vi "AutoRun.vi"(11 "AllControls In":T1) -> ()   [LabVIEW 2017]
uses:
  Ctrls/AllControls.ctl
  Ctrls/Data.ctl
  Ctrls/CSV_Data.ctl
  0516/X682 Chassis Connectivity Tester Program/Ctrls/682_cmd.ctl
  <vilib>/Utility/miscctls.llb/LVRowAndColumnTypeDef.ctl
  Ctrls/AlarmIndex.ctl
  Ctrls/PathChoose.ctl
  ComVIS/Files/Ini/WriteIniFiles_ByVarient.vi
  <vilib>/Utility/file.llb/Write Delimited Spreadsheet (string).vi
  <vilib>/regexp/Match Regular Expression.xnode
  <instrlib>/GPP/GPP.lvlib
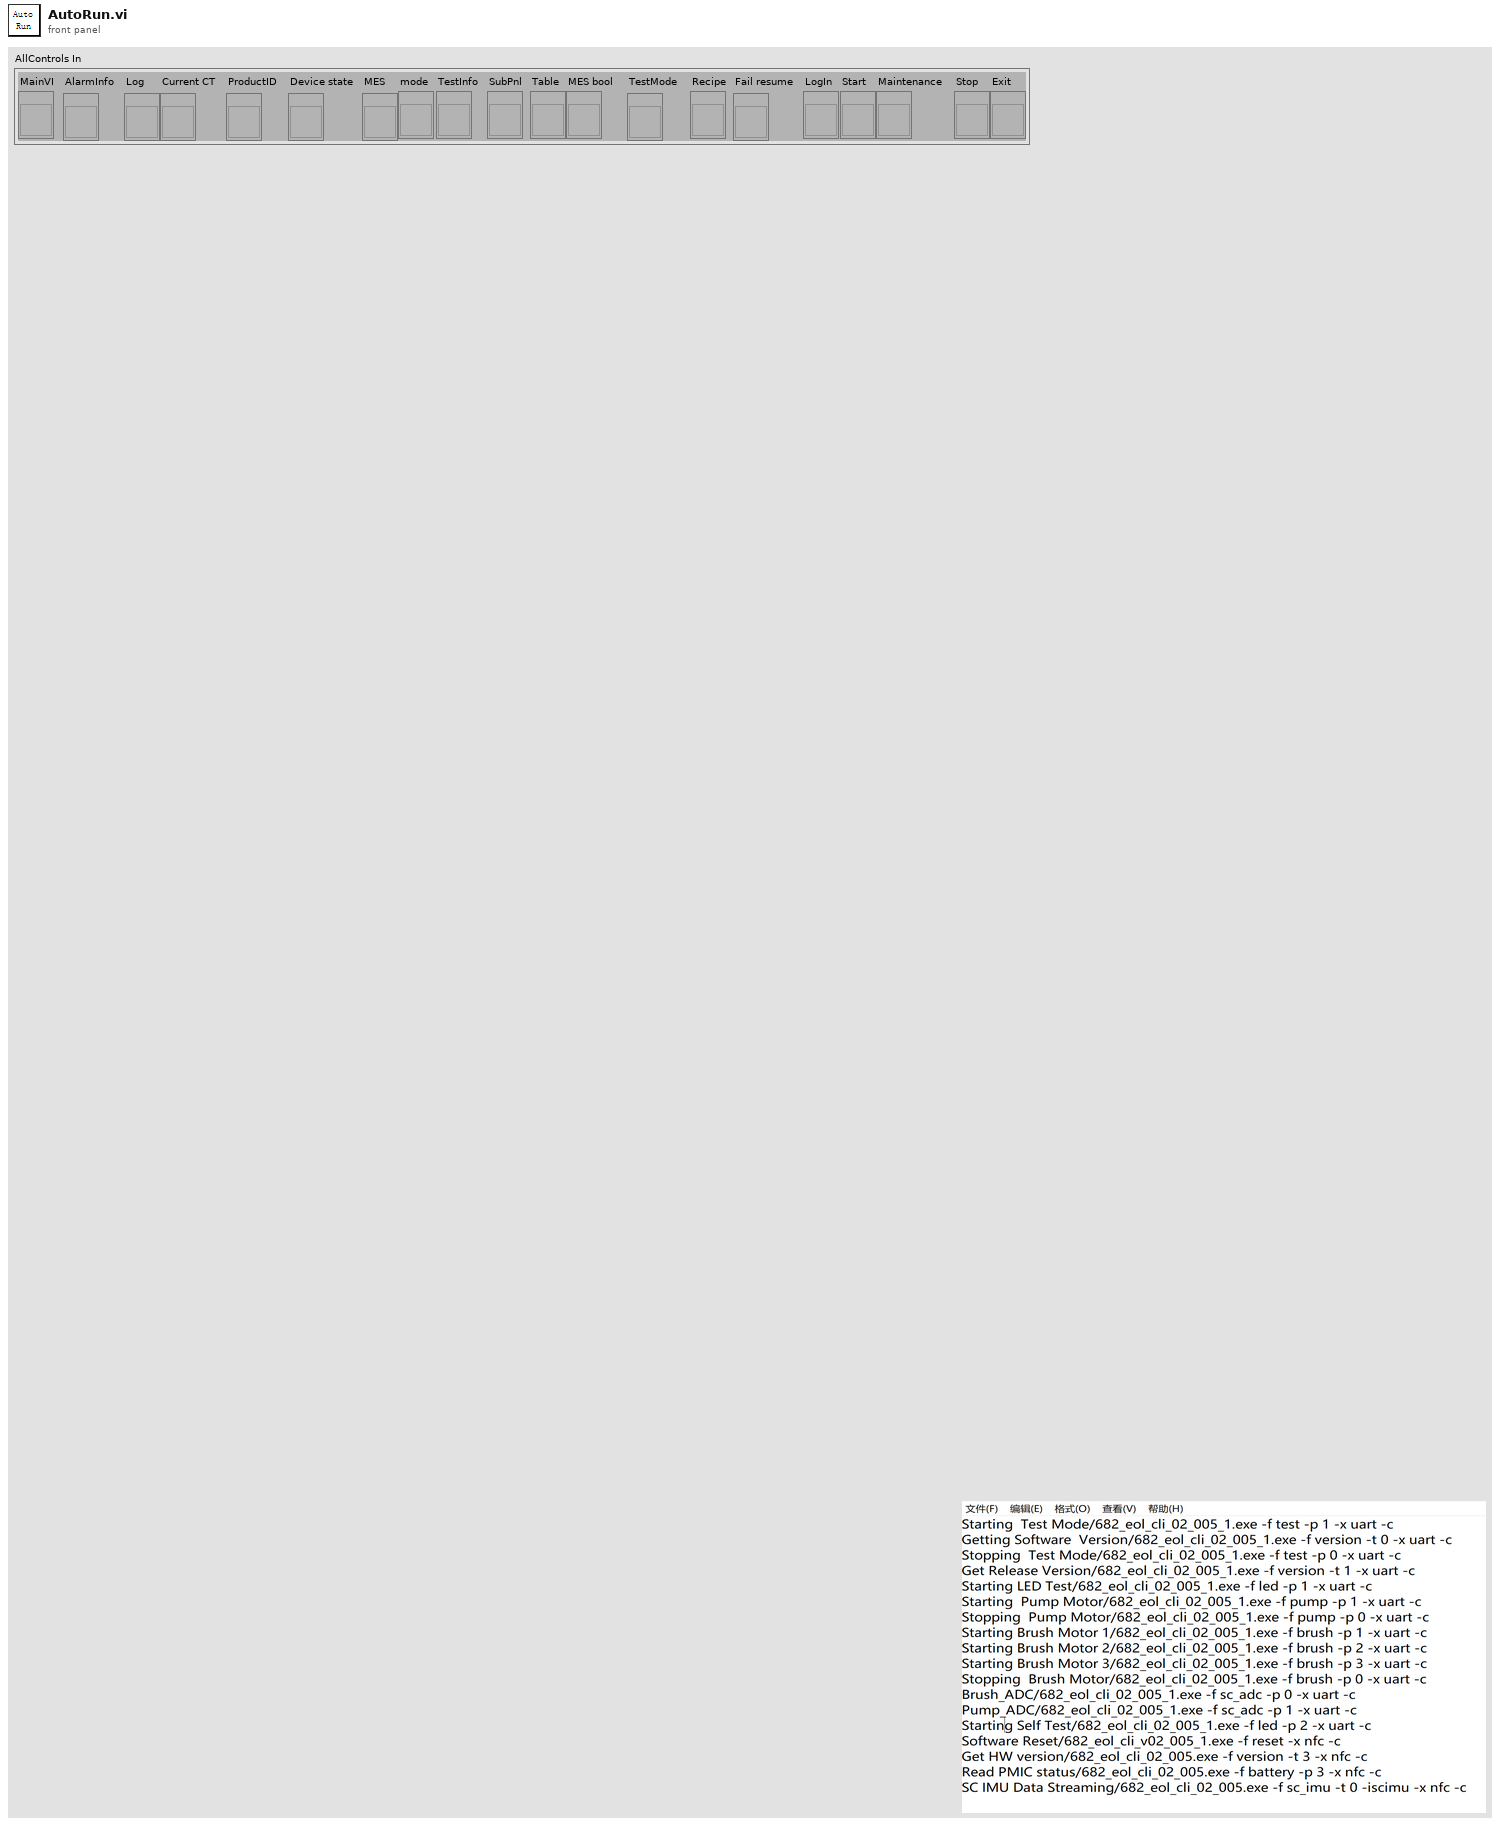
[diagram p1: front panel]
types:
  T1 = typedef "AllControls.ctl" = cluster{"MainVI":refnum<vi>, "AlarmInfo":refnum<vi>, "Log":refnum<vi>, "Current CT":refnum<vi>, "ProductID":refnum<vi>, "Device state":refnum<vi>, "MES":refnum<vi>, "mode":refnum<vi>, "TestInfo":refnum<vi>, "SubPnl":refnum<vi>, "Table":refnum<vi>, "MES bool":refnum<vi>, "TestMode":refnum<vi>, "Recipe":refnum<vi>, "Fail resume":refnum<vi>, "LogIn":refnum<vi>, "Start":refnum<vi>, "Maintenance":refnum<vi>, "Stop":refnum<vi>, "Exit":refnum<vi>}
  T2 = typedef "682_cmd.ctl" = cluster{"Brush_ADC.bat":string, "Get Release Version.bat":string, "Getting Software  Version.bat":string, "Pump_ADC.bat":string, "Starting  Pump Motor.bat":string, "Starting  Test Mode.bat":string, "Starting Brush Motor 1.bat":string, "Starting Brush Motor 2.bat":string, "Starting Brush Motor 3.bat":string, "Starting LED Test.bat":string, "Stopping  Brush Motor.bat":string, "Stopping  Pump Motor.bat":string, "Stopping  Test Mode.bat":string, "Starting Self Test.bat":string, "Software Reset.bat":string, "Get HW version.bat":string, "Read PMIC status.bat":string, "SC IMU Data Streaming.bat":string}
  T3 = typedef "CSV_Data.ctl" = cluster{"Initialisation":cluster{"LMT - Connect UUT (con COM)":string, "LMT - Software Version (rrel)":string, "LMT - Write SKU file (wskuc)":string, "LMT - SKU file name":string, "Connect UUT DDM":string, "Read DDM EOL Timestamp - Mode":string, "Read DDM EOL Timestamp - Timestamp":string, "Read DDM EOL Timestamp - Rig ID":string, "Read DDM EOL Timestamp - Passmark ID":string, "Read DDM EOL Timestamp - Passmark Rev":string, "Software Version before flashing":string, "Read Hardware Serial":string, "UUT DDM SN":string, "Compare DDM SN with MES SN":string, "Backup PCBA Calibration EEPROM Response - CAL":string, "Flash Firmware Version":string, "Check SW Version":string, "Read DDM SW Version after flashing":string, "Set SKU Config":string, "Ready Status":string, "Set Device Mode to EOL":string, "DDM Parameter - Voltage":string, "DDM Parameter - Current":string, "DDM Parameter - Power":string, "DDM Parameter - Speed":string, "DDM Parameter - Pressure":string, "Tester Parameter - Voltage":string, "Tester Parameter - Current":string, "Tester Parameter - Power":string, "Tester Parameter - Ambient Pressure":string, "Tester Parameter - Ambient Temperature":string, "Calculated Parameter - DDM Pressure Corrected":string, "Calculated Parameter - DDM Real Power":string, "Calculated Parameter - Delta V":string}, "BEMF_Calibration":cluster{"Calibration Result - eol_cold_bemf_temp":string, "DDM Ambient Temp":string, "Restriction Plate Diameter":string, "Calibration Result - eol_bemf_mp_cold_coef_a":string, "Calibration Result - eol_bemf_mp_cold_coef_b":string, "Calibration Result - eol_bemf_mp_cold_coef_c":string, "Calibration Result - eol_bemf_lsi_cold_ref_coeffs":string, "Get - Calibration Result - eol_bemf_lsi_speed":string, "Get - Calibration Result - eol_bemf_lsi_integral_0":string, "Calibration Result - eol_bemf_lsi_integral_1":string, "Get - Calibration Result - eol_bemf_lsi_integral_2":string, "Get - Calibration Result - eol_cold_bemf":string, "Get - Calibration Result - eol_cold_bemf_fisf":string, "Finalise Calibration":string, "Compare -Calibration Result - eol_cold_bemf":string, "Compare -Calibration Result - eol_cold_bemf_fisf":string}, "ECO":cluster{"Reset Power Tune":string, "Reset BEMF FISF Calibration":string, "Restriction Plate Diameter":string, "ECO - Stabilisation Time":string, "ECO - DDM Parameter - Voltage":string, "ECO - DDM Parameter - Current":string, "ECO - DDM Parameter - Power":string, "ECO - DDM Parameter - Measured Power":string, "ECO - DDM Parameter - Speed":string, "ECO - DDM Parameter - Pressure":string, "ECO - Tester Parameter - Voltage":string, "ECO - Tester Parameter - Current":string, "ECO - Tester Parameter - Power":string, "ECO - Tester Parameter - Ambient Pressure":string, "ECO - Tester Parameter - Ambient Temperature":string, "ECO - Tester Parameter - Ambient Humidity":string, "ECO - Calculated Parameter - DDM Pressure Corrected":string, "ECO - Calculated Parameter - DDM Real Power":string, "ECO - Calculated Parameter - Delta V":string, "ECO - Calculated Parameter - Flowrate":string, "ECO - Calculated Parameter - Airwatt":string, "ECO - Formula":string, "PT ECO - Power Tune Mode Status":string}, "BOOST":cluster{"Restriction Plate Diameter":string, "BOOST - Stabilisation Time":string, "BOOST - DDM Parameter - Voltage":string, "BOOST - DDM Parameter - Current":string, "BOOST - DDM Parameter - Power":string, "BOOST - DDM Parameter - Measured Power":string, "BOOST - DDM Parameter - Speed":string, "BOOST - DDM Parameter - Pressure":string, "BOOST - Tester Parameter - Voltage":string, "BOOST - Tester Parameter - Current":string, "BOOST - Tester Parameter - Power":string, "BOOST - Tester Parameter - Ambient Pressure":string, "BOOST - Tester Parameter - Ambient Temperature":string, "BOOST - Tester Parameter - Ambient Humidity":string, "BOOST - Calculated Parameter - DDM Pressure Corrected":string, "BOOST - Calculated Parameter - DDM Real Power":string, "BOOST - Calculated Parameter - Delta V":string, "BOOST - Calculated Parameter - Flowrate":string, "BOOST - Calculated Parameter - Airwatt":string, "BOOST - Get AM Presence":string, "Air Muscle Turn Off Status":string, "BOOST - Air Muscle Calculated Parameter - Airwatt B":string, "BOOST - Air Muscle Calculate Airwatt Delta":string, "PT BOOST - Power Tune Mode Status":string, "Finalise Calibration":string, "ECO - Get AW Calibration value":string, "BOOST - Get AW Calibration value":string}, "MAX":cluster{"Restriction Plate Diameter":string, "MAX - Stabilisation Time":string, "Get Average Delta Tmag (LSIdelta_FISFdelta_LSItmag_FISFtmag_IIRtmag)":string, "Get Average Delta Tmag FISF":string, "MAX - DDM Parameter - Voltage":string, "MAX - DDM Parameter - Current":string, "MAX - DDM Parameter - Power":string, "MAX - DDM Parameter - Measured Power":string, "MAX - DDM Parameter - Speed":string, "MAX - DDM Parameter - Pressure":string, "MAX - Tester Parameter - Voltage":string, "MAX - Tester Parameter - Current":string, "MAX - Tester Parameter - Power":string, "MAX - Tester Parameter - Ambient Pressure":string, "MAX - Tester Parameter - Ambient Temperature":string, "MAX - Tester Parameter - Ambient Humidity":string, "MAX - Calculated Parameter - DDM Pressure Corrected":string, "MAX - Calculated Parameter - DDM Real Power":string, "MAX - Calculated Parameter - Delta V":string, "MAX - Calculated Parameter - Flowrate":string, "MAX - Calculated Parameter - Airwatt":string, "MAX_FISF_Check_Average_Delta_Tmag":string, "MAX - FISF - BEMF Finetune Result":string, "MAX tune - Delta P1":string, "MAX tune - Calculated Parameter - Airwatt":string, "Calculate Delta Airwatts - MAX finetune - Delta P2":string, "MAX finetune - DDM Parameter - Voltage":string, "MAX finetune - DDM Parameter - Current":string, "MAX finetune - DDM Parameter - Power":string, "MAX finetune - DDM Parameter - Measured Power":string, "MAX finetune - DDM Parameter - Speed":string, "MAX finetune - DDM Parameter - Pressure":string, "MAX finetune - Tester Parameter - Voltage":string, "MAX finetune - Tester Parameter - Current":string, "MAX finetune - Tester Parameter - Power":string, "MAX finetune - Tester Parameter - Ambient Pressure":string, "MAX finetune - Tester Parameter - Ambient Temperature":string, "MAX finetune - Tester Parameter - Ambient Humidity":string, "MAX finetune - Calculated Parameter - DDM Pressure Corrected":string, "MAX finetune - Calculated Parameter - DDM Real Power":string, "MAX finetune - Calculated Parameter - Delta V":string, "MAX finetune - Calculated Parameter - Flowrate":string, "MAX finetune - Calculated Parameter - Airwatt":string, "Check Derate Result":string, "Delta Tmag FISF":string, "Get Hot BEMF Result":string, "Calculate delta Pressure":string, "Finalise Calibration":string, "Calculate & Check Delta BEMF":string, "Delta P Airwatts Value":string}, "LL":cluster{"DDM Ambient Temp":string, "Restriction Plate Diameter":string, "LL - DDM Parameter - Voltage":string, "LL - DDM Parameter - Current":string, "LL - DDM Parameter - Power":string, "LL - DDM Parameter - Measured Power":string, "LL - DDM Parameter - Speed":string, "LL - DDM Parameter - Pressure":string, "LL - Tester Parameter - Voltage":string, "LL - Tester Parameter - Current":string, "LL - Tester Parameter - Power":string, "LL - DDM Real Power":string, "LL - Calibrate Task Detect LL":string}, "HL":cluster{"HL - DDM Parameter - Voltage":string, "HL - DDM Parameter - Current":string, "HL - DDM Parameter - Power":string, "HL - DDM Parameter - Measured Power":string, "HL - DDM Parameter - Speed":string, "HL - DDM Parameter - Pressure":string, "HL - Tester Parameter - Voltage":string, "HL - Tester Parameter - Current":string, "HL - Tester Parameter - Power":string, "HL - DDM Real Power":string, "HL - Calibrate Task Detect HL":string}, "LH":cluster{"Restriction Plate Diameter":string, "LH - DDM Parameter - Voltage":string, "LH - DDM Parameter - Current":string, "LH - DDM Parameter - Power":string, "LH - DDM Parameter - Measured Power":string, "LH - DDM Parameter - Speed":string, "LH - DDM Parameter - Pressure":string, "LH - Tester Parameter - Voltage":string, "LH - Tester Parameter - Current":string, "LH - Tester Parameter - Power":string, "LH - DDM Real Power":string, "LH - Calibrate Task Detect LH":string}, "HH":cluster{"HH - DDM Parameter - Voltage":string, "HH - DDM Parameter - Current":string, "HH - DDM Parameter - Power":string, "HH - DDM Parameter - Measured Power":string, "HH - DDM Parameter - Speed":string, "HH - DDM Parameter - Pressure":string, "HH - Tester Parameter - Voltage":string, "HH - Tester Parameter - Current":string, "HH - Tester Parameter - Power":string, "HH - DDM Real Power":string, "HH - Calibrate Task Detect HH":string}, "Inlet Blockage Calibration":cluster{"Inlet Blockage Calibration - DDM Parameter - Voltage":string, "Inlet Blockage Calibration - DDM Parameter - Current":string, "Inlet Blockage Calibration - DDM Parameter - Power":string, "Inlet Blockage Calibration - DDM Parameter - Measured Power":string, "Inlet Blockage Calibration - DDM Parameter - Speed":string, "Inlet Blockage Calibration - DDM Parameter - Pressure":string, "Inlet Blockage Calibration - Tester Parameter - Voltage":string, "Inlet Blockage Calibration - Tester Parameter - Current":string, "Inlet Blockage Calibration - Tester Parameter - Power":string, "Inlet Blockage Calibration - DDM Real Power":string, "Calibration Inlet Blockage_E":string, "Finalise Calibration":string, "Get Task Detect LL":string, "Get Task Detect HL":string, "Get Task Detect LH":string, "Get Task Detect HH":string, "Calibration Inlet Blockage":string, "Calibration eol cold bemf temp":string}, "GOOD":cluster{"GOOD UNIT - Clear EEPROM Error Log":string, "GOOD UNIT - Write Product Timestamp - Mode":string, "GOOD UNIT - Write Product Timestamp - Timestamp":string, "GOOD UNIT - Write Product Timestamp - Rig ID":string, "GOOD UNIT - Write Product Timestamp - Passmark ID":string, "GOOD UNIT - Write Product Timestamp - Passmark Rev":string, "GOOD UNIT - Set Device Mode to PROD":string, "GOOD UNIT - Backup PCBA Calibration EEPROM Response":string, "GOOD UNIT - Check Security Bit":string, "GOOD UNIT - Set Calibration Lock":string, "GOOD UNIT - Get_Calibration_Lock":string, "GOOD UNIT - Disconnect UUT":string}, "NG":cluster{"NG UNIT - Read NVM Error":string, "NG UNIT - Set Device Mode to FCT":string, "NG UNIT - Backup PCBA Calibration EEPROM Response - CAL":string, "NG UNIT - Backup PCBA Calibration EEPROM Response - ERROR":string, "NG UNIT - Backup PCBA Calibration EEPROM Response - USAGE":string, "NG UNIT - Disconnect UUT":string}, "SN":string, "Table":string[][], "Count":cluster{"Total":i32, "OK":i32, "NG":i32, "Yield":dbl}, "Start Time":timestamp, "daemon reference":refnum<k5>, "CT":dbl, "Config":string[][], "OK/NG":bool, "Station ID":string, "MES DDM SN":string, "MES PCBA SN":string, "Retest":string, "Lux":string, "Initialisation_Status":cluster{"LMT - Connect UUT (con COM)":string, "LMT - Software Version (rrel)":string, "LMT - Write SKU file (wskuc)":string, "LMT - SKU file name":string, "Connect UUT DDM":string, "Read DDM EOL Timestamp - Mode":string, "Read DDM EOL Timestamp - Timestamp":string, "Read DDM EOL Timestamp - Rig ID":string, "Read DDM EOL Timestamp - Passmark ID":string, "Read DDM EOL Timestamp - Passmark Rev":string, "Software Version before flashing":string, "Read Hardware Serial":string, "UUT DDM SN":string, "Compare DDM SN with MES SN":string, "Backup PCBA Calibration EEPROM Response - CAL":string, "Flash Firmware Version":string, "Check SW Version":string, "Read DDM SW Version after flashing":string, "Set SKU Config":string, "Ready Status":string, "Set Device Mode to EOL":string, "DDM Parameter - Voltage":string, "DDM Parameter - Current":string, "DDM Parameter - Power":string, "DDM Parameter - Speed":string, "DDM Parameter - Pressure":string, "Tester Parameter - Voltage":string, "Tester Parameter - Current":string, "Tester Parameter - Power":string, "Tester Parameter - Ambient Pressure":string, "Tester Parameter - Ambient Temperature":string, "Calculated Parameter - DDM Pressure Corrected":string, "Calculated Parameter - DDM Real Power":string, "Calculated Parameter - Delta V":string}, "BEMF_Calibration_Status":cluster{"Calibration Result - eol_cold_bemf_temp":string, "DDM Ambient Temp":string, "Restriction Plate Diameter":string, "Calibration Result - eol_bemf_mp_cold_coef_a":string, "Calibration Result - eol_bemf_mp_cold_coef_b":string, "Calibration Result - eol_bemf_mp_cold_coef_c":string, "Calibration Result - eol_bemf_lsi_cold_ref_coeffs":string, "Get - Calibration Result - eol_bemf_lsi_speed":string, "Get - Calibration Result - eol_bemf_lsi_integral_0":string, "Calibration Result - eol_bemf_lsi_integral_1":string, "Get - Calibration Result - eol_bemf_lsi_integral_2":string, "Get - Calibration Result - eol_cold_bemf":string, "Get - Calibration Result - eol_cold_bemf_fisf":string, "Finalise Calibration":string, "Compare -Calibration Result - eol_cold_bemf":string, "Compare -Calibration Result - eol_cold_bemf_fisf":string}, "ECO_Status":cluster{"Reset Power Tune":string, "Reset BEMF FISF Calibration":string, "Restriction Plate Diameter":string, "ECO - Stabilisation Time":string, "ECO - DDM Parameter - Voltage":string, "ECO - DDM Parameter - Current":string, "ECO - DDM Parameter - Power":string, "ECO - DDM Parameter - Measured Power":string, "ECO - DDM Parameter - Speed":string, "ECO - DDM Parameter - Pressure":string, "ECO - Tester Parameter - Voltage":string, "ECO - Tester Parameter - Current":string, "ECO - Tester Parameter - Power":string, "ECO - Tester Parameter - Ambient Pressure":string, "ECO - Tester Parameter - Ambient Temperature":string, "ECO - Tester Parameter - Ambient Humidity":string, "ECO - Calculated Parameter - DDM Pressure Corrected":string, "ECO - Calculated Parameter - DDM Real Power":string, "ECO - Calculated Parameter - Delta V":string, "ECO - Calculated Parameter - Flowrate":string, "ECO - Calculated Parameter - Airwatt":string, "ECO - Formula":string, "PT ECO - Power Tune Mode Status":string}, "BOOST_Status":cluster{"Restriction Plate Diameter":string, "BOOST - Stabilisation Time":string, "BOOST - DDM Parameter - Voltage":string, "BOOST - DDM Parameter - Current":string, "BOOST - DDM Parameter - Power":string, "BOOST - DDM Parameter - Measured Power":string, "BOOST - DDM Parameter - Speed":string, "BOOST - DDM Parameter - Pressure":string, "BOOST - Tester Parameter - Voltage":string, "BOOST - Tester Parameter - Current":string, "BOOST - Tester Parameter - Power":string, "BOOST - Tester Parameter - Ambient Pressure":string, "BOOST - Tester Parameter - Ambient Temperature":string, "BOOST - Tester Parameter - Ambient Humidity":string, "BOOST - Calculated Parameter - DDM Pressure Corrected":string, "BOOST - Calculated Parameter - DDM Real Power":string, "BOOST - Calculated Parameter - Delta V":string, "BOOST - Calculated Parameter - Flowrate":string, "BOOST - Calculated Parameter - Airwatt":string, "BOOST - Get AM Presence":string, "Air Muscle Turn Off Status":string, "BOOST - Air Muscle Calculated Parameter - Airwatt B":string, "BOOST - Air Muscle Calculate Airwatt Delta":string, "PT BOOST - Power Tune Mode Status":string, "Finalise Calibration":string, "ECO - Get AW Calibration value":string, "BOOST - Get AW Calibration value":string}, "MAX_Status":cluster{"Restriction Plate Diameter":string, "MAX - Stabilisation Time":string, "Get Average Delta Tmag (LSIdelta_FISFdelta_LSItmag_FISFtmag_IIRtmag)":string, "Get Average Delta Tmag FISF":string, "MAX - DDM Parameter - Voltage":string, "MAX - DDM Parameter - Current":string, "MAX - DDM Parameter - Power":string, "MAX - DDM Parameter - Measured Power":string, "MAX - DDM Parameter - Speed":string, "MAX - DDM Parameter - Pressure":string, "MAX - Tester Parameter - Voltage":string, "MAX - Tester Parameter - Current":string, "MAX - Tester Parameter - Power":string, "MAX - Tester Parameter - Ambient Pressure":string, "MAX - Tester Parameter - Ambient Temperature":string, "MAX - Tester Parameter - Ambient Humidity":string, "MAX - Calculated Parameter - DDM Pressure Corrected":string, "MAX - Calculated Parameter - DDM Real Power":string, "MAX - Calculated Parameter - Delta V":string, "MAX - Calculated Parameter - Flowrate":string, "MAX - Calculated Parameter - Airwatt":string, "MAX_FISF_Check_Average_Delta_Tmag":string, "MAX - FISF - BEMF Finetune Result":string, "MAX tune - Delta P1":string, "MAX tune - Calculated Parameter - Airwatt":string, "Calculate Delta Airwatts - MAX finetune - Delta P2":string, "MAX finetune - DDM Parameter - Voltage":string, "MAX finetune - DDM Parameter - Current":string, "MAX finetune - DDM Parameter - Power":string, "MAX finetune - DDM Parameter - Measured Power":string, "MAX finetune - DDM Parameter - Speed":string, "MAX finetune - DDM Parameter - Pressure":string, "MAX finetune - Tester Parameter - Voltage":string, "MAX finetune - Tester Parameter - Current":string, "MAX finetune - Tester Parameter - Power":string, "MAX finetune - Tester Parameter - Ambient Pressure":string, "MAX finetune - Tester Parameter - Ambient Temperature":string, "MAX finetune - Tester Parameter - Ambient Humidity":string, "MAX finetune - Calculated Parameter - DDM Pressure Corrected":string, "MAX finetune - Calculated Parameter - DDM Real Power":string, "MAX finetune - Calculated Parameter - Delta V":string, "MAX finetune - Calculated Parameter - Flowrate":string, "MAX finetune - Calculated Parameter - Airwatt":string, "Check Derate Result":string, "Delta Tmag FISF":string, "Get Hot BEMF Result":string, "Calculate delta Pressure":string, "Finalise Calibration":string, "Calculate & Check Delta BEMF":string, "Delta P Airwatts Value":string}, "LL_Status":cluster{"DDM Ambient Temp":string, "Restriction Plate Diameter":string, "LL - DDM Parameter - Voltage":string, "LL - DDM Parameter - Current":string, "LL - DDM Parameter - Power":string, "LL - DDM Parameter - Measured Power":string, "LL - DDM Parameter - Speed":string, "LL - DDM Parameter - Pressure":string, "LL - Tester Parameter - Voltage":string, "LL - Tester Parameter - Current":string, "LL - Tester Parameter - Power":string, "LL - DDM Real Power":string, "LL - Calibrate Task Detect LL":string}, "HL_Status":cluster{"HL - DDM Parameter - Voltage":string, "HL - DDM Parameter - Current":string, "HL - DDM Parameter - Power":string, "HL - DDM Parameter - Measured Power":string, "HL - DDM Parameter - Speed":string, "HL - DDM Parameter - Pressure":string, "HL - Tester Parameter - Voltage":string, "HL - Tester Parameter - Current":string, "HL - Tester Parameter - Power":string, "HL - DDM Real Power":string, "HL - Calibrate Task Detect HL":string}, "LH_Status":cluster{"Restriction Plate Diameter":string, "LH - DDM Parameter - Voltage":string, "LH - DDM Parameter - Current":string, "LH - DDM Parameter - Power":string, "LH - DDM Parameter - Measured Power":string, "LH - DDM Parameter - Speed":string, "LH - DDM Parameter - Pressure":string, "LH - Tester Parameter - Voltage":string, "LH - Tester Parameter - Current":string, "LH - Tester Parameter - Power":string, "LH - DDM Real Power":string, "LH - Calibrate Task Detect LH":string}, "HH_Status":cluster{"HH - DDM Parameter - Voltage":string, "HH - DDM Parameter - Current":string, "HH - DDM Parameter - Power":string, "HH - DDM Parameter - Measured Power":string, "HH - DDM Parameter - Speed":string, "HH - DDM Parameter - Pressure":string, "HH - Tester Parameter - Voltage":string, "HH - Tester Parameter - Current":string, "HH - Tester Parameter - Power":string, "HH - DDM Real Power":string, "HH - Calibrate Task Detect HH":string}, "Inlet Blockage Calibration_Status":cluster{"Inlet Blockage Calibration - DDM Parameter - Voltage":string, "Inlet Blockage Calibration - DDM Parameter - Current":string, "Inlet Blockage Calibration - DDM Parameter - Power":string, "Inlet Blockage Calibration - DDM Parameter - Measured Power":string, "Inlet Blockage Calibration - DDM Parameter - Speed":string, "Inlet Blockage Calibration - DDM Parameter - Pressure":string, "Inlet Blockage Calibration - Tester Parameter - Voltage":string, "Inlet Blockage Calibration - Tester Parameter - Current":string, "Inlet Blockage Calibration - Tester Parameter - Power":string, "Inlet Blockage Calibration - DDM Real Power":string, "Calibration Inlet Blockage_E":string, "Finalise Calibration":string, "Get Task Detect LL":string, "Get Task Detect HL":string, "Get Task Detect LH":string, "Get Task Detect HH":string, "Calibration Inlet Blockage":string, "Calibration eol cold bemf temp":string}, "GOOD_Status":cluster{"GOOD UNIT - Clear EEPROM Error Log":string, "GOOD UNIT - Write Product Timestamp - Mode":string, "GOOD UNIT - Write Product Timestamp - Timestamp":string, "GOOD UNIT - Write Product Timestamp - Rig ID":string, "GOOD UNIT - Write Product Timestamp - Passmark ID":string, "GOOD UNIT - Write Product Timestamp - Passmark Rev":string, "GOOD UNIT - Set Device Mode to PROD":string, "GOOD UNIT - Backup PCBA Calibration EEPROM Response":string, "GOOD UNIT - Check Security Bit":string, "GOOD UNIT - Set Calibration Lock":string, "GOOD UNIT - Get_Calibration_Lock":string, "GOOD UNIT - Disconnect UUT":string}, "NG_Status":cluster{"NG UNIT - Read NVM Error":string, "NG UNIT - Set Device Mode to FCT":string, "NG UNIT - Backup PCBA Calibration EEPROM Response - CAL":string, "NG UNIT - Backup PCBA Calibration EEPROM Response - ERROR":string, "NG UNIT - Backup PCBA Calibration EEPROM Response - USAGE":string, "NG UNIT - Disconnect UUT":string}, "SKU":string, "Plate_Diameter":string, "Alarm":string}
  T4 = typedef "Data.ctl" = cluster{"Initialisation":cluster{"DDM_Parameter":dbl[], "DDM_Parameter_status":bool[], "Get_Tester_Parameter":dbl[], "Get_Tester_Parameter_status":bool[], "Cal_Tester_Parameter":dbl[], "Cal_Tester_Parameter_status":bool[], "sw_version_before_status":bool, "sw_version_after_status":bool, "Set_SKU_Config_With_LMT_status":bool, "FCT_timestamp_status":bool, "LMT_Connect_to_UUT_status":bool}, "BEMF_Calibration":cluster{"Read_ambient_temperature":dbl, "Calibration_Vaule":dbl[], "Calibration_Vaule _B":dbl[], "Calibration_Vaule_status":bool[], "Calibration_Vaule_B_status":bool[]}, "ECO":cluster{"DDM_Parameter":dbl[], "DDM_Parameter_status":bool[], "Get_Tester_Parameter":dbl[], "Get_Tester_Parameter_status":bool[], "Cal_Tester_Parameter":dbl[], "Cal_Tester_Parameter_status":bool[], "DDM_Parameter_after_power_tune":dbl[], "Get_Tester_Parameter_after_power_tune":dbl[], "Cal_Tester_Parameter_after_power_tune":dbl[], "Cal_Tester_Parameter_after_power_tune_status":bool[], "Delta_P":dbl}, "BOOST":cluster{"DDM_Parameter":dbl[], "DDM_Parameter_status":bool[], "Get_Tester_Parameter":dbl[], "Get_Tester_Parameter_status":bool[], "Cal_Tester_Parameter":dbl[], "Cal_Tester_Parameter_status":bool[], "DDM_Parameter_after_power_tune":dbl[], "Get_Tester_Parameter_after_power_tune":dbl[], "Cal_Tester_Parameter_after_power_tune":dbl[], "Cal_Tester_Parameter_after_power_tune_status":bool[], "airwatts_am_off":dbl, "AW_Delta_(AM_on_and_off)":dbl, "AW_Delta_(AM_on_and_off)_Status":bool, "Delta_P":dbl}, "MAX":cluster{"Average_Tmag_Data":cluster{"LSI Delta in degC":dbl, "FISF Delta in degc":dbl, "LSI Tmag in degC":dbl, "Fisf Tmag in degC":dbl, "IIR Tmag in degC":dbl}, "DDM_Parameter":dbl[], "DDM_Parameter_status":bool[], "Get_Tester_Parameter":dbl[], "Get_Tester_Parameter_status":bool[], "Cal_Tester_Parameter":dbl[], "BEMF_Finetune":cluster{"eol_bemf_mp_cold_coef_c":dbl, "eol_cold_bemf_fisf_offset":dbl}, "AW_Tune":cluster{"delta_P1":dbl, "delta_P_Setting":dbl}, "DDM_Parameter_after_Airwatts_Tune":dbl[], "Get_Tester_Parameter_after_Airwatts_Tune":dbl[], "Cal_Tester_Parameter_after_Airwatts_Tune":dbl[], "DDM_Parameter_after_Airwatts_Finetune":dbl[], "Get_Tester_Parameter_after_Airwatts_Finetune":dbl[], "Cal_Tester_Parameter_after_Airwatts_Finetune":dbl[], "AW_Finetune":cluster{"delta_P2":dbl, "delta_P_Setting":dbl}, "Delta_Tmag_after_tune":cluster{"LSI Delta in degC":dbl, "FISF Delta in degc":dbl, "LSI Tmag in degC":dbl, "Fisf Tmag in degC":dbl, "IIR Tmag in degC":dbl}, "Hot Bemf in mV":dbl, "DDM_Pressure":dbl, "Delta_Pressure":dbl, " Cold Bemf in mV":dbl, " delta Bemf":dbl, " delta p":dbl, "Delta_Pressure_status":bool, " delta Bemf_status":bool, "LSI Delta in degC_status":bool, "FISF Delta in degc_status":bool, "Max_check_derate_status_status":bool, "Average_All_data":dbl[][], "Average_Tmag_Data_status":bool[], "Average_Tmag_Data_after_tune_status":bool[], "Cal_Tester_Parameter_status":bool[], "Cal_Tester_Parameter_status_after_Airwatts_Tune":bool[], "Cal_Tester_Parameter_status_after_Airwatts_FineTune":bool[]}, "Task_Detect_Calib":cluster{"LL":cluster{"DDM_Parameter":dbl[], "DDM_Parameter_status":bool[], "Get_Tester_Parameter":dbl[], "Get_Tester_Parameter_status":bool[], "Set_task_detect_A":dbl, "Set_task_detect_A_Status":bool}, "HL":cluster{"DDM_Parameter":dbl[], "DDM_Parameter_status":bool[], "Get_Tester_Parameter":dbl[], "Get_Tester_Parameter_status":bool[], "Set_task_detect_B":dbl, "Set_task_detect_B_Status":bool}, "LH":cluster{"DDM_Parameter":dbl[], "DDM_Parameter_status":bool[], "Get_Tester_Parameter":dbl[], "Get_Tester_Parameter_status":bool[], "Set_task_detect_C":dbl, "Set_task_detect_C_Status":bool}, "HH":cluster{"DDM_Parameter":dbl[], "DDM_Parameter_status":bool[], "Get_Tester_Parameter":dbl[], "Get_Tester_Parameter_status":bool[], "Set_task_detect_D":dbl, "Read_and_check_calibration_Status":bool[], "Set_task_detect_D_Status":bool}, "Get_eol_inlet_blockage_E":dbl, "Calib_vaule":cluster{"Get_task_detect_LL":dbl, "Get_task_detect_HL":dbl, "Get_task_detect_LH":dbl, "Get_task_detect_HH":dbl, "eol_inlet_blockage":dbl, "eol_code_bemf_temp":dbl}, "calibrated temp":dbl, "Inlet_Blockage_Calibration":cluster{"DDM_Parameter":dbl[], "DDM_Parameter_status":bool[], "Get_Tester_Parameter":dbl[], "Get_Tester_Parameter_status":bool[]}, "Get_eol_inlet_blockage_E_Status":bool}, "good":cluster{"Write_Product_TS":cluster{"TIMESTAMP":i64, "RIG_ID":i64, "PASSMARK_ID":i64, "PASSMARK_REV":i64}, "Read_Product_TS":cluster{"TIMESTAMP":i64, "RIG_ID":i64, "PASSMARK_ID":i64, "PASSMARK_REV":i64}, "Good_Check_Secuity_Bit_Stauts":bool}}
  T5 = typedef "amc_Message Queue.ctl" = refnum<queue>
  T6 = typedef "TesterInfo.ctl" = cluster{"Station Name":string, "Station Code":string, "ES NO.":string, "Tester ID":string, "PassMark Revision":string, "Rig ID":string, "Deamon_vision":string, "Project Name":string, "FFTesterPath":path, "Enable_User":bool, "Mode":enum16{"682"}, "MES":bool}
  T7 = cluster{"Total":i32, "OK":i32, "NG":i32, "Yield":dbl}
  T8 = typedef "LVRowAndColumnTypeDef.ctl" = cluster{"Row":i32, "Column":i32}
  T9 = enum8{"Enabled", "Disabled", "Disabled and Grayed Out"}
  T10 = typedef "AlarmIndex.ctl" = enum16{"E-Stop", "Safety light grid", "UUT Sealing Cylinder HomePoint", "UUT Sealing Cylinder WorkPoint", "Orifice fixed Cylinder L HomePoint", "Orifice fixed Cylinder L WorkPoint", "Orifice fixed Cylinder R HomePoint", "Orifice fixed Cylinder R WorkPoint", "UUT Cylinder HomePoint", "UUT Cylinder WorkPoint", "Carrier fixed Cylinder L HomePoint", "Carrier fixed Cylinder L WorkPoint", "Carrier fixed Cylinder R HomePoint", "Carrier fixed Cylinder R WorkPoint", "Probe Cylinder HomePoint", "Probe Cylinder WorkPoint", "Motor Error", "Test Error"}
  T11 = typedef "PathChoose.ctl" = enum16{"OperatorLog", "AutoRunLog", "AlmLog", "TestData", "AllTestData", "backup_nvm", "backup_before_flashing"}
  T12 = typedef "HD Config.ctl" = cluster{" PC":cluster{"PC Address":u8[], "PC Port":i32}, "FCO":cluster{"COM":refnum<visa-resource-name>, "Baudrate":u32}, "DC Power ":cluster{"COM":refnum<visa-resource-name>, "Baudrate":u32}, "PW3336":cluster{"COM":refnum<visa-resource-name>, "Baudrate":u32}, "Lefoo":cluster{"COM":refnum<visa-resource-name>, "Baudrate":u32}, "Tempt&Hum":cluster{"COM":refnum<visa-resource-name>, "Baudrate":u32}, "DIPC":cluster{"COM":refnum<visa-resource-name>}, "Daemon":cluster{"IP Address":string, "Port":u16, "Retry":u16}, "URAT":cluster{"COM":refnum<visa-resource-name>, "Baudrate":u32}, "Fail_resume_mode":bool, "GRR":bool}
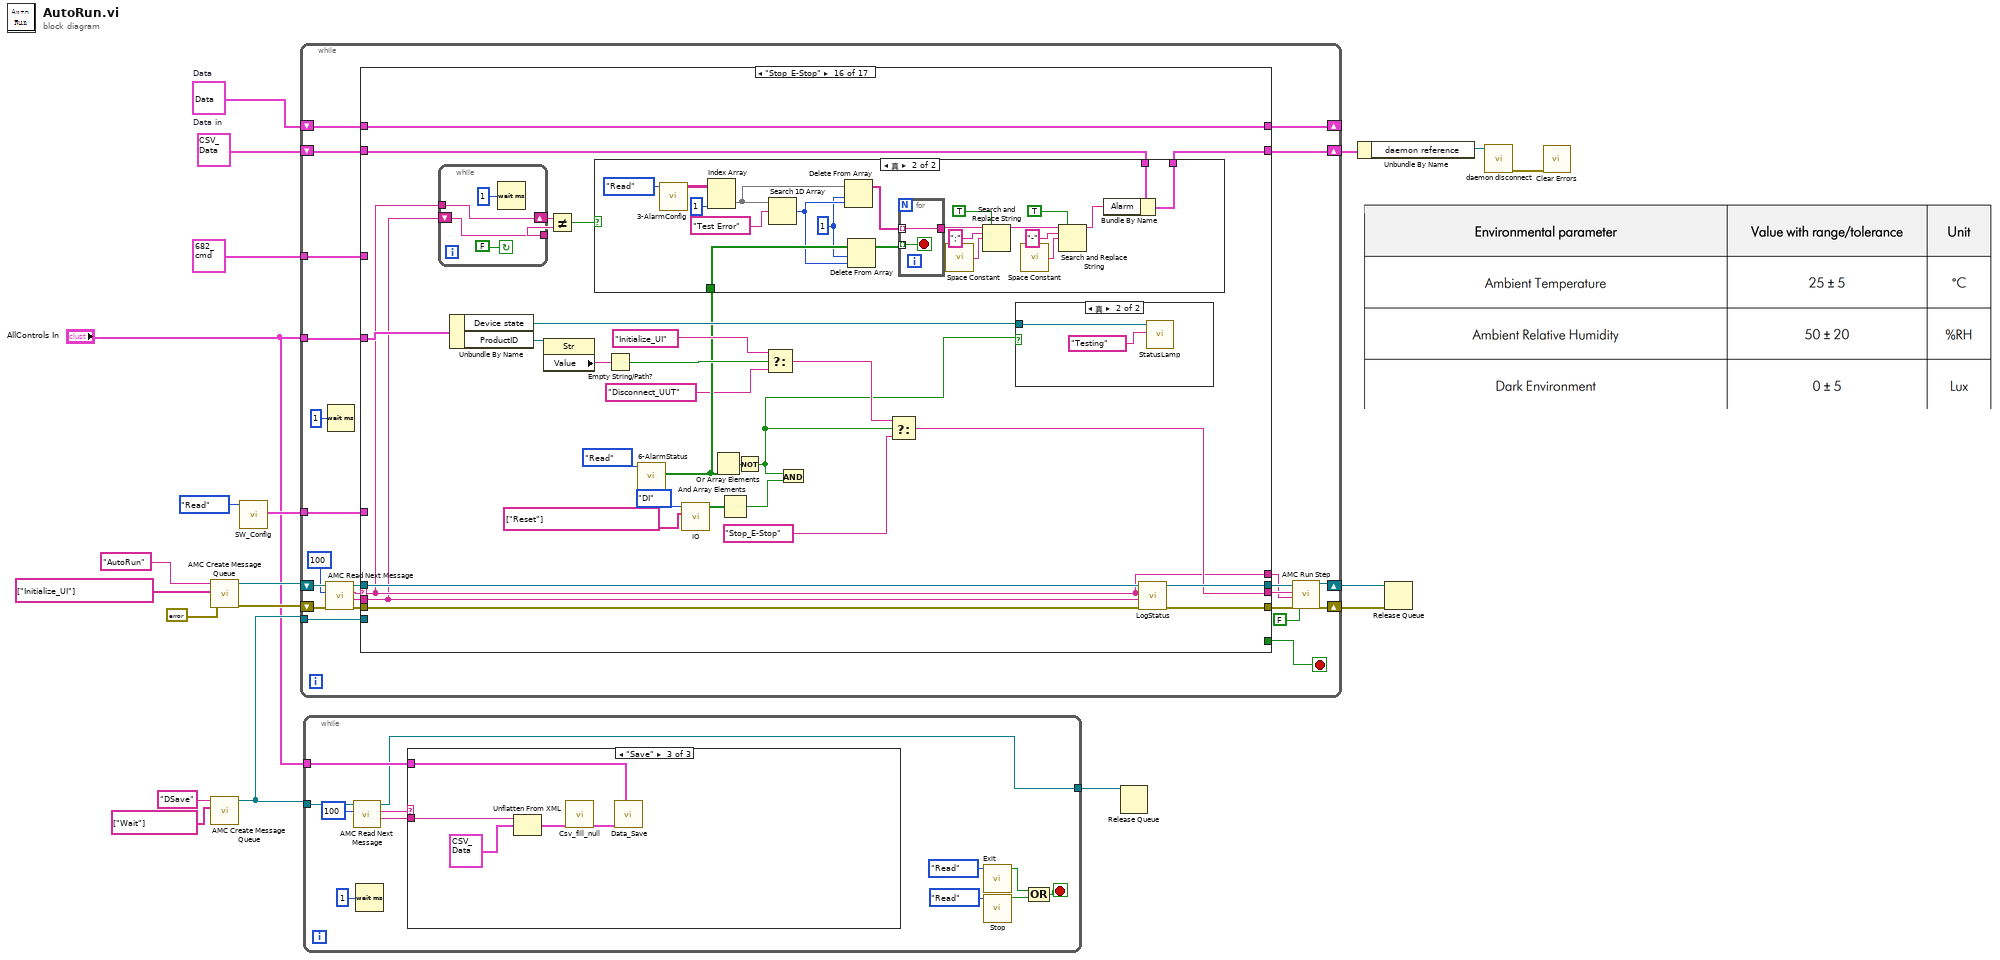
[diagram p0: block diagram]
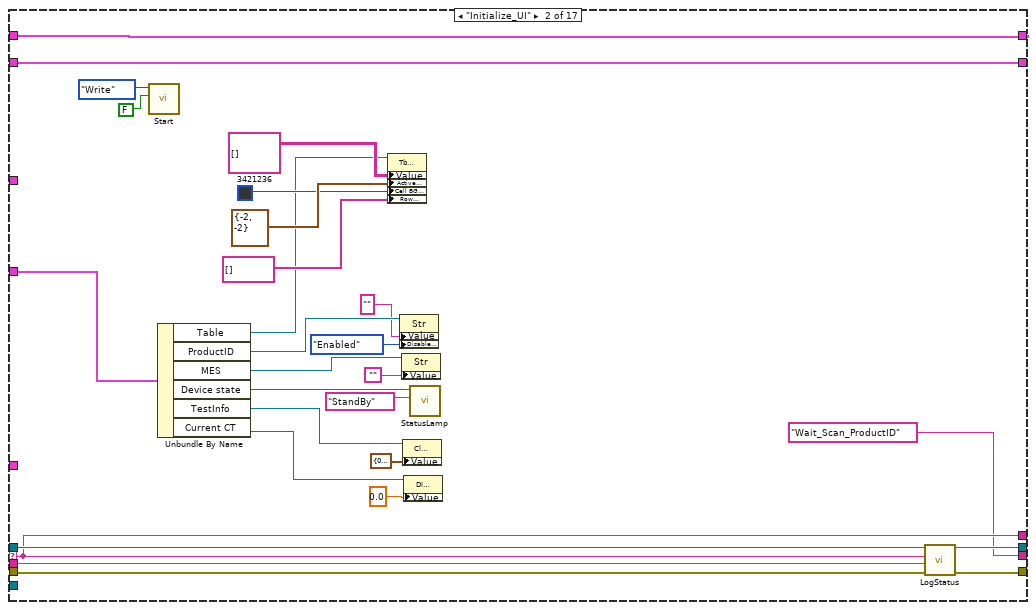
[diagram p5: hidden frame]
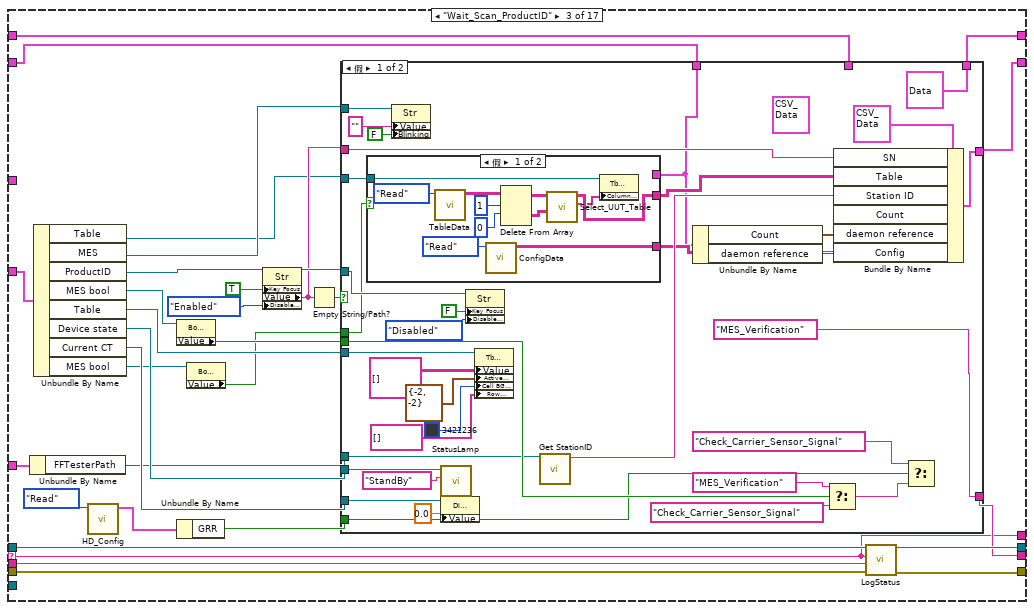
[diagram p6: hidden frame]
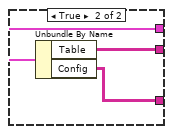
[diagram p7: hidden frame]
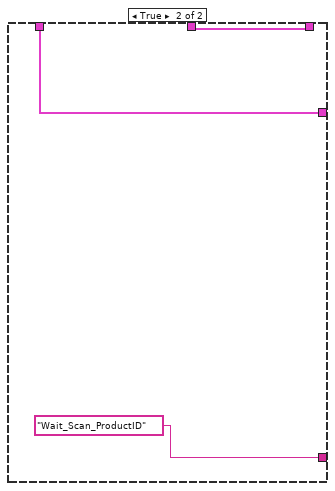
[diagram p8: hidden frame]
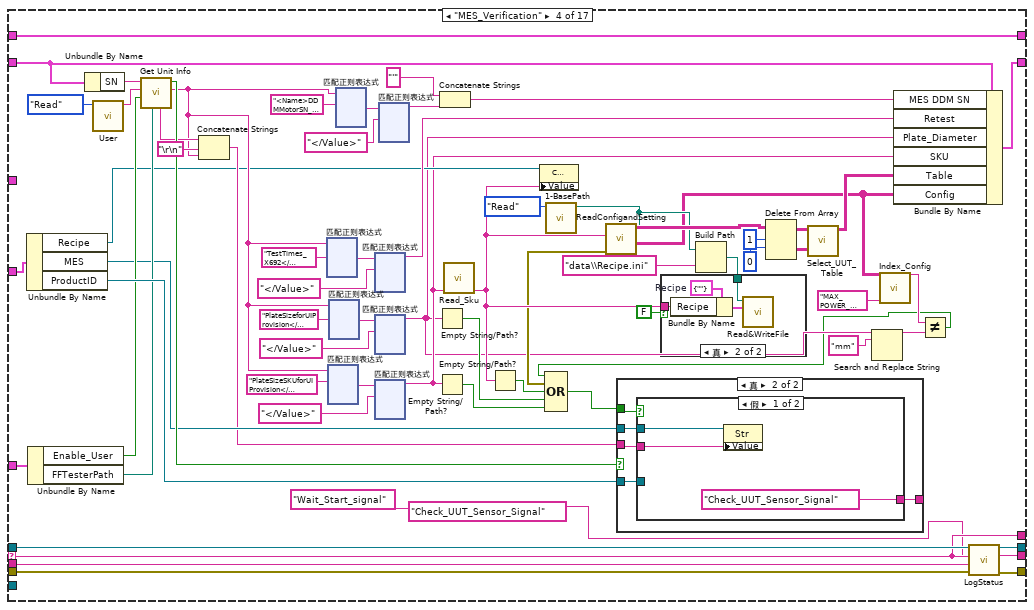
[diagram p9: hidden frame]
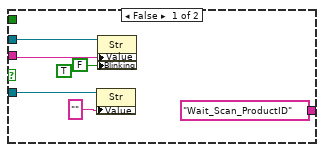
[diagram p11: hidden frame]
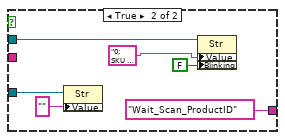
[diagram p12: hidden frame]
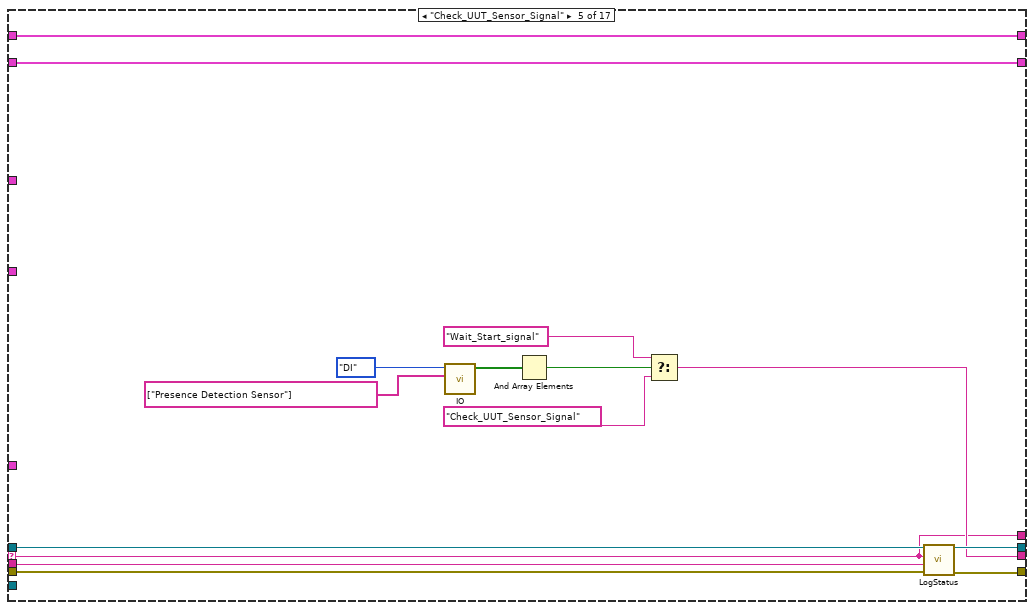
[diagram p13: hidden frame]
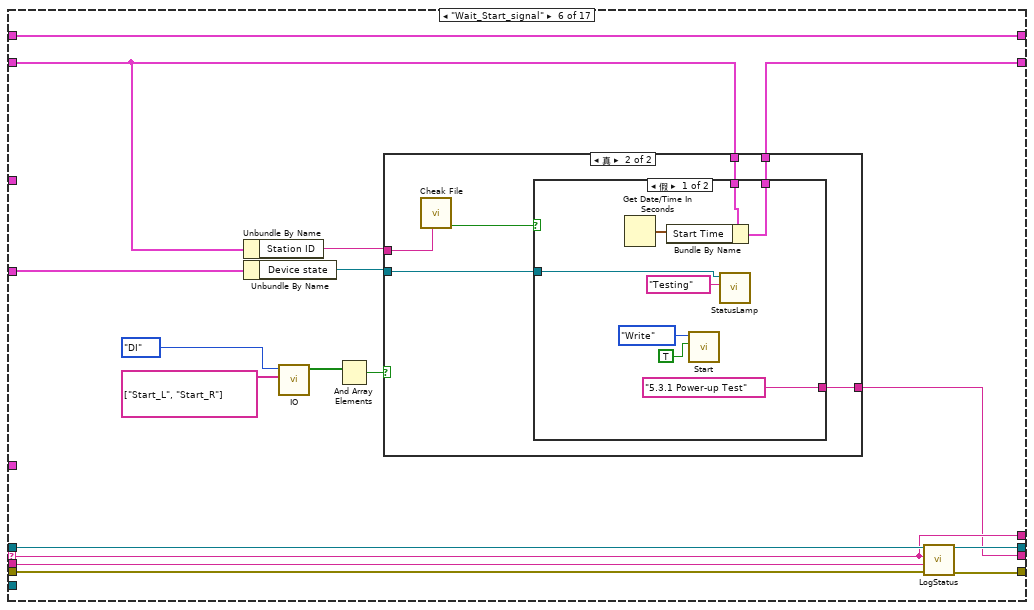
[diagram p14: hidden frame]
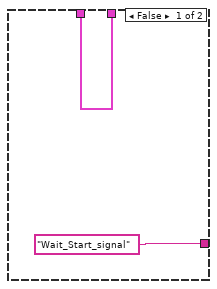
[diagram p15: hidden frame]
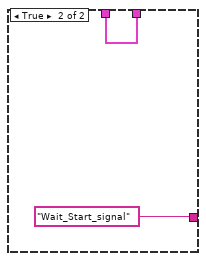
[diagram p16: hidden frame]
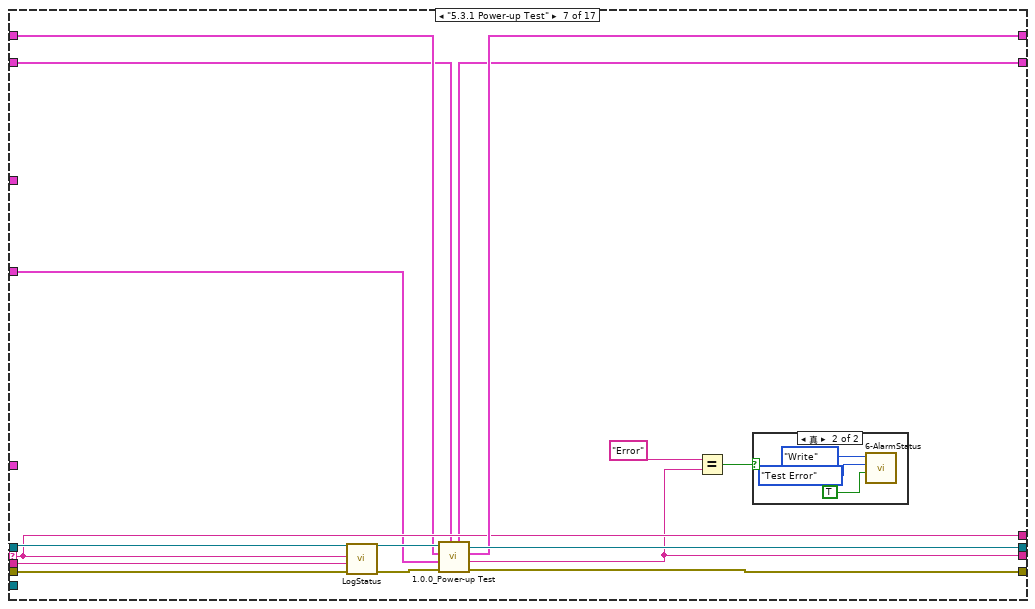
[diagram p17: hidden frame]
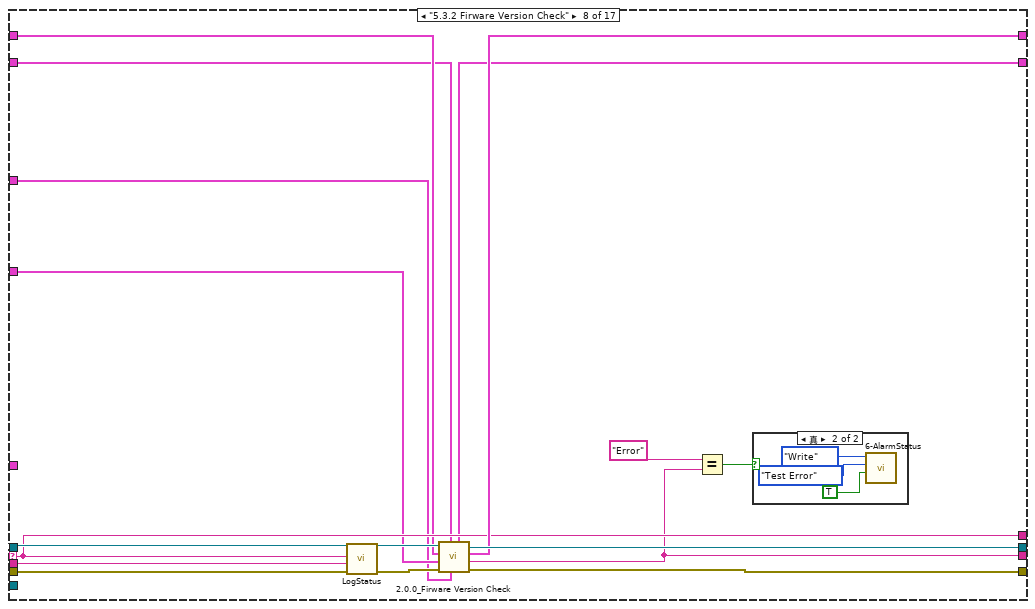
[diagram p19: hidden frame]
diagram:
  w3 = T3 {"Initialisation"={"LMT - Connect UUT (con COM)"="", "LMT - Software Version (rrel)"="", "LMT - Write SKU file (wskuc)"="", "LMT - SKU file name"="", "Connect UUT DDM"="", "Read DDM EOL Timestamp - Mode"="", "Read DDM EOL Timestamp - Timestamp"="", "Read DDM EOL Timestamp - Rig ID"="", "Read DDM EOL Timestamp - Passmark ID"="", "Read DDM EOL Timestamp - Passmark Rev"="", "Software Version before flashing"="", "Read Hardware Serial"="", "UUT DDM SN"="", "Compare DDM SN with MES SN"="", "Backup PCBA Calibration EEPROM Response - CAL"="", "Flash Firmware Version"="", "Check SW Version"="", "Read DDM SW Version after flashing"="", "Set SKU Config"="", "Ready Status"="", "Set Device Mode to EOL"="", "DDM Parameter - Voltage"="", "DDM Parameter - Current"="", "DDM Parameter - Power"="", "DDM Parameter - Speed"="", "DDM Parameter - Pressure"="", "Tester Parameter - Voltage"="", "Tester Parameter - Current"="", "Tester Parameter - Power"="", "Tester Parameter - Ambient Pressure"="", "Tester Parameter - Ambient Temperature"="", "Calculated Parameter - DDM Pressure Corrected"="", "Calculated Parameter - DDM Real Power"="", "Calculated Parameter - Delta V"=""}, "BEMF_Calibration"={"Calibration Result - eol_cold_bemf_temp"="", "DDM Ambient Temp"="", "Restriction Plate Diameter"="", "Calibration Result - eol_bemf_mp_cold_coef_a"="", "Calibration Result - eol_bemf_mp_cold_coef_b"="", "Calibration Result - eol_bemf_mp_cold_coef_c"="", "Calibration Result - eol_bemf_lsi_cold_ref_coeffs"="", "Get - Calibration Result - eol_bemf_lsi_speed"="", "Get - Calibration Result - eol_bemf_lsi_integral_0"="", "Calibration Result - eol_bemf_lsi_integral_1"="", "Get - Calibration Result - eol_bemf_lsi_integral_2"="", "Get - Calibration Result - eol_cold_bemf"="", "Get - Calibration Result - eol_cold_bemf_fisf"="", "Finalise Calibration"="", "Compare -Calibration Result - eol_cold_bemf"="", "Compare -Calibration Result - eol_cold_bemf_fisf"=""}, "ECO"={"Reset Power Tune"="", "Reset BEMF FISF Calibration"="", "Restriction Plate Diameter"="", "ECO - Stabilisation Time"="", "ECO - DDM Parameter - Voltage"="", "ECO - DDM Parameter - Current"="", "ECO - DDM Parameter - Power"="", "ECO - DDM Parameter - Measured Power"="", "ECO - DDM Parameter - Speed"="", "ECO - DDM Parameter - Pressure"="", "ECO - Tester Parameter - Voltage"="", "ECO - Tester Parameter - Current"="", "ECO - Tester Parameter - Power"="", "ECO - Tester Parameter - Ambient Pressure"="", "ECO - Tester Parameter - Ambient Temperature"="", "ECO - Tester Parameter - Ambient Humidity"="", "ECO - Calculated Parameter - DDM Pressure Corrected"="", "ECO - Calculated Parameter - DDM Real Power"="", "ECO - Calculated Parameter - Delta V"="", "ECO - Calculated Parameter - Flowrate"="", "ECO - Calculated Parameter - Airwatt"="", "ECO - Formula"="", "PT ECO - Power Tune Mode Status"=""}, "BOOST"={"Restriction Plate Diameter"="", "BOOST - Stabilisation Time"="", "BOOST - DDM Parameter - Voltage"="", "BOOST - DDM Parameter - Current"="", "BOOST - DDM Parameter - Power"="", "BOOST - DDM Parameter - Measured Power"="", "BOOST - DDM Parameter - Speed"="", "BOOST - DDM Parameter - Pressure"="", "BOOST - Tester Parameter - Voltage"="", "BOOST - Tester Parameter - Current"="", "BOOST - Tester Parameter - Power"="", "BOOST - Tester Parameter - Ambient Pressure"="", "BOOST - Tester Parameter - Ambient Temperature"="", "BOOST - Tester Parameter - Ambient Humidity"="", "BOOST - Calculated Parameter - DDM Pressure Corrected"="", "BOOST - Calculated Parameter - DDM Real Power"="", "BOOST - Calculated Parameter - Delta V"="", "BOOST - Calculated Parameter - Flowrate"="", "BOOST - Calculated Parameter - Airwatt"="", "BOOST - Get AM Presence"="", "Air Muscle Turn Off Status"="", "BOOST - Air Muscle Calculated Parameter - Airwatt B"="", "BOOST - Air Muscle Calculate Airwatt Delta"="", "PT BOOST - Power Tune Mode Status"="", "Finalise Calibration"="", "ECO - Get AW Calibration value"="", "BOOST - Get AW Calibration value"=""}, "MAX"={"Restriction Plate Diameter"="", "MAX - Stabilisation Time"="", "Get Average Delta Tmag (LSIdelta_FISFdelta_LSItmag_FISFtmag_IIRtmag)"="", "Get Average Delta Tmag FISF"="", "MAX - DDM Parameter - Voltage"="", "MAX - DDM Parameter - Current"="", "MAX - DDM Parameter - Power"="", "MAX - DDM Parameter - Measured Power"="", "MAX - DDM Parameter - Speed"="", "MAX - DDM Parameter - Pressure"="", "MAX - Tester Parameter - Voltage"="", "MAX - Tester Parameter - Current"="", "MAX - Tester Parameter - Power"="", "MAX - Tester Parameter - Ambient Pressure"="", "MAX - Tester Parameter - Ambient Temperature"="", "MAX - Tester Parameter - Ambient Humidity"="", "MAX - Calculated Parameter - DDM Pressure Corrected"="", "MAX - Calculated Parameter - DDM Real Power"="", "MAX - Calculated Parameter - Delta V"="", "MAX - Calculated Parameter - Flowrate"="", "MAX - Calculated Parameter - Airwatt"="", "MAX_FISF_Check_Average_Delta_Tmag"="", "MAX - FISF - BEMF Finetune Result"="No BEMF Finetune Required", "MAX tune - Delta P1"="No AW tune required", "MAX tune - Calculated Parameter - Airwatt"="", "Calculate Delta Airwatts - MAX finetune - Delta P2"="No AW finetune required", "MAX finetune - DDM Parameter - Voltage"="", "MAX finetune - DDM Parameter - Current"="", "MAX finetune - DDM Parameter - Power"="", "MAX finetune - DDM Parameter - Measured Power"="", "MAX finetune - DDM Parameter - Speed"="", "MAX finetune - DDM Parameter - Pressure"="", "MAX finetune - Tester Parameter - Voltage"="", "MAX finetune - Tester Parameter - Current"="", "MAX finetune - Tester Parameter - Power"="", "MAX finetune - Tester Parameter - Ambient Pressure"="", "MAX finetune - Tester Parameter - Ambient Temperature"="", "MAX finetune - Tester Parameter - Ambient Humidity"="", "MAX finetune - Calculated Parameter - DDM Pressure Corrected"="", "MAX finetune - Calculated Parameter - DDM Real Power"="", "MAX finetune - Calculated Parameter - Delta V"="", "MAX finetune - Calculated Parameter - Flowrate"="", "MAX finetune - Calculated Parameter - Airwatt"="", "Check Derate Result"="", "Delta Tmag FISF"="", "Get Hot BEMF Result"="", "Calculate delta Pressure"="", "Finalise Calibration"="", "Calculate & Check Delta BEMF"="", "Delta P Airwatts Value"=""}, "LL"={"DDM Ambient Temp"="", "Restriction Plate Diameter"="", "LL - DDM Parameter - Voltage"="", "LL - DDM Parameter - Current"="", "LL - DDM Parameter - Power"="", "LL - DDM Parameter - Measured Power"="", "LL - DDM Parameter - Speed"="", "LL - DDM Parameter - Pressure"="", "LL - Tester Parameter - Voltage"="", "LL - Tester Parameter - Current"="", "LL - Tester Parameter - Power"="", "LL - DDM Real Power"="", "LL - Calibrate Task Detect LL"=""}, "HL"={"HL - DDM Parameter - Voltage"="", "HL - DDM Parameter - Current"="", "HL - DDM Parameter - Power"="", "HL - DDM Parameter - Measured Power"="", "HL - DDM Parameter - Speed"="", "HL - DDM Parameter - Pressure"="", "HL - Tester Parameter - Voltage"="", "HL - Tester Parameter - Current"="", "HL - Tester Parameter - Power"="", "HL - DDM Real Power"="", "HL - Calibrate Task Detect HL"=""}, "LH"={"Restriction Plate Diameter"="", "LH - DDM Parameter - Voltage"="", "LH - DDM Parameter - Current"="", "LH - DDM Parameter - Power"="", "LH - DDM Parameter - Measured Power"="", "LH - DDM Parameter - Speed"="", "LH - DDM Parameter - Pressure"="", "LH - Tester Parameter - Voltage"="", "LH - Tester Parameter - Current"="", "LH - Tester Parameter - Power"="", "LH - DDM Real Power"="", "LH - Calibrate Task Detect LH"=""}, "HH"={"HH - DDM Parameter - Voltage"="", "HH - DDM Parameter - Current"="", "HH - DDM Parameter - Power"="", "HH - DDM Parameter - Measured Power"="", "HH - DDM Parameter - Speed"="", "HH - DDM Parameter - Pressure"="", "HH - Tester Parameter - Voltage"="", "HH - Tester Parameter - Current"="", "HH - Tester Parameter - Power"="", "HH - DDM Real Power"="", "HH - Calibrate Task Detect HH"=""}, "Inlet Blockage Calibration"={"Inlet Blockage Calibration - DDM Parameter - Voltage"="", "Inlet Blockage Calibration - DDM Parameter - Current"="", "Inlet Blockage Calibration - DDM Parameter - Power"="", "Inlet Blockage Calibration - DDM Parameter - Measured Power"="", "Inlet Blockage Calibration - DDM Parameter - Speed"="", "Inlet Blockage Calibration - DDM Parameter - Pressure"="", "Inlet Blockage Calibration - Tester Parameter - Voltage"="", "Inlet Blockage Calibration - Tester Parameter - Current"="", "Inlet Blockage Calibration - Tester Parameter - Power"="", "Inlet Blockage Calibration - DDM Real Power"="", "Calibration Inlet Blockage_E"="", "Finalise Calibration"="", "Get Task Detect LL"="", "Get Task Detect HL"="", "Get Task Detect LH"="", "Get Task Detect HH"="", "Calibration Inlet Blockage"="", "Calibration eol cold bemf temp"=""}, "GOOD"={"GOOD UNIT - Clear EEPROM Error Log"="", "GOOD UNIT - Write Product Timestamp - Mode"="", "GOOD UNIT - Write Product Timestamp - Timestamp"="", "GOOD UNIT - Write Product Timestamp - Rig ID"="", "GOOD UNIT - Write Product Timestamp - Passmark ID"="", "GOOD UNIT - Write Product Timestamp - Passmark Rev"="", "GOOD UNIT - Set Device Mode to PROD"="", "GOOD UNIT - Backup PCBA Calibration EEPROM Response"="", "GOOD UNIT - Check Security Bit"="", "GOOD UNIT - Set Calibration Lock"="", "GOOD UNIT - Get_Calibration_Lock"="", "GOOD UNIT - Disconnect UUT"=""}, "NG"={"NG UNIT - Read NVM Error"="", "NG UNIT - Set Device Mode to FCT"="", "NG UNIT - Backup PCBA Calibration EEPROM Response - CAL"="", "NG UNIT - Backup PCBA Calibration EEPROM Response - ERROR"="", "NG UNIT - Backup PCBA Calibration EEPROM Response - USAGE"="", "NG UNIT - Disconnect UUT"=""}, "SN"="", "Table"=[], "Count"={"Total"=0, "OK"=0, "NG"=0, "Yield"=0.0}, "Start Time"=timestamp(0 s since 1904-01-01), "daemon reference"=refnum, "CT"=0.0, "Config"=[], "OK/NG"=FALSE, "Station ID"="", "MES DDM SN"="", "MES PCBA SN"="", "Retest"="", "Lux"="", "Initialisation_Status"={"LMT - Connect UUT (con COM)"="", "LMT - Software Version (rrel)"="", "LMT - Write SKU file (wskuc)"="", "LMT - SKU file name"="", "Connect UUT DDM"="", "Read DDM EOL Timestamp - Mode"="", "Read DDM EOL Timestamp - Timestamp"="", "Read DDM EOL Timestamp - Rig ID"="", "Read DDM EOL Timestamp - Passmark ID"="", "Read DDM EOL Timestamp - Passmark Rev"="", "Software Version before flashing"="", "Read Hardware Serial"="", "UUT DDM SN"="", "Compare DDM SN with MES SN"="", "Backup PCBA Calibration EEPROM Response - CAL"="", "Flash Firmware Version"="", "Check SW Version"="", "Read DDM SW Version after flashing"="", "Set SKU Config"="", "Ready Status"="", "Set Device Mode to EOL"="", "DDM Parameter - Voltage"="", "DDM Parameter - Current"="", "DDM Parameter - Power"="", "DDM Parameter - Speed"="", "DDM Parameter - Pressure"="", "Tester Parameter - Voltage"="", "Tester Parameter - Current"="", "Tester Parameter - Power"="", "Tester Parameter - Ambient Pressure"="", "Tester Parameter - Ambient Temperature"="", "Calculated Parameter - DDM Pressure Corrected"="", "Calculated Parameter - DDM Real Power"="", "Calculated Parameter - Delta V"=""}, "BEMF_Calibration_Status"={"Calibration Result - eol_cold_bemf_temp"="", "DDM Ambient Temp"="", "Restriction Plate Diameter"="", "Calibration Result - eol_bemf_mp_cold_coef_a"="", "Calibration Result - eol_bemf_mp_cold_coef_b"="", "Calibration Result - eol_bemf_mp_cold_coef_c"="", "Calibration Result - eol_bemf_lsi_cold_ref_coeffs"="", "Get - Calibration Result - eol_bemf_lsi_speed"="", "Get - Calibration Result - eol_bemf_lsi_integral_0"="", "Calibration Result - eol_bemf_lsi_integral_1"="", "Get - Calibration Result - eol_bemf_lsi_integral_2"="", "Get - Calibration Result - eol_cold_bemf"="", "Get - Calibration Result - eol_cold_bemf_fisf"="", "Finalise Calibration"="", "Compare -Calibration Result - eol_cold_bemf"="", "Compare -Calibration Result - eol_cold_bemf_fisf"=""}, "ECO_Status"={"Reset Power Tune"="", "Reset BEMF FISF Calibration"="", "Restriction Plate Diameter"="", "ECO - Stabilisation Time"="", "ECO - DDM Parameter - Voltage"="", "ECO - DDM Parameter - Current"="", "ECO - DDM Parameter - Power"="", "ECO - DDM Parameter - Measured Power"="", "ECO - DDM Parameter - Speed"="", "ECO - DDM Parameter - Pressure"="", "ECO - Tester Parameter - Voltage"="", "ECO - Tester Parameter - Current"="", "ECO - Tester Parameter - Power"="", "ECO - Tester Parameter - Ambient Pressure"="", "ECO - Tester Parameter - Ambient Temperature"="", "ECO - Tester Parameter - Ambient Humidity"="", "ECO - Calculated Parameter - DDM Pressure Corrected"="", "ECO - Calculated Parameter - DDM Real Power"="", "ECO - Calculated Parameter - Delta V"="", "ECO - Calculated Parameter - Flowrate"="", "ECO - Calculated Parameter - Airwatt"="", "ECO - Formula"="", "PT ECO - Power Tune Mode Status"=""}, "BOOST_Status"={"Restriction Plate Diameter"="", "BOOST - Stabilisation Time"="", "BOOST - DDM Parameter - Voltage"="", "BOOST - DDM Parameter - Current"="", "BOOST - DDM Parameter - Power"="", "BOOST - DDM Parameter - Measured Power"="", "BOOST - DDM Parameter - Speed"="", "BOOST - DDM Parameter - Pressure"="", "BOOST - Tester Parameter - Voltage"="", "BOOST - Tester Parameter - Current"="", "BOOST - Tester Parameter - Power"="", "BOOST - Tester Parameter - Ambient Pressure"="", "BOOST - Tester Parameter - Ambient Temperature"="", "BOOST - Tester Parameter - Ambient Humidity"="", "BOOST - Calculated Parameter - DDM Pressure Corrected"="", "BOOST - Calculated Parameter - DDM Real Power"="", "BOOST - Calculated Parameter - Delta V"="", "BOOST - Calculated Parameter - Flowrate"="", "BOOST - Calculated Parameter - Airwatt"="", "BOOST - Get AM Presence"="", "Air Muscle Turn Off Status"="", "BOOST - Air Muscle Calculated Parameter - Airwatt B"="", "BOOST - Air Muscle Calculate Airwatt Delta"="", "PT BOOST - Power Tune Mode Status"="", "Finalise Calibration"="", "ECO - Get AW Calibration value"="", "BOOST - Get AW Calibration value"=""}, "MAX_Status"={"Restriction Plate Diameter"="", "MAX - Stabilisation Time"="", "Get Average Delta Tmag (LSIdelta_FISFdelta_LSItmag_FISFtmag_IIRtmag)"="", "Get Average Delta Tmag FISF"="", "MAX - DDM Parameter - Voltage"="", "MAX - DDM Parameter - Current"="", "MAX - DDM Parameter - Power"="", "MAX - DDM Parameter - Measured Power"="", "MAX - DDM Parameter - Speed"="", "MAX - DDM Parameter - Pressure"="", "MAX - Tester Parameter - Voltage"="", "MAX - Tester Parameter - Current"="", "MAX - Tester Parameter - Power"="", "MAX - Tester Parameter - Ambient Pressure"="", "MAX - Tester Parameter - Ambient Temperature"="", "MAX - Tester Parameter - Ambient Humidity"="", "MAX - Calculated Parameter - DDM Pressure Corrected"="", "MAX - Calculated Parameter - DDM Real Power"="", "MAX - Calculated Parameter - Delta V"="", "MAX - Calculated Parameter - Flowrate"="", "MAX - Calculated Parameter - Airwatt"="", "MAX_FISF_Check_Average_Delta_Tmag"="", "MAX - FISF - BEMF Finetune Result"="", "MAX tune - Delta P1"="", "MAX tune - Calculated Parameter - Airwatt"="", "Calculate Delta Airwatts - MAX finetune - Delta P2"="", "MAX finetune - DDM Parameter - Voltage"="", "MAX finetune - DDM Parameter - Current"="", "MAX finetune - DDM Parameter - Power"="", "MAX finetune - DDM Parameter - Measured Power"="", "MAX finetune - DDM Parameter - Speed"="", "MAX finetune - DDM Parameter - Pressure"="", "MAX finetune - Tester Parameter - Voltage"="", "MAX finetune - Tester Parameter - Current"="", "MAX finetune - Tester Parameter - Power"="", "MAX finetune - Tester Parameter - Ambient Pressure"="", "MAX finetune - Tester Parameter - Ambient Temperature"="", "MAX finetune - Tester Parameter - Ambient Humidity"="", "MAX finetune - Calculated Parameter - DDM Pressure Corrected"="", "MAX finetune - Calculated Parameter - DDM Real Power"="", "MAX finetune - Calculated Parameter - Delta V"="", "MAX finetune - Calculated Parameter - Flowrate"="", "MAX finetune - Calculated Parameter - Airwatt"="", "Check Derate Result"="", "Delta Tmag FISF"="", "Get Hot BEMF Result"="", "Calculate delta Pressure"="", "Finalise Calibration"="", "Calculate & Check Delta BEMF"="", "Delta P Airwatts Value"=""}, "LL_Status"={"DDM Ambient Temp"="", "Restriction Plate Diameter"="", "LL - DDM Parameter - Voltage"="", "LL - DDM Parameter - Current"="", "LL - DDM Parameter - Power"="", "LL - DDM Parameter - Measured Power"="", "LL - DDM Parameter - Speed"="", "LL - DDM Parameter - Pressure"="", "LL - Tester Parameter - Voltage"="", "LL - Tester Parameter - Current"="", "LL - Tester Parameter - Power"="", "LL - DDM Real Power"="", "LL - Calibrate Task Detect LL"=""}, "HL_Status"={"HL - DDM Parameter - Voltage"="", "HL - DDM Parameter - Current"="", "HL - DDM Parameter - Power"="", "HL - DDM Parameter - Measured Power"="", "HL - DDM Parameter - Speed"="", "HL - DDM Parameter - Pressure"="", "HL - Tester Parameter - Voltage"="", "HL - Tester Parameter - Current"="", "HL - Tester Parameter - Power"="", "HL - DDM Real Power"="", "HL - Calibrate Task Detect HL"=""}, "LH_Status"={"Restriction Plate Diameter"="", "LH - DDM Parameter - Voltage"="", "LH - DDM Parameter - Current"="", "LH - DDM Parameter - Power"="", "LH - DDM Parameter - Measured Power"="", "LH - DDM Parameter - Speed"="", "LH - DDM Parameter - Pressure"="", "LH - Tester Parameter - Voltage"="", "LH - Tester Parameter - Current"="", "LH - Tester Parameter - Power"="", "LH - DDM Real Power"="", "LH - Calibrate Task Detect LH"=""}, "HH_Status"={"HH - DDM Parameter - Voltage"="", "HH - DDM Parameter - Current"="", "HH - DDM Parameter - Power"="", "HH - DDM Parameter - Measured Power"="", "HH - DDM Parameter - Speed"="", "HH - DDM Parameter - Pressure"="", "HH - Tester Parameter - Voltage"="", "HH - Tester Parameter - Current"="", "HH - Tester Parameter - Power"="", "HH - DDM Real Power"="", "HH - Calibrate Task Detect HH"=""}, "Inlet Blockage Calibration_Status"={"Inlet Blockage Calibration - DDM Parameter - Voltage"="", "Inlet Blockage Calibration - DDM Parameter - Current"="", "Inlet Blockage Calibration - DDM Parameter - Power"="", "Inlet Blockage Calibration - DDM Parameter - Measured Power"="", "Inlet Blockage Calibration - DDM Parameter - Speed"="", "Inlet Blockage Calibration - DDM Parameter - Pressure"="", "Inlet Blockage Calibration - Tester Parameter - Voltage"="", "Inlet Blockage Calibration - Tester Parameter - Current"="", "Inlet Blockage Calibration - Tester Parameter - Power"="", "Inlet Blockage Calibration - DDM Real Power"="", "Calibration Inlet Blockage_E"="", "Finalise Calibration"="", "Get Task Detect LL"="", "Get Task Detect HL"="", "Get Task Detect LH"="", "Get Task Detect HH"="", "Calibration Inlet Blockage"="", "Calibration eol cold bemf temp"=""}, "GOOD_Status"={"GOOD UNIT - Clear EEPROM Error Log"="", "GOOD UNIT - Write Product Timestamp - Mode"="", "GOOD UNIT - Write Product Timestamp - Timestamp"="", "GOOD UNIT - Write Product Timestamp - Rig ID"="", "GOOD UNIT - Write Product Timestamp - Passmark ID"="", "GOOD UNIT - Write Product Timestamp - Passmark Rev"="", "GOOD UNIT - Set Device Mode to PROD"="", "GOOD UNIT - Backup PCBA Calibration EEPROM Response"="", "GOOD UNIT - Check Security Bit"="", "GOOD UNIT - Set Calibration Lock"="", "GOOD UNIT - Get_Calibration_Lock"="", "GOOD UNIT - Disconnect UUT"=""}, "NG_Status"={"NG UNIT - Read NVM Error"="", "NG UNIT - Set Device Mode to FCT"="", "NG UNIT - Backup PCBA Calibration EEPROM Response - CAL"="", "NG UNIT - Backup PCBA Calibration EEPROM Response - ERROR"="", "NG UNIT - Backup PCBA Calibration EEPROM Response - USAGE"="", "NG UNIT - Disconnect UUT"=""}, "SKU"="", "Plate_Diameter"="", "Alarm"=""}  # Data in
  w8 = T4 {"Initialisation"={"DDM_Parameter"=[], "DDM_Parameter_status"=[], "Get_Tester_Parameter"=[], "Get_Tester_Parameter_status"=[], "Cal_Tester_Parameter"=[], "Cal_Tester_Parameter_status"=[], "sw_version_before_status"=FALSE, "sw_version_after_status"=FALSE, "Set_SKU_Config_With_LMT_status"=FALSE, "FCT_timestamp_status"=FALSE, "LMT_Connect_to_UUT_status"=FALSE}, "BEMF_Calibration"={"Read_ambient_temperature"=0.0, "Calibration_Vaule"=[], "Calibration_Vaule _B"=[], "Calibration_Vaule_status"=[], "Calibration_Vaule_B_status"=[]}, "ECO"={"DDM_Parameter"=[], "DDM_Parameter_status"=[], "Get_Tester_Parameter"=[], "Get_Tester_Parameter_status"=[], "Cal_Tester_Parameter"=[], "Cal_Tester_Parameter_status"=[], "DDM_Parameter_after_power_tune"=[], "Get_Tester_Parameter_after_power_tune"=[], "Cal_Tester_Parameter_after_power_tune"=[], "Cal_Tester_Parameter_after_power_tune_status"=[], "Delta_P"=0.0}, "BOOST"={"DDM_Parameter"=[], "DDM_Parameter_status"=[], "Get_Tester_Parameter"=[], "Get_Tester_Parameter_status"=[], "Cal_Tester_Parameter"=[], "Cal_Tester_Parameter_status"=[], "DDM_Parameter_after_power_tune"=[], "Get_Tester_Parameter_after_power_tune"=[], "Cal_Tester_Parameter_after_power_tune"=[], "Cal_Tester_Parameter_after_power_tune_status"=[], "airwatts_am_off"=0.0, "AW_Delta_(AM_on_and_off)"=0.0, "AW_Delta_(AM_on_and_off)_Status"=FALSE, "Delta_P"=0.0}, "MAX"={"Average_Tmag_Data"={"LSI Delta in degC"=0.0, "FISF Delta in degc"=0.0, "LSI Tmag in degC"=0.0, "Fisf Tmag in degC"=0.0, "IIR Tmag in degC"=0.0}, "DDM_Parameter"=[], "DDM_Parameter_status"=[], "Get_Tester_Parameter"=[], "Get_Tester_Parameter_status"=[], "Cal_Tester_Parameter"=[], "BEMF_Finetune"={"eol_bemf_mp_cold_coef_c"=0.0, "eol_cold_bemf_fisf_offset"=0.0}, "AW_Tune"={"delta_P1"=0.0, "delta_P_Setting"=0.0}, "DDM_Parameter_after_Airwatts_Tune"=[], "Get_Tester_Parameter_after_Airwatts_Tune"=[], "Cal_Tester_Parameter_after_Airwatts_Tune"=[], "DDM_Parameter_after_Airwatts_Finetune"=[], "Get_Tester_Parameter_after_Airwatts_Finetune"=[], "Cal_Tester_Parameter_after_Airwatts_Finetune"=[], "AW_Finetune"={"delta_P2"=0.0, "delta_P_Setting"=0.0}, "Delta_Tmag_after_tune"={"LSI Delta in degC"=0.0, "FISF Delta in degc"=0.0, "LSI Tmag in degC"=0.0, "Fisf Tmag in degC"=0.0, "IIR Tmag in degC"=0.0}, "Hot Bemf in mV"=0.0, "DDM_Pressure"=0.0, "Delta_Pressure"=0.0, " Cold Bemf in mV"=0.0, " delta Bemf"=0.0, " delta p"=0.0, "Delta_Pressure_status"=FALSE, " delta Bemf_status"=FALSE, "LSI Delta in degC_status"=FALSE, "FISF Delta in degc_status"=FALSE, "Max_check_derate_status_status"=FALSE, "Average_All_data"=[], "Average_Tmag_Data_status"=[], "Average_Tmag_Data_after_tune_status"=[], "Cal_Tester_Parameter_status"=[], "Cal_Tester_Parameter_status_after_Airwatts_Tune"=[], "Cal_Tester_Parameter_status_after_Airwatts_FineTune"=[]}, "Task_Detect_Calib"={"LL"={"DDM_Parameter"=[], "DDM_Parameter_status"=[], "Get_Tester_Parameter"=[], "Get_Tester_Parameter_status"=[], "Set_task_detect_A"=0.0, "Set_task_detect_A_Status"=FALSE}, "HL"={"DDM_Parameter"=[], "DDM_Parameter_status"=[], "Get_Tester_Parameter"=[], "Get_Tester_Parameter_status"=[], "Set_task_detect_B"=0.0, "Set_task_detect_B_Status"=FALSE}, "LH"={"DDM_Parameter"=[], "DDM_Parameter_status"=[], "Get_Tester_Parameter"=[], "Get_Tester_Parameter_status"=[], "Set_task_detect_C"=0.0, "Set_task_detect_C_Status"=FALSE}, "HH"={"DDM_Parameter"=[], "DDM_Parameter_status"=[], "Get_Tester_Parameter"=[], "Get_Tester_Parameter_status"=[], "Set_task_detect_D"=0.0, "Read_and_check_calibration_Status"=[], "Set_task_detect_D_Status"=FALSE}, "Get_eol_inlet_blockage_E"=0.0, "Calib_vaule"={"Get_task_detect_LL"=0.0, "Get_task_detect_HL"=0.0, "Get_task_detect_LH"=0.0, "Get_task_detect_HH"=0.0, "eol_inlet_blockage"=0.0, "eol_code_bemf_temp"=0.0}, "calibrated temp"=0.0, "Inlet_Blockage_Calibration"={"DDM_Parameter"=[], "DDM_Parameter_status"=[], "Get_Tester_Parameter"=[], "Get_Tester_Parameter_status"=[]}, "Get_eol_inlet_blockage_E_Status"=FALSE}, "good"={"Write_Product_TS"={"TIMESTAMP"=0, "RIG_ID"=0, "PASSMARK_ID"=0, "PASSMARK_REV"=0}, "Read_Product_TS"={"TIMESTAMP"=0, "RIG_ID"=0, "PASSMARK_ID"=0, "PASSMARK_REV"=0}, "Good_Check_Secuity_Bit_Stauts"=FALSE}}  # Data
  n1 = call "AMC Create Message Queue.vi"("error in (no error)"=errorcluster {"status"=FALSE, "code"=0, "source"=""}, "Initial Message Names"=string[] ["Initialize_UI"] ("Initial Message Values"), "Message Queue Name"="AutoRun" ("Message queue name (unnamed)")) -> ("error out"=w18:errorcluster, "Message Queue out"=w19:T5)  [unwired: 2 in, 5 out]
  n2 = call "AMC Create Message Queue.vi"("Initial Message Names"=string[] ["Wait"], "Message Queue Name"="DSave") -> ("Message Queue out"=w14:T5)  [unwired: 3 in, 6 out]
  n3 = call "SW_Config.vi"("Step"=enum16{"Initial", "Write", "Read"}."Read") -> ("SW Config out"=w10:T6)  [unwired: 9 in, 1 out]
  n4 = while {
    tunnel: "AllControls In" -> [w33]
    shift-right: [w40] -> w6
    shift-left: w19 -> [w44]
    shift-right: [w41] -> w5
    shift-left: w18 -> [w43]
    tunnel: w14 -> [w38]
    shift-right: [w26] -> _
    shift-left: w8 -> [w27]
    tunnel: w10 -> [w25]
    shift-right: [w24] -> w9
    shift-left: w3 -> [w23]
    tunnel: T2 {"Brush_ADC.bat"="Brush_ADC.bat", "Get Release Version.bat"="Get Release Version.bat", "Getting Software  Version.bat"="Getting Software  Version.bat", "Pump_ADC.bat"="Pump_ADC.bat", "Starting  Pump Motor.bat"="Starting  Pump Motor.bat", "Starting  Test Mode.bat"="Starting  Test Mode.bat", "Starting Brush Motor 1.bat"="Starting Brush Motor 1.bat", "Starting Brush Motor 2.bat"="Starting Brush Motor 2.bat", "Starting Brush Motor 3.bat"="Starting Brush Motor 3.bat", "Starting LED Test.bat"="Starting LED Test.bat", "Stopping  Brush Motor.bat"="Stopping  Brush Motor.bat", "Stopping  Pump Motor.bat"="Stopping  Pump Motor.bat", "Stopping  Test Mode.bat"="Stopping  Test Mode.bat", "Starting Self Test.bat"="Starting Self Test.bat", "Software Reset.bat"="Software Reset.bat", "Get HW version.bat"="Get HW version.bat", "Read PMIC status.bat"="Read PMIC status.bat", "SC IMU Data Streaming.bat"="SC IMU Data Streaming.bat"} (".batCMD") -> [w22]
    stop <- w21 stop-if-true
    n5 = call "AMC Read Next Message.vi"("error in (no error)"=w43, "timeout (1ms)"=100 ("Timeout"), "Message Queue in"=w44) -> ("error out"=w34:errorcluster, "Message Value"=w28:string, "Message Name"=w37:string, "Message Queue out"=w36:T5)  [unwired: 1 in, 4 out]
    n6 = Wait (ms)(milliseconds to wait=u32 1) -> ()  [unwired: 1 out]
    n7 = case shown="\"Stop_E-Stop\"" w37 {
      selector: w37 -> [_ w50 w92 w217 w1165 w1184 w1216 w1235 w1254 w1273 w1292 w1323 w1378 w1402 w1441 w1451 w1521]
      tunnel: w38 -> [_ _ _ _ _ _ _ _ _ _ _ _ w1382 _ _ _ _]
      tunnel: w36 -> [w48 w75 w106 w223 w1173 w1189 w1220 w1239 w1258 w1277 w1296 w1326 w1383 w1407 w1444 w1475 w1523]
      tunnel: [w48 w75 w106 w223 w1173 w1189 w1219 w1238 w1257 w1276 w1295 w1326 w1383 w1407 w1444 w1475 w1523] -> w35
      tunnel: w34 -> [w47 w55 w105 w222 w1172 w1188 w1222 w1241 w1260 w1279 w1298 w1325 w1380 w1406 w1443 w1474 w1518]
      tunnel: [w47 w71 w104 w221 w1171 w1187 w1218 w1237 w1256 w1275 w1294 w1324 w1379 w1405 w1442 w1473 w1520] -> w31
      tunnel: w33 -> [_ w73 w100 w219 _ w1180 w1211 w1230 w1249 w1268 w1287 _ w1369 w1384 w1432 w1463 _]
      tunnel: [_ _ _ _ _ _ _ _ _ _ _ _ _ _ _ _ TRUE] -> w21
      tunnel: [_ "Wait_Scan_ProductID" w98 "Wait_Start_signal" w1167 w1178 w1208 w1227 w1246 w1265 w1284 "UI_Display_and_Save_Test_Data" w1335 "Wait_Scan_ProductID" w1433 w1462 _] -> w30
      tunnel: [_ w50 w92 w217 w1165 w1184 w1216 w1235 w1254 w1273 w1292 w1323 w1378 w1402 w1441 w1451 _] -> w29
      tunnel: w28 -> [_ w65 w96 w218 w1164 w1183 w1221 w1240 w1259 w1278 w1297 w1322 w1377 w1403 w1440 w1450 _]
      tunnel: w27 -> [w46 w52 w93 w209 w1166 w1175 w1215 w1234 w1253 w1272 w1291 w1318 w1343 w1401 w1426 w1460 w1519]
      tunnel: [w46 w52 w94 w209 w1166 w1175 w1217 w1236 w1255 w1274 w1293 w1318 w1343 w1401 w1426 w1460 w1519] -> w26
      tunnel: w25 -> [_ _ w85 w212 _ _ _ _ _ _ _ _ _ w1386 _ _ _]
      tunnel: [w45 w51 w83 w207 w1160 w1174 w1210 w1229 w1248 w1267 w1286 w1319 w1342 w1388 w1416 w1455 w1517] -> w24
      tunnel: w23 -> [w45 w51 w82 w208 w1160 w1176 w1209 w1228 w1247 w1266 w1285 w1317 w1341 w1388 w1416 w1456 w1517]
      tunnel: w22 -> [_ _ _ _ _ _ _ w1226 w1245 w1264 w1283 _ _ _ _ _ _]
      frame "Empty", Default {
      }
      frame "Initialize_UI" {
        n8 = call "Start.vi"("Start In"=FALSE, "Step"=enum16{"Initial", "Write", "Read"}."Write") -> ()  [unwired: 8 in, 2 out]
        n9 = Unbundle By Name(w73) -> ("Table"=w60:refnum<vi>, "ProductID"=w68:refnum<vi>, "MES"=w74:refnum<vi>, "Device state"=w70:refnum<vi>, "TestInfo"=w59:refnum<vi>, "Current CT"=w57:refnum<vi>)
        n10 = property class="Tbl (strict)"(reference=w60, "Value"=string[][] [] ("值"), "Active Cell"=T8 {"Row"=-2, "Column"=-2} ("活动单元格:活动单元格"), "Cell BG Color"=u32 3421236, "Row Headers[]"=string[] [] ("Row Header Strings[]")) -> ()  [unwired: 1 in, 2 out]
        n11 = property class="Str"(reference=w68, "Value"="" ("值"), "DisabledEnum"=T9."Enabled" ("Disabled")) -> ()  [unwired: 1 in, 2 out]
        n12 = property class="Str"(reference=w74, "Value"="") -> ()  [unwired: 1 in, 2 out]
        n13 = property class="Clust (strict)"(reference=w59, "Value"=T7 {"Total"=0, "OK"=0, "NG"=0, "Yield"=0.0}) -> ()  [unwired: 1 in, 2 out]
        n14 = property class="DigNum (strict)"(reference=w57, "Value"=0.0) -> ()  [unwired: 1 in, 2 out]
        n15 = call "StatusLamp.vi"("State"="StandBy", "Boolean输入"=w70) -> ()  [unwired: 9 in, 1 out]
        n16 = call "LogStatus.vi"("error in (no error)"=w55, "last message"=w65, "message"=w50) -> ("error  out"=w71:errorcluster)  [unwired: 8 in]
      }
      frame "Wait_Scan_ProductID" {
        n17 = Unbundle By Name(w85) -> ("FFTesterPath"=w84:path)
        n18 = Unbundle By Name(w100) -> ("Table"=w76:refnum<vi>, "MES"=w89:refnum<vi>, "ProductID"=w103:refnum<vi>, "MES bool"=w91:refnum<vi>, "Table"=w88:refnum<vi>, "Device state"=w87:refnum<vi>, "Current CT"=w86:refnum<vi>, "MES bool"=w78:refnum<vi>)
        n19 = call "HD_Config.vi"("Step"=enum16{"Initial", "Write", "Read"}."Read") -> ("HD Config out"=w80:T12)  [unwired: 9 in, 1 out]
        n20 = property class="Bool (strict)"(reference=w91) -> ("Value"=w90:bool)  [unwired: 1 in, 2 out]
        n21 = Unbundle By Name(w80) -> ("GRR"=w79:bool)
        n22 = property class="Bool (严格)"(reference=w78) -> ("Value"=w77:bool)  [unwired: 1 in, 2 out]
        n23 = property class="Str"(reference=w103, "Key Focus"=TRUE, "DisabledEnum"=T9."Enabled" ("Disabled")) -> (reference out=w97:refnum<vi>, "Value"=w95:string)  [unwired: 1 in, 1 out]
        n24 = Empty String/Path?(string/path=w95) -> (empty?=w99:bool)
        n25 = case shown="假" w99 {
          tunnel: ["MES_Verification" "Wait_Scan_ProductID"] -> w98
          tunnel: w97 -> [w139 _]
          tunnel: w93 -> [_ w157]
          tunnel: w95 -> [w122 _]
          tunnel: [T4 {"Initialisation"={"DDM_Parameter"=[nan, nan, nan, nan, nan], "DDM_Parameter_status"=[FALSE, FALSE, FALSE, FALSE, FALSE], "Get_Tester_Parameter"=[nan, nan, nan, nan, nan, nan], "Get_Tester_Parameter_status"=[FALSE, FALSE, FALSE, FALSE, FALSE, FALSE], "Cal_Tester_Parameter"=[nan, nan, nan], "Cal_Tester_Parameter_status"=[FALSE, FALSE, FALSE], "sw_version_before_status"=FALSE, "sw_version_after_status"=FALSE, "Set_SKU_Config_With_LMT_status"=FALSE, "FCT_timestamp_status"=FALSE, "LMT_Connect_to_UUT_status"=FALSE}, "BEMF_Calibration"={"Read_ambient_temperature"=nan, "Calibration_Vaule"=[nan, nan, nan, nan, nan, nan, nan, nan, nan, nan], "Calibration_Vaule _B"=[nan, nan], "Calibration_Vaule_status"=[FALSE, FALSE, FALSE, FALSE, FALSE, FALSE, FALSE, FALSE, FALSE, FALSE], "Calibration_Vaule_B_status"=[FALSE, FALSE]}, "ECO"={"DDM_Parameter"=[nan, nan, nan, nan, nan, nan, nan, nan, nan], "DDM_Parameter_status"=[FALSE, FALSE, FALSE, FALSE, FALSE, FALSE, FALSE, FALSE, FALSE], "Get_Tester_Parameter"=[nan, nan, nan, nan, nan, nan, nan], "Get_Tester_Parameter_status"=[FALSE, FALSE, FALSE, FALSE, FALSE, FALSE, FALSE], "Cal_Tester_Parameter"=[nan, nan, nan, nan, nan, nan], "Cal_Tester_Parameter_status"=[FALSE, FALSE, FALSE, FALSE, FALSE], "DDM_Parameter_after_power_tune"=[nan, nan, nan, nan, nan, nan, nan, nan, nan], "Get_Tester_Parameter_after_power_tune"=[nan, nan, nan, nan, nan, nan, nan], "Cal_Tester_Parameter_after_power_tune"=[nan, nan, nan, nan, nan, nan], "Cal_Tester_Parameter_after_power_tune_status"=[FALSE, FALSE, FALSE, FALSE, FALSE], "Delta_P"=nan}, "BOOST"={"DDM_Parameter"=[nan, nan, nan, nan, nan, nan, nan, nan, nan], "DDM_Parameter_status"=[FALSE, FALSE, FALSE, FALSE, FALSE, FALSE, FALSE, FALSE, FALSE], "Get_Tester_Parameter"=[nan, nan, nan, nan, nan, nan, nan], "Get_Tester_Parameter_status"=[FALSE, FALSE, FALSE, FALSE, FALSE, FALSE, FALSE], "Cal_Tester_Parameter"=[nan, nan, nan, nan, nan, nan], "Cal_Tester_Parameter_status"=[FALSE, FALSE, FALSE, FALSE, FALSE], "DDM_Parameter_after_power_tune"=[nan, nan, nan, nan, nan, nan, nan, nan, nan], "Get_Tester_Parameter_after_power_tune"=[nan, nan, nan, nan, nan, nan, nan], "Cal_Tester_Parameter_after_power_tune"=[nan, nan, nan, nan, nan, nan], "Cal_Tester_Parameter_after_power_tune_status"=[FALSE, FALSE, FALSE, FALSE, FALSE], "airwatts_am_off"=nan, "AW_Delta_(AM_on_and_off)"=nan, "AW_Delta_(AM_on_and_off)_Status"=FALSE, "Delta_P"=nan}, "MAX"={"Average_Tmag_Data"={"LSI Delta in degC"=nan, "FISF Delta in degc"=nan, "LSI Tmag in degC"=nan, "Fisf Tmag in degC"=nan, "IIR Tmag in degC"=nan}, "DDM_Parameter"=[nan, nan, nan, nan, nan, nan, nan, nan, nan], "DDM_Parameter_status"=[FALSE, FALSE, FALSE, FALSE, FALSE, FALSE, FALSE, FALSE, FALSE], "Get_Tester_Parameter"=[nan, nan, nan, nan, nan, nan, nan], "Get_Tester_Parameter_status"=[FALSE, FALSE, FALSE, FALSE, FALSE, FALSE, FALSE], "Cal_Tester_Parameter"=[nan, nan, nan, nan, nan, nan], "BEMF_Finetune"={"eol_bemf_mp_cold_coef_c"=nan, "eol_cold_bemf_fisf_offset"=nan}, "AW_Tune"={"delta_P1"=nan, "delta_P_Setting"=nan}, "DDM_Parameter_after_Airwatts_Tune"=[nan, nan, nan, nan, nan, nan, nan, nan, nan], "Get_Tester_Parameter_after_Airwatts_Tune"=[nan, nan, nan, nan, nan, nan, nan], "Cal_Tester_Parameter_after_Airwatts_Tune"=[nan, nan, nan, nan, nan, nan], "DDM_Parameter_after_Airwatts_Finetune"=[nan, nan, nan, nan, nan, nan, nan, nan, nan], "Get_Tester_Parameter_after_Airwatts_Finetune"=[nan, nan, nan, nan, nan, nan, nan], "Cal_Tester_Parameter_after_Airwatts_Finetune"=[nan, nan, nan, nan, nan, nan], "AW_Finetune"={"delta_P2"=nan, "delta_P_Setting"=nan}, "Delta_Tmag_after_tune"={"LSI Delta in degC"=nan, "FISF Delta in degc"=nan, "LSI Tmag in degC"=nan, "Fisf Tmag in degC"=nan, "IIR Tmag in degC"=nan}, "Hot Bemf in mV"=nan, "DDM_Pressure"=nan, "Delta_Pressure"=nan, " Cold Bemf in mV"=nan, " delta Bemf"=nan, " delta p"=nan, "Delta_Pressure_status"=FALSE, " delta Bemf_status"=FALSE, "LSI Delta in degC_status"=FALSE, "FISF Delta in degc_status"=FALSE, "Max_check_derate_status_status"=FALSE, "Average_All_data"=[[nan], [nan], [nan], [nan], [nan]], "Average_Tmag_Data_status"=[FALSE, FALSE, FALSE, FALSE, FALSE], "Average_Tmag_Data_after_tune_status"=[FALSE, FALSE, FALSE, FALSE, FALSE], "Cal_Tester_Parameter_status"=[FALSE, FALSE, FALSE, FALSE, FALSE], "Cal_Tester_Parameter_status_after_Airwatts_Tune"=[FALSE, FALSE, FALSE, FALSE, FALSE], "Cal_Tester_Parameter_status_after_Airwatts_FineTune"=[FALSE, FALSE, FALSE, FALSE, FALSE]}, "Task_Detect_Calib"={"LL"={"DDM_Parameter"=[nan, nan, nan, nan, nan, nan], "DDM_Parameter_status"=[FALSE, FALSE, FALSE, FALSE, FALSE, FALSE], "Get_Tester_Parameter"=[nan, nan, nan, nan], "Get_Tester_Parameter_status"=[FALSE, FALSE, FALSE, FALSE], "Set_task_detect_A"=nan, "Set_task_detect_A_Status"=FALSE}, "HL"={"DDM_Parameter"=[nan, nan, nan, nan, nan, nan], "DDM_Parameter_status"=[FALSE, FALSE, FALSE, FALSE, FALSE, FALSE], "Get_Tester_Parameter"=[nan, nan, nan, nan], "Get_Tester_Parameter_status"=[FALSE, FALSE, FALSE, FALSE], "Set_task_detect_B"=nan, "Set_task_detect_B_Status"=FALSE}, "LH"={"DDM_Parameter"=[nan, nan, nan, nan, nan, nan], "DDM_Parameter_status"=[FALSE, FALSE, FALSE, FALSE, FALSE, FALSE], "Get_Tester_Parameter"=[nan, nan, nan, nan], "Get_Tester_Parameter_status"=[FALSE, FALSE, FALSE, FALSE], "Set_task_detect_C"=nan, "Set_task_detect_C_Status"=FALSE}, "HH"={"DDM_Parameter"=[nan, nan, nan, nan, nan, nan], "DDM_Parameter_status"=[FALSE, FALSE, FALSE, FALSE, FALSE, FALSE], "Get_Tester_Parameter"=[nan, nan, nan, nan], "Get_Tester_Parameter_status"=[FALSE, FALSE, FALSE, FALSE], "Set_task_detect_D"=nan, "Read_and_check_calibration_Status"=[FALSE, FALSE, FALSE, FALSE, FALSE, FALSE], "Set_task_detect_D_Status"=FALSE}, "Get_eol_inlet_blockage_E"=nan, "Calib_vaule"={"Get_task_detect_LL"=nan, "Get_task_detect_HL"=nan, "Get_task_detect_LH"=nan, "Get_task_detect_HH"=nan, "eol_inlet_blockage"=nan, "eol_code_bemf_temp"=nan}, "calibrated temp"=nan, "Inlet_Blockage_Calibration"={"DDM_Parameter"=[nan, nan, nan, nan, nan, nan, nan, nan, nan], "DDM_Parameter_status"=[FALSE, FALSE, FALSE, FALSE, FALSE, FALSE], "Get_Tester_Parameter"=[nan, nan, nan, nan], "Get_Tester_Parameter_status"=[FALSE, FALSE, FALSE, FALSE]}, "Get_eol_inlet_blockage_E_Status"=FALSE}, "good"={"Write_Product_TS"={"TIMESTAMP"=0, "RIG_ID"=0, "PASSMARK_ID"=0, "PASSMARK_REV"=0}, "Read_Product_TS"={"TIMESTAMP"=0, "RIG_ID"=0, "PASSMARK_ID"=0, "PASSMARK_REV"=0}, "Good_Check_Secuity_Bit_Stauts"=FALSE}} ("Data") w157] -> w94
          tunnel: w90 -> [w136 _]
          tunnel: w89 -> [w135 _]
          tunnel: w88 -> [w129 _]
          tunnel: w87 -> [w127 _]
          tunnel: w86 -> [w126 _]
          tunnel: w84 -> [w124 _]
          tunnel: [w123 w156] -> w83
          tunnel: w82 -> [w108 w156]
          tunnel: w79 -> [w118 _]
          tunnel: w77 -> [w111 _]
          tunnel: w76 -> [w109 _]
          frame False {
            (unwired) T3 {"Initialisation"={"LMT - Connect UUT (con COM)"="Skip", "LMT - Software Version (rrel)"="Skip", "LMT - Write SKU file (wskuc)"="Skip", "LMT - SKU file name"="Skip", "Connect UUT DDM"="", "Read DDM EOL Timestamp - Mode"="", "Read DDM EOL Timestamp - Timestamp"="", "Read DDM EOL Timestamp - Rig ID"="", "Read DDM EOL Timestamp - Passmark ID"="", "Read DDM EOL Timestamp - Passmark Rev"="", "Software Version before flashing"="", "Read Hardware Serial"="", "UUT DDM SN"="", "Compare DDM SN with MES SN"="Skip", "Backup PCBA Calibration EEPROM Response - CAL"="Skip", "Flash Firmware Version"="", "Check SW Version"="", "Read DDM SW Version after flashing"="", "Set SKU Config"="", "Ready Status"="Skip", "Set Device Mode to EOL"="", "DDM Parameter - Voltage"="", "DDM Parameter - Current"="", "DDM Parameter - Power"="", "DDM Parameter - Speed"="", "DDM Parameter - Pressure"="", "Tester Parameter - Voltage"="", "Tester Parameter - Current"="", "Tester Parameter - Power"="", "Tester Parameter - Ambient Pressure"="", "Tester Parameter - Ambient Temperature"="", "Calculated Parameter - DDM Pressure Corrected"="", "Calculated Parameter - DDM Real Power"="", "Calculated Parameter - Delta V"=""}, "BEMF_Calibration"={"Calibration Result - eol_cold_bemf_temp"="", "DDM Ambient Temp"="Skip", "Restriction Plate Diameter"="Skip", "Calibration Result - eol_bemf_mp_cold_coef_a"="", "Calibration Result - eol_bemf_mp_cold_coef_b"="", "Calibration Result - eol_bemf_mp_cold_coef_c"="", "Calibration Result - eol_bemf_lsi_cold_ref_coeffs"="", "Get - Calibration Result - eol_bemf_lsi_speed"="", "Get - Calibration Result - eol_bemf_lsi_integral_0"="", "Calibration Result - eol_bemf_lsi_integral_1"="", "Get - Calibration Result - eol_bemf_lsi_integral_2"="", "Get - Calibration Result - eol_cold_bemf"="", "Get - Calibration Result - eol_cold_bemf_fisf"="", "Finalise Calibration"="Skip", "Compare -Calibration Result - eol_cold_bemf"="", "Compare -Calibration Result - eol_cold_bemf_fisf"=""}, "ECO"={"Reset Power Tune"="", "Reset BEMF FISF Calibration"="", "Restriction Plate Diameter"="", "ECO - Stabilisation Time"="", "ECO - DDM Parameter - Voltage"="", "ECO - DDM Parameter - Current"="", "ECO - DDM Parameter - Power"="", "ECO - DDM Parameter - Measured Power"="", "ECO - DDM Parameter - Speed"="", "ECO - DDM Parameter - Pressure"="", "ECO - Tester Parameter - Voltage"="", "ECO - Tester Parameter - Current"="", "ECO - Tester Parameter - Power"="", "ECO - Tester Parameter - Ambient Pressure"="", "ECO - Tester Parameter - Ambient Temperature"="", "ECO - Tester Parameter - Ambient Humidity"="", "ECO - Calculated Parameter - DDM Pressure Corrected"="", "ECO - Calculated Parameter - DDM Real Power"="", "ECO - Calculated Parameter - Delta V"="", "ECO - Calculated Parameter - Flowrate"="", "ECO - Calculated Parameter - Airwatt"="", "ECO - Formula"="", "PT ECO - Power Tune Mode Status"="Skip"}, "BOOST"={"Restriction Plate Diameter"="", "BOOST - Stabilisation Time"="", "BOOST - DDM Parameter - Voltage"="", "BOOST - DDM Parameter - Current"="", "BOOST - DDM Parameter - Power"="", "BOOST - DDM Parameter - Measured Power"="", "BOOST - DDM Parameter - Speed"="", "BOOST - DDM Parameter - Pressure"="", "BOOST - Tester Parameter - Voltage"="", "BOOST - Tester Parameter - Current"="", "BOOST - Tester Parameter - Power"="", "BOOST - Tester Parameter - Ambient Pressure"="", "BOOST - Tester Parameter - Ambient Temperature"="", "BOOST - Tester Parameter - Ambient Humidity"="", "BOOST - Calculated Parameter - DDM Pressure Corrected"="", "BOOST - Calculated Parameter - DDM Real Power"="", "BOOST - Calculated Parameter - Delta V"="", "BOOST - Calculated Parameter - Flowrate"="", "BOOST - Calculated Parameter - Airwatt"="", "BOOST - Get AM Presence"="", "Air Muscle Turn Off Status"="", "BOOST - Air Muscle Calculated Parameter - Airwatt B"="", "BOOST - Air Muscle Calculate Airwatt Delta"="", "PT BOOST - Power Tune Mode Status"="Skip", "Finalise Calibration"="Skip", "ECO - Get AW Calibration value"="", "BOOST - Get AW Calibration value"=""}, "MAX"={"Restriction Plate Diameter"="", "MAX - Stabilisation Time"="", "Get Average Delta Tmag (LSIdelta_FISFdelta_LSItmag_FISFtmag_IIRtmag)"="", "Get Average Delta Tmag FISF"="", "MAX - DDM Parameter - Voltage"="", "MAX - DDM Parameter - Current"="", "MAX - DDM Parameter - Power"="", "MAX - DDM Parameter - Measured Power"="", "MAX - DDM Parameter - Speed"="", "MAX - DDM Parameter - Pressure"="", "MAX - Tester Parameter - Voltage"="", "MAX - Tester Parameter - Current"="", "MAX - Tester Parameter - Power"="", "MAX - Tester Parameter - Ambient Pressure"="", "MAX - Tester Parameter - Ambient Temperature"="", "MAX - Tester Parameter - Ambient Humidity"="", "MAX - Calculated Parameter - DDM Pressure Corrected"="", "MAX - Calculated Parameter - DDM Real Power"="", "MAX - Calculated Parameter - Delta V"="", "MAX - Calculated Parameter - Flowrate"="", "MAX - Calculated Parameter - Airwatt"="", "MAX_FISF_Check_Average_Delta_Tmag"="", "MAX - FISF - BEMF Finetune Result"="No BEMF Finetune Required", "MAX tune - Delta P1"="No AW tune required", "MAX tune - Calculated Parameter - Airwatt"="", "Calculate Delta Airwatts - MAX finetune - Delta P2"="No AW finetune required", "MAX finetune - DDM Parameter - Voltage"="", "MAX finetune - DDM Parameter - Current"="", "MAX finetune - DDM Parameter - Power"="", "MAX finetune - DDM Parameter - Measured Power"="", "MAX finetune - DDM Parameter - Speed"="", "MAX finetune - DDM Parameter - Pressure"="", "MAX finetune - Tester Parameter - Voltage"="", "MAX finetune - Tester Parameter - Current"="", "MAX finetune - Tester Parameter - Power"="", "MAX finetune - Tester Parameter - Ambient Pressure"="", "MAX finetune - Tester Parameter - Ambient Temperature"="", "MAX finetune - Tester Parameter - Ambient Humidity"="", "MAX finetune - Calculated Parameter - DDM Pressure Corrected"="", "MAX finetune - Calculated Parameter - DDM Real Power"="", "MAX finetune - Calculated Parameter - Delta V"="", "MAX finetune - Calculated Parameter - Flowrate"="", "MAX finetune - Calculated Parameter - Airwatt"="", "Check Derate Result"="", "Delta Tmag FISF"="", "Get Hot BEMF Result"="", "Calculate delta Pressure"="", "Finalise Calibration"="Skip", "Calculate & Check Delta BEMF"="", "Delta P Airwatts Value"=""}, "LL"={"DDM Ambient Temp"="", "Restriction Plate Diameter"="", "LL - DDM Parameter - Voltage"="", "LL - DDM Parameter - Current"="", "LL - DDM Parameter - Power"="", "LL - DDM Parameter - Measured Power"="", "LL - DDM Parameter - Speed"="", "LL - DDM Parameter - Pressure"="", "LL - Tester Parameter - Voltage"="", "LL - Tester Parameter - Current"="", "LL - Tester Parameter - Power"="", "LL - DDM Real Power"="", "LL - Calibrate Task Detect LL"=""}, "HL"={"HL - DDM Parameter - Voltage"="", "HL - DDM Parameter - Current"="", "HL - DDM Parameter - Power"="", "HL - DDM Parameter - Measured Power"="", "HL - DDM Parameter - Speed"="", "HL - DDM Parameter - Pressure"="", "HL - Tester Parameter - Voltage"="", "HL - Tester Parameter - Current"="", "HL - Tester Parameter - Power"="", "HL - DDM Real Power"="", "HL - Calibrate Task Detect HL"=""}, "LH"={"Restriction Plate Diameter"="", "LH - DDM Parameter - Voltage"="", "LH - DDM Parameter - Current"="", "LH - DDM Parameter - Power"="", "LH - DDM Parameter - Measured Power"="", "LH - DDM Parameter - Speed"="", "LH - DDM Parameter - Pressure"="", "LH - Tester Parameter - Voltage"="", "LH - Tester Parameter - Current"="", "LH - Tester Parameter - Power"="", "LH - DDM Real Power"="", "LH - Calibrate Task Detect LH"=""}, "HH"={"HH - DDM Parameter - Voltage"="", "HH - DDM Parameter - Current"="", "HH - DDM Parameter - Power"="", "HH - DDM Parameter - Measured Power"="", "HH - DDM Parameter - Speed"="", "HH - DDM Parameter - Pressure"="", "HH - Tester Parameter - Voltage"="", "HH - Tester Parameter - Current"="", "HH - Tester Parameter - Power"="", "HH - DDM Real Power"="", "HH - Calibrate Task Detect HH"=""}, "Inlet Blockage Calibration"={"Inlet Blockage Calibration - DDM Parameter - Voltage"="", "Inlet Blockage Calibration - DDM Parameter - Current"="", "Inlet Blockage Calibration - DDM Parameter - Power"="", "Inlet Blockage Calibration - DDM Parameter - Measured Power"="", "Inlet Blockage Calibration - DDM Parameter - Speed"="", "Inlet Blockage Calibration - DDM Parameter - Pressure"="", "Inlet Blockage Calibration - Tester Parameter - Voltage"="", "Inlet Blockage Calibration - Tester Parameter - Current"="", "Inlet Blockage Calibration - Tester Parameter - Power"="", "Inlet Blockage Calibration - DDM Real Power"="", "Calibration Inlet Blockage_E"="", "Finalise Calibration"="Skip", "Get Task Detect LL"="", "Get Task Detect HL"="", "Get Task Detect LH"="", "Get Task Detect HH"="", "Calibration Inlet Blockage"="", "Calibration eol cold bemf temp"=""}, "GOOD"={"GOOD UNIT - Clear EEPROM Error Log"="", "GOOD UNIT - Write Product Timestamp - Mode"="", "GOOD UNIT - Write Product Timestamp - Timestamp"="", "GOOD UNIT - Write Product Timestamp - Rig ID"="", "GOOD UNIT - Write Product Timestamp - Passmark ID"="", "GOOD UNIT - Write Product Timestamp - Passmark Rev"="", "GOOD UNIT - Set Device Mode to PROD"="", "GOOD UNIT - Backup PCBA Calibration EEPROM Response"="", "GOOD UNIT - Check Security Bit"="", "GOOD UNIT - Set Calibration Lock"="", "GOOD UNIT - Get_Calibration_Lock"="", "GOOD UNIT - Disconnect UUT"=""}, "NG"={"NG UNIT - Read NVM Error"="", "NG UNIT - Set Device Mode to FCT"="", "NG UNIT - Backup PCBA Calibration EEPROM Response - CAL"="", "NG UNIT - Backup PCBA Calibration EEPROM Response - ERROR"="", "NG UNIT - Backup PCBA Calibration EEPROM Response - USAGE"="", "NG UNIT - Disconnect UUT"=""}, "SN"="", "Table"=[], "Count"={"Total"=0, "OK"=0, "NG"=0, "Yield"=0.0}, "Start Time"=timestamp(0 s since 1904-01-01), "daemon reference"=refnum, "CT"=0.0, "Config"=[], "OK/NG"=FALSE, "Station ID"="", "MES DDM SN"="Skip", "MES PCBA SN"="", "Retest"="Skip", "Lux"="", "Initialisation_Status"={"LMT - Connect UUT (con COM)"="", "LMT - Software Version (rrel)"="", "LMT - Write SKU file (wskuc)"="", "LMT - SKU file name"="", "Connect UUT DDM"="", "Read DDM EOL Timestamp - Mode"="", "Read DDM EOL Timestamp - Timestamp"="", "Read DDM EOL Timestamp - Rig ID"="", "Read DDM EOL Timestamp - Passmark ID"="", "Read DDM EOL Timestamp - Passmark Rev"="", "Software Version before flashing"="", "Read Hardware Serial"="", "UUT DDM SN"="", "Compare DDM SN with MES SN"="", "Backup PCBA Calibration EEPROM Response - CAL"="", "Flash Firmware Version"="", "Check SW Version"="", "Read DDM SW Version after flashing"="", "Set SKU Config"="", "Ready Status"="", "Set Device Mode to EOL"="", "DDM Parameter - Voltage"="", "DDM Parameter - Current"="", "DDM Parameter - Power"="", "DDM Parameter - Speed"="", "DDM Parameter - Pressure"="", "Tester Parameter - Voltage"="", "Tester Parameter - Current"="", "Tester Parameter - Power"="", "Tester Parameter - Ambient Pressure"="", "Tester Parameter - Ambient Temperature"="", "Calculated Parameter - DDM Pressure Corrected"="", "Calculated Parameter - DDM Real Power"="", "Calculated Parameter - Delta V"=""}, "BEMF_Calibration_Status"={"Calibration Result - eol_cold_bemf_temp"="", "DDM Ambient Temp"="", "Restriction Plate Diameter"="", "Calibration Result - eol_bemf_mp_cold_coef_a"="", "Calibration Result - eol_bemf_mp_cold_coef_b"="", "Calibration Result - eol_bemf_mp_cold_coef_c"="", "Calibration Result - eol_bemf_lsi_cold_ref_coeffs"="", "Get - Calibration Result - eol_bemf_lsi_speed"="", "Get - Calibration Result - eol_bemf_lsi_integral_0"="", "Calibration Result - eol_bemf_lsi_integral_1"="", "Get - Calibration Result - eol_bemf_lsi_integral_2"="", "Get - Calibration Result - eol_cold_bemf"="", "Get - Calibration Result - eol_cold_bemf_fisf"="", "Finalise Calibration"="", "Compare -Calibration Result - eol_cold_bemf"="", "Compare -Calibration Result - eol_cold_bemf_fisf"=""}, "ECO_Status"={"Reset Power Tune"="", "Reset BEMF FISF Calibration"="", "Restriction Plate Diameter"="", "ECO - Stabilisation Time"="", "ECO - DDM Parameter - Voltage"="", "ECO - DDM Parameter - Current"="", "ECO - DDM Parameter - Power"="", "ECO - DDM Parameter - Measured Power"="", "ECO - DDM Parameter - Speed"="", "ECO - DDM Parameter - Pressure"="", "ECO - Tester Parameter - Voltage"="", "ECO - Tester Parameter - Current"="", "ECO - Tester Parameter - Power"="", "ECO - Tester Parameter - Ambient Pressure"="", "ECO - Tester Parameter - Ambient Temperature"="", "ECO - Tester Parameter - Ambient Humidity"="", "ECO - Calculated Parameter - DDM Pressure Corrected"="", "ECO - Calculated Parameter - DDM Real Power"="", "ECO - Calculated Parameter - Delta V"="", "ECO - Calculated Parameter - Flowrate"="", "ECO - Calculated Parameter - Airwatt"="", "ECO - Formula"="", "PT ECO - Power Tune Mode Status"=""}, "BOOST_Status"={"Restriction Plate Diameter"="", "BOOST - Stabilisation Time"="", "BOOST - DDM Parameter - Voltage"="", "BOOST - DDM Parameter - Current"="", "BOOST - DDM Parameter - Power"="", "BOOST - DDM Parameter - Measured Power"="", "BOOST - DDM Parameter - Speed"="", "BOOST - DDM Parameter - Pressure"="", "BOOST - Tester Parameter - Voltage"="", "BOOST - Tester Parameter - Current"="", "BOOST - Tester Parameter - Power"="", "BOOST - Tester Parameter - Ambient Pressure"="", "BOOST - Tester Parameter - Ambient Temperature"="", "BOOST - Tester Parameter - Ambient Humidity"="", "BOOST - Calculated Parameter - DDM Pressure Corrected"="", "BOOST - Calculated Parameter - DDM Real Power"="", "BOOST - Calculated Parameter - Delta V"="", "BOOST - Calculated Parameter - Flowrate"="", "BOOST - Calculated Parameter - Airwatt"="", "BOOST - Get AM Presence"="", "Air Muscle Turn Off Status"="", "BOOST - Air Muscle Calculated Parameter - Airwatt B"="", "BOOST - Air Muscle Calculate Airwatt Delta"="", "PT BOOST - Power Tune Mode Status"="", "Finalise Calibration"="", "ECO - Get AW Calibration value"="", "BOOST - Get AW Calibration value"=""}, "MAX_Status"={"Restriction Plate Diameter"="", "MAX - Stabilisation Time"="", "Get Average Delta Tmag (LSIdelta_FISFdelta_LSItmag_FISFtmag_IIRtmag)"="", "Get Average Delta Tmag FISF"="", "MAX - DDM Parameter - Voltage"="", "MAX - DDM Parameter - Current"="", "MAX - DDM Parameter - Power"="", "MAX - DDM Parameter - Measured Power"="", "MAX - DDM Parameter - Speed"="", "MAX - DDM Parameter - Pressure"="", "MAX - Tester Parameter - Voltage"="", "MAX - Tester Parameter - Current"="", "MAX - Tester Parameter - Power"="", "MAX - Tester Parameter - Ambient Pressure"="", "MAX - Tester Parameter - Ambient Temperature"="", "MAX - Tester Parameter - Ambient Humidity"="", "MAX - Calculated Parameter - DDM Pressure Corrected"="", "MAX - Calculated Parameter - DDM Real Power"="", "MAX - Calculated Parameter - Delta V"="", "MAX - Calculated Parameter - Flowrate"="", "MAX - Calculated Parameter - Airwatt"="", "MAX_FISF_Check_Average_Delta_Tmag"="", "MAX - FISF - BEMF Finetune Result"="", "MAX tune - Delta P1"="", "MAX tune - Calculated Parameter - Airwatt"="", "Calculate Delta Airwatts - MAX finetune - Delta P2"="", "MAX finetune - DDM Parameter - Voltage"="", "MAX finetune - DDM Parameter - Current"="", "MAX finetune - DDM Parameter - Power"="", "MAX finetune - DDM Parameter - Measured Power"="", "MAX finetune - DDM Parameter - Speed"="", "MAX finetune - DDM Parameter - Pressure"="", "MAX finetune - Tester Parameter - Voltage"="", "MAX finetune - Tester Parameter - Current"="", "MAX finetune - Tester Parameter - Power"="", "MAX finetune - Tester Parameter - Ambient Pressure"="", "MAX finetune - Tester Parameter - Ambient Temperature"="", "MAX finetune - Tester Parameter - Ambient Humidity"="", "MAX finetune - Calculated Parameter - DDM Pressure Corrected"="", "MAX finetune - Calculated Parameter - DDM Real Power"="", "MAX finetune - Calculated Parameter - Delta V"="", "MAX finetune - Calculated Parameter - Flowrate"="", "MAX finetune - Calculated Parameter - Airwatt"="", "Check Derate Result"="", "Delta Tmag FISF"="", "Get Hot BEMF Result"="", "Calculate delta Pressure"="", "Finalise Calibration"="", "Calculate & Check Delta BEMF"="", "Delta P Airwatts Value"=""}, "LL_Status"={"DDM Ambient Temp"="", "Restriction Plate Diameter"="", "LL - DDM Parameter - Voltage"="", "LL - DDM Parameter - Current"="", "LL - DDM Parameter - Power"="", "LL - DDM Parameter - Measured Power"="", "LL - DDM Parameter - Speed"="", "LL - DDM Parameter - Pressure"="", "LL - Tester Parameter - Voltage"="", "LL - Tester Parameter - Current"="", "LL - Tester Parameter - Power"="", "LL - DDM Real Power"="", "LL - Calibrate Task Detect LL"=""}, "HL_Status"={"HL - DDM Parameter - Voltage"="", "HL - DDM Parameter - Current"="", "HL - DDM Parameter - Power"="", "HL - DDM Parameter - Measured Power"="", "HL - DDM Parameter - Speed"="", "HL - DDM Parameter - Pressure"="", "HL - Tester Parameter - Voltage"="", "HL - Tester Parameter - Current"="", "HL - Tester Parameter - Power"="", "HL - DDM Real Power"="", "HL - Calibrate Task Detect HL"=""}, "LH_Status"={"Restriction Plate Diameter"="", "LH - DDM Parameter - Voltage"="", "LH - DDM Parameter - Current"="", "LH - DDM Parameter - Power"="", "LH - DDM Parameter - Measured Power"="", "LH - DDM Parameter - Speed"="", "LH - DDM Parameter - Pressure"="", "LH - Tester Parameter - Voltage"="", "LH - Tester Parameter - Current"="", "LH - Tester Parameter - Power"="", "LH - DDM Real Power"="", "LH - Calibrate Task Detect LH"=""}, "HH_Status"={"HH - DDM Parameter - Voltage"="", "HH - DDM Parameter - Current"="", "HH - DDM Parameter - Power"="", "HH - DDM Parameter - Measured Power"="", "HH - DDM Parameter - Speed"="", "HH - DDM Parameter - Pressure"="", "HH - Tester Parameter - Voltage"="", "HH - Tester Parameter - Current"="", "HH - Tester Parameter - Power"="", "HH - DDM Real Power"="", "HH - Calibrate Task Detect HH"=""}, "Inlet Blockage Calibration_Status"={"Inlet Blockage Calibration - DDM Parameter - Voltage"="", "Inlet Blockage Calibration - DDM Parameter - Current"="", "Inlet Blockage Calibration - DDM Parameter - Power"="", "Inlet Blockage Calibration - DDM Parameter - Measured Power"="", "Inlet Blockage Calibration - DDM Parameter - Speed"="", "Inlet Blockage Calibration - DDM Parameter - Pressure"="", "Inlet Blockage Calibration - Tester Parameter - Voltage"="", "Inlet Blockage Calibration - Tester Parameter - Current"="", "Inlet Blockage Calibration - Tester Parameter - Power"="", "Inlet Blockage Calibration - DDM Real Power"="", "Calibration Inlet Blockage_E"="", "Finalise Calibration"="", "Get Task Detect LL"="", "Get Task Detect HL"="", "Get Task Detect LH"="", "Get Task Detect HH"="", "Calibration Inlet Blockage"="", "Calibration eol cold bemf temp"=""}, "GOOD_Status"={"GOOD UNIT - Clear EEPROM Error Log"="", "GOOD UNIT - Write Product Timestamp - Mode"="", "GOOD UNIT - Write Product Timestamp - Timestamp"="", "GOOD UNIT - Write Product Timestamp - Rig ID"="", "GOOD UNIT - Write Product Timestamp - Passmark ID"="", "GOOD UNIT - Write Product Timestamp - Passmark Rev"="", "GOOD UNIT - Set Device Mode to PROD"="", "GOOD UNIT - Backup PCBA Calibration EEPROM Response"="", "GOOD UNIT - Check Security Bit"="", "GOOD UNIT - Set Calibration Lock"="", "GOOD UNIT - Get_Calibration_Lock"="", "GOOD UNIT - Disconnect UUT"=""}, "NG_Status"={"NG UNIT - Read NVM Error"="", "NG UNIT - Set Device Mode to FCT"="", "NG UNIT - Backup PCBA Calibration EEPROM Response - CAL"="", "NG UNIT - Backup PCBA Calibration EEPROM Response - ERROR"="", "NG UNIT - Backup PCBA Calibration EEPROM Response - USAGE"="", "NG UNIT - Disconnect UUT"=""}, "SKU"="", "Plate_Diameter"="", "Alarm"=""} ("Data in")
            n26 = case shown="假" w111 {
              tunnel: [w146 w154] -> w121
              tunnel: [w144 w153] -> w110
              tunnel: w109 -> [w143 _]
              tunnel: w108 -> [_ w155]
              frame False {
                n27 = call "TableData.vi"("Step"=enum16{"Initial", "Write", "Read"}."Read") -> ("Tabledata Out"=w147:string[][])  [unwired: 9 in, 1 out]
                n28 = call "ConfigData.vi"("Step"=enum16{"Initial", "Write", "Read"}."Read") -> ("Tabledata Out"=w144:string[][])  [unwired: 9 in, 1 out]
                n29 = Delete From Array(array=w147, length=1 ("长度"), index (row)=0 ("索引 (行)")) -> (deleted portion=w148:string[][], array with subset deleted=w149:string[][])  [unwired: 1 in]
                n30 = call "Select_UUT_Table.vi"("all Title"=w148, "all Table"=w149) -> ("Title"=w142:string[], "Table"=w146:string[][])  [unwired: 8 in]
                n31 = property class="Tbl (strict)"(reference=w143, "Column Headers[]"=w142) -> ()  [unwired: 1 in, 2 out]
              }
              frame True {
                n32 = Unbundle By Name(w155) -> ("Table"=w154:string[][], "Config"=w153:string[][])
              }
            }
            n33 = property class="Str"(reference=w135, "Value"="" ("值"), "Blinking"=FALSE ("闪烁")) -> ()  [unwired: 1 in, 2 out]
            n34 = call "StatusLamp.vi"("State"="StandBy", "Boolean输入"=w127) -> ()  [unwired: 9 in, 1 out]
            n35 = property class="DigNum (strict)"(reference=w126, "Value"=0.0) -> ()  [unwired: 1 in, 2 out]
            n36 = property class="Str"(reference=w139, "Key Focus"=FALSE, "DisabledEnum"=T9."Disabled" ("Disabled")) -> ()  [unwired: 1 in, 2 out]
            n37 = property class="Tbl (strict)"(reference=w129, "Value"=string[][] [] ("值"), "Active Cell"=T8 {"Row"=-2, "Column"=-2} ("活动单元格:活动单元格"), "Cell BG Color"=u32 3421236, "Row Headers[]"=string[] [] ("Row Header Strings[]")) -> ()  [unwired: 1 in, 2 out]
            n38 = call "Get StationID.vi"("路径"=w124) -> ("Station ID"=w120:string)  [unwired: 10 in]
            n39 = Unbundle By Name(w108) -> ("Count"=w115:T7, "daemon reference"=w114:refnum<k5>)
            n40 = Select(t="MES_Verification", s=w136, f="Check_Carrier_Sensor_Signal") -> (s? t:f=w119:string)
            n41 = Bundle By Name(cluster=T3 {"Initialisation"={"LMT - Connect UUT (con COM)"="", "LMT - Software Version (rrel)"="", "LMT - Write SKU file (wskuc)"="", "LMT - SKU file name"="", "Connect UUT DDM"="", "Read DDM EOL Timestamp - Mode"="", "Read DDM EOL Timestamp - Timestamp"="", "Read DDM EOL Timestamp - Rig ID"="", "Read DDM EOL Timestamp - Passmark ID"="", "Read DDM EOL Timestamp - Passmark Rev"="", "Software Version before flashing"="", "Read Hardware Serial"="", "UUT DDM SN"="", "Compare DDM SN with MES SN"="", "Backup PCBA Calibration EEPROM Response - CAL"="", "Flash Firmware Version"="", "Check SW Version"="", "Read DDM SW Version after flashing"="", "Set SKU Config"="", "Ready Status"="", "Set Device Mode to EOL"="", "DDM Parameter - Voltage"="", "DDM Parameter - Current"="", "DDM Parameter - Power"="", "DDM Parameter - Speed"="", "DDM Parameter - Pressure"="", "Tester Parameter - Voltage"="", "Tester Parameter - Current"="", "Tester Parameter - Power"="", "Tester Parameter - Ambient Pressure"="", "Tester Parameter - Ambient Temperature"="", "Calculated Parameter - DDM Pressure Corrected"="", "Calculated Parameter - DDM Real Power"="", "Calculated Parameter - Delta V"=""}, "BEMF_Calibration"={"Calibration Result - eol_cold_bemf_temp"="", "DDM Ambient Temp"="", "Restriction Plate Diameter"="", "Calibration Result - eol_bemf_mp_cold_coef_a"="", "Calibration Result - eol_bemf_mp_cold_coef_b"="", "Calibration Result - eol_bemf_mp_cold_coef_c"="", "Calibration Result - eol_bemf_lsi_cold_ref_coeffs"="", "Get - Calibration Result - eol_bemf_lsi_speed"="", "Get - Calibration Result - eol_bemf_lsi_integral_0"="", "Calibration Result - eol_bemf_lsi_integral_1"="", "Get - Calibration Result - eol_bemf_lsi_integral_2"="", "Get - Calibration Result - eol_cold_bemf"="", "Get - Calibration Result - eol_cold_bemf_fisf"="", "Finalise Calibration"="", "Compare -Calibration Result - eol_cold_bemf"="", "Compare -Calibration Result - eol_cold_bemf_fisf"=""}, "ECO"={"Reset Power Tune"="", "Reset BEMF FISF Calibration"="", "Restriction Plate Diameter"="", "ECO - Stabilisation Time"="", "ECO - DDM Parameter - Voltage"="", "ECO - DDM Parameter - Current"="", "ECO - DDM Parameter - Power"="", "ECO - DDM Parameter - Measured Power"="", "ECO - DDM Parameter - Speed"="", "ECO - DDM Parameter - Pressure"="", "ECO - Tester Parameter - Voltage"="", "ECO - Tester Parameter - Current"="", "ECO - Tester Parameter - Power"="", "ECO - Tester Parameter - Ambient Pressure"="", "ECO - Tester Parameter - Ambient Temperature"="", "ECO - Tester Parameter - Ambient Humidity"="", "ECO - Calculated Parameter - DDM Pressure Corrected"="", "ECO - Calculated Parameter - DDM Real Power"="", "ECO - Calculated Parameter - Delta V"="", "ECO - Calculated Parameter - Flowrate"="", "ECO - Calculated Parameter - Airwatt"="", "ECO - Formula"="", "PT ECO - Power Tune Mode Status"=""}, "BOOST"={"Restriction Plate Diameter"="", "BOOST - Stabilisation Time"="", "BOOST - DDM Parameter - Voltage"="", "BOOST - DDM Parameter - Current"="", "BOOST - DDM Parameter - Power"="", "BOOST - DDM Parameter - Measured Power"="", "BOOST - DDM Parameter - Speed"="", "BOOST - DDM Parameter - Pressure"="", "BOOST - Tester Parameter - Voltage"="", "BOOST - Tester Parameter - Current"="", "BOOST - Tester Parameter - Power"="", "BOOST - Tester Parameter - Ambient Pressure"="", "BOOST - Tester Parameter - Ambient Temperature"="", "BOOST - Tester Parameter - Ambient Humidity"="", "BOOST - Calculated Parameter - DDM Pressure Corrected"="", "BOOST - Calculated Parameter - DDM Real Power"="", "BOOST - Calculated Parameter - Delta V"="", "BOOST - Calculated Parameter - Flowrate"="", "BOOST - Calculated Parameter - Airwatt"="", "BOOST - Get AM Presence"="", "Air Muscle Turn Off Status"="", "BOOST - Air Muscle Calculated Parameter - Airwatt B"="", "BOOST - Air Muscle Calculate Airwatt Delta"="", "PT BOOST - Power Tune Mode Status"="", "Finalise Calibration"="", "ECO - Get AW Calibration value"="", "BOOST - Get AW Calibration value"=""}, "MAX"={"Restriction Plate Diameter"="", "MAX - Stabilisation Time"="", "Get Average Delta Tmag (LSIdelta_FISFdelta_LSItmag_FISFtmag_IIRtmag)"="", "Get Average Delta Tmag FISF"="", "MAX - DDM Parameter - Voltage"="", "MAX - DDM Parameter - Current"="", "MAX - DDM Parameter - Power"="", "MAX - DDM Parameter - Measured Power"="", "MAX - DDM Parameter - Speed"="", "MAX - DDM Parameter - Pressure"="", "MAX - Tester Parameter - Voltage"="", "MAX - Tester Parameter - Current"="", "MAX - Tester Parameter - Power"="", "MAX - Tester Parameter - Ambient Pressure"="", "MAX - Tester Parameter - Ambient Temperature"="", "MAX - Tester Parameter - Ambient Humidity"="", "MAX - Calculated Parameter - DDM Pressure Corrected"="", "MAX - Calculated Parameter - DDM Real Power"="", "MAX - Calculated Parameter - Delta V"="", "MAX - Calculated Parameter - Flowrate"="", "MAX - Calculated Parameter - Airwatt"="", "MAX_FISF_Check_Average_Delta_Tmag"="", "MAX - FISF - BEMF Finetune Result"="", "MAX tune - Delta P1"="", "MAX tune - Calculated Parameter - Airwatt"="", "Calculate Delta Airwatts - MAX finetune - Delta P2"="", "MAX finetune - DDM Parameter - Voltage"="", "MAX finetune - DDM Parameter - Current"="", "MAX finetune - DDM Parameter - Power"="", "MAX finetune - DDM Parameter - Measured Power"="", "MAX finetune - DDM Parameter - Speed"="", "MAX finetune - DDM Parameter - Pressure"="", "MAX finetune - Tester Parameter - Voltage"="", "MAX finetune - Tester Parameter - Current"="", "MAX finetune - Tester Parameter - Power"="", "MAX finetune - Tester Parameter - Ambient Pressure"="", "MAX finetune - Tester Parameter - Ambient Temperature"="", "MAX finetune - Tester Parameter - Ambient Humidity"="", "MAX finetune - Calculated Parameter - DDM Pressure Corrected"="", "MAX finetune - Calculated Parameter - DDM Real Power"="", "MAX finetune - Calculated Parameter - Delta V"="", "MAX finetune - Calculated Parameter - Flowrate"="", "MAX finetune - Calculated Parameter - Airwatt"="", "Check Derate Result"="", "Delta Tmag FISF"="", "Get Hot BEMF Result"="", "Calculate delta Pressure"="", "Finalise Calibration"="", "Calculate & Check Delta BEMF"="", "Delta P Airwatts Value"=""}, "LL"={"DDM Ambient Temp"="", "Restriction Plate Diameter"="", "LL - DDM Parameter - Voltage"="", "LL - DDM Parameter - Current"="", "LL - DDM Parameter - Power"="", "LL - DDM Parameter - Measured Power"="", "LL - DDM Parameter - Speed"="", "LL - DDM Parameter - Pressure"="", "LL - Tester Parameter - Voltage"="", "LL - Tester Parameter - Current"="", "LL - Tester Parameter - Power"="", "LL - DDM Real Power"="", "LL - Calibrate Task Detect LL"=""}, "HL"={"HL - DDM Parameter - Voltage"="", "HL - DDM Parameter - Current"="", "HL - DDM Parameter - Power"="", "HL - DDM Parameter - Measured Power"="", "HL - DDM Parameter - Speed"="", "HL - DDM Parameter - Pressure"="", "HL - Tester Parameter - Voltage"="", "HL - Tester Parameter - Current"="", "HL - Tester Parameter - Power"="", "HL - DDM Real Power"="", "HL - Calibrate Task Detect HL"=""}, "LH"={"Restriction Plate Diameter"="", "LH - DDM Parameter - Voltage"="", "LH - DDM Parameter - Current"="", "LH - DDM Parameter - Power"="", "LH - DDM Parameter - Measured Power"="", "LH - DDM Parameter - Speed"="", "LH - DDM Parameter - Pressure"="", "LH - Tester Parameter - Voltage"="", "LH - Tester Parameter - Current"="", "LH - Tester Parameter - Power"="", "LH - DDM Real Power"="", "LH - Calibrate Task Detect LH"=""}, "HH"={"HH - DDM Parameter - Voltage"="", "HH - DDM Parameter - Current"="", "HH - DDM Parameter - Power"="", "HH - DDM Parameter - Measured Power"="", "HH - DDM Parameter - Speed"="", "HH - DDM Parameter - Pressure"="", "HH - Tester Parameter - Voltage"="", "HH - Tester Parameter - Current"="", "HH - Tester Parameter - Power"="", "HH - DDM Real Power"="", "HH - Calibrate Task Detect HH"=""}, "Inlet Blockage Calibration"={"Inlet Blockage Calibration - DDM Parameter - Voltage"="", "Inlet Blockage Calibration - DDM Parameter - Current"="", "Inlet Blockage Calibration - DDM Parameter - Power"="", "Inlet Blockage Calibration - DDM Parameter - Measured Power"="", "Inlet Blockage Calibration - DDM Parameter - Speed"="", "Inlet Blockage Calibration - DDM Parameter - Pressure"="", "Inlet Blockage Calibration - Tester Parameter - Voltage"="", "Inlet Blockage Calibration - Tester Parameter - Current"="", "Inlet Blockage Calibration - Tester Parameter - Power"="", "Inlet Blockage Calibration - DDM Real Power"="", "Calibration Inlet Blockage_E"="", "Finalise Calibration"="", "Get Task Detect LL"="", "Get Task Detect HL"="", "Get Task Detect LH"="", "Get Task Detect HH"="", "Calibration Inlet Blockage"="", "Calibration eol cold bemf temp"=""}, "GOOD"={"GOOD UNIT - Clear EEPROM Error Log"="", "GOOD UNIT - Write Product Timestamp - Mode"="", "GOOD UNIT - Write Product Timestamp - Timestamp"="", "GOOD UNIT - Write Product Timestamp - Rig ID"="", "GOOD UNIT - Write Product Timestamp - Passmark ID"="", "GOOD UNIT - Write Product Timestamp - Passmark Rev"="", "GOOD UNIT - Set Device Mode to PROD"="", "GOOD UNIT - Backup PCBA Calibration EEPROM Response"="", "GOOD UNIT - Check Security Bit"="", "GOOD UNIT - Set Calibration Lock"="", "GOOD UNIT - Get_Calibration_Lock"="", "GOOD UNIT - Disconnect UUT"=""}, "NG"={"NG UNIT - Read NVM Error"="", "NG UNIT - Set Device Mode to FCT"="", "NG UNIT - Backup PCBA Calibration EEPROM Response - CAL"="", "NG UNIT - Backup PCBA Calibration EEPROM Response - ERROR"="", "NG UNIT - Backup PCBA Calibration EEPROM Response - USAGE"="", "NG UNIT - Disconnect UUT"=""}, "SN"="", "Table"=[], "Count"={"Total"=0, "OK"=0, "NG"=0, "Yield"=0.0}, "Start Time"=timestamp(0 s since 1904-01-01), "daemon reference"=refnum, "CT"=0.0, "Config"=[], "OK/NG"=FALSE, "Station ID"="", "MES DDM SN"="", "MES PCBA SN"="", "Retest"="", "Lux"="", "Initialisation_Status"={"LMT - Connect UUT (con COM)"="", "LMT - Software Version (rrel)"="", "LMT - Write SKU file (wskuc)"="", "LMT - SKU file name"="", "Connect UUT DDM"="", "Read DDM EOL Timestamp - Mode"="", "Read DDM EOL Timestamp - Timestamp"="", "Read DDM EOL Timestamp - Rig ID"="", "Read DDM EOL Timestamp - Passmark ID"="", "Read DDM EOL Timestamp - Passmark Rev"="", "Software Version before flashing"="", "Read Hardware Serial"="", "UUT DDM SN"="", "Compare DDM SN with MES SN"="", "Backup PCBA Calibration EEPROM Response - CAL"="", "Flash Firmware Version"="", "Check SW Version"="", "Read DDM SW Version after flashing"="", "Set SKU Config"="", "Ready Status"="", "Set Device Mode to EOL"="", "DDM Parameter - Voltage"="", "DDM Parameter - Current"="", "DDM Parameter - Power"="", "DDM Parameter - Speed"="", "DDM Parameter - Pressure"="", "Tester Parameter - Voltage"="", "Tester Parameter - Current"="", "Tester Parameter - Power"="", "Tester Parameter - Ambient Pressure"="", "Tester Parameter - Ambient Temperature"="", "Calculated Parameter - DDM Pressure Corrected"="", "Calculated Parameter - DDM Real Power"="", "Calculated Parameter - Delta V"=""}, "BEMF_Calibration_Status"={"Calibration Result - eol_cold_bemf_temp"="", "DDM Ambient Temp"="", "Restriction Plate Diameter"="", "Calibration Result - eol_bemf_mp_cold_coef_a"="", "Calibration Result - eol_bemf_mp_cold_coef_b"="", "Calibration Result - eol_bemf_mp_cold_coef_c"="", "Calibration Result - eol_bemf_lsi_cold_ref_coeffs"="", "Get - Calibration Result - eol_bemf_lsi_speed"="", "Get - Calibration Result - eol_bemf_lsi_integral_0"="", "Calibration Result - eol_bemf_lsi_integral_1"="", "Get - Calibration Result - eol_bemf_lsi_integral_2"="", "Get - Calibration Result - eol_cold_bemf"="", "Get - Calibration Result - eol_cold_bemf_fisf"="", "Finalise Calibration"="", "Compare -Calibration Result - eol_cold_bemf"="", "Compare -Calibration Result - eol_cold_bemf_fisf"=""}, "ECO_Status"={"Reset Power Tune"="", "Reset BEMF FISF Calibration"="", "Restriction Plate Diameter"="", "ECO - Stabilisation Time"="", "ECO - DDM Parameter - Voltage"="", "ECO - DDM Parameter - Current"="", "ECO - DDM Parameter - Power"="", "ECO - DDM Parameter - Measured Power"="", "ECO - DDM Parameter - Speed"="", "ECO - DDM Parameter - Pressure"="", "ECO - Tester Parameter - Voltage"="", "ECO - Tester Parameter - Current"="", "ECO - Tester Parameter - Power"="", "ECO - Tester Parameter - Ambient Pressure"="", "ECO - Tester Parameter - Ambient Temperature"="", "ECO - Tester Parameter - Ambient Humidity"="", "ECO - Calculated Parameter - DDM Pressure Corrected"="", "ECO - Calculated Parameter - DDM Real Power"="", "ECO - Calculated Parameter - Delta V"="", "ECO - Calculated Parameter - Flowrate"="", "ECO - Calculated Parameter - Airwatt"="", "ECO - Formula"="", "PT ECO - Power Tune Mode Status"=""}, "BOOST_Status"={"Restriction Plate Diameter"="", "BOOST - Stabilisation Time"="", "BOOST - DDM Parameter - Voltage"="", "BOOST - DDM Parameter - Current"="", "BOOST - DDM Parameter - Power"="", "BOOST - DDM Parameter - Measured Power"="", "BOOST - DDM Parameter - Speed"="", "BOOST - DDM Parameter - Pressure"="", "BOOST - Tester Parameter - Voltage"="", "BOOST - Tester Parameter - Current"="", "BOOST - Tester Parameter - Power"="", "BOOST - Tester Parameter - Ambient Pressure"="", "BOOST - Tester Parameter - Ambient Temperature"="", "BOOST - Tester Parameter - Ambient Humidity"="", "BOOST - Calculated Parameter - DDM Pressure Corrected"="", "BOOST - Calculated Parameter - DDM Real Power"="", "BOOST - Calculated Parameter - Delta V"="", "BOOST - Calculated Parameter - Flowrate"="", "BOOST - Calculated Parameter - Airwatt"="", "BOOST - Get AM Presence"="", "Air Muscle Turn Off Status"="", "BOOST - Air Muscle Calculated Parameter - Airwatt B"="", "BOOST - Air Muscle Calculate Airwatt Delta"="", "PT BOOST - Power Tune Mode Status"="", "Finalise Calibration"="", "ECO - Get AW Calibration value"="", "BOOST - Get AW Calibration value"=""}, "MAX_Status"={"Restriction Plate Diameter"="", "MAX - Stabilisation Time"="", "Get Average Delta Tmag (LSIdelta_FISFdelta_LSItmag_FISFtmag_IIRtmag)"="", "Get Average Delta Tmag FISF"="", "MAX - DDM Parameter - Voltage"="", "MAX - DDM Parameter - Current"="", "MAX - DDM Parameter - Power"="", "MAX - DDM Parameter - Measured Power"="", "MAX - DDM Parameter - Speed"="", "MAX - DDM Parameter - Pressure"="", "MAX - Tester Parameter - Voltage"="", "MAX - Tester Parameter - Current"="", "MAX - Tester Parameter - Power"="", "MAX - Tester Parameter - Ambient Pressure"="", "MAX - Tester Parameter - Ambient Temperature"="", "MAX - Tester Parameter - Ambient Humidity"="", "MAX - Calculated Parameter - DDM Pressure Corrected"="", "MAX - Calculated Parameter - DDM Real Power"="", "MAX - Calculated Parameter - Delta V"="", "MAX - Calculated Parameter - Flowrate"="", "MAX - Calculated Parameter - Airwatt"="", "MAX_FISF_Check_Average_Delta_Tmag"="", "MAX - FISF - BEMF Finetune Result"="", "MAX tune - Delta P1"="", "MAX tune - Calculated Parameter - Airwatt"="", "Calculate Delta Airwatts - MAX finetune - Delta P2"="", "MAX finetune - DDM Parameter - Voltage"="", "MAX finetune - DDM Parameter - Current"="", "MAX finetune - DDM Parameter - Power"="", "MAX finetune - DDM Parameter - Measured Power"="", "MAX finetune - DDM Parameter - Speed"="", "MAX finetune - DDM Parameter - Pressure"="", "MAX finetune - Tester Parameter - Voltage"="", "MAX finetune - Tester Parameter - Current"="", "MAX finetune - Tester Parameter - Power"="", "MAX finetune - Tester Parameter - Ambient Pressure"="", "MAX finetune - Tester Parameter - Ambient Temperature"="", "MAX finetune - Tester Parameter - Ambient Humidity"="", "MAX finetune - Calculated Parameter - DDM Pressure Corrected"="", "MAX finetune - Calculated Parameter - DDM Real Power"="", "MAX finetune - Calculated Parameter - Delta V"="", "MAX finetune - Calculated Parameter - Flowrate"="", "MAX finetune - Calculated Parameter - Airwatt"="", "Check Derate Result"="", "Delta Tmag FISF"="", "Get Hot BEMF Result"="", "Calculate delta Pressure"="", "Finalise Calibration"="", "Calculate & Check Delta BEMF"="", "Delta P Airwatts Value"=""}, "LL_Status"={"DDM Ambient Temp"="", "Restriction Plate Diameter"="", "LL - DDM Parameter - Voltage"="", "LL - DDM Parameter - Current"="", "LL - DDM Parameter - Power"="", "LL - DDM Parameter - Measured Power"="", "LL - DDM Parameter - Speed"="", "LL - DDM Parameter - Pressure"="", "LL - Tester Parameter - Voltage"="", "LL - Tester Parameter - Current"="", "LL - Tester Parameter - Power"="", "LL - DDM Real Power"="", "LL - Calibrate Task Detect LL"=""}, "HL_Status"={"HL - DDM Parameter - Voltage"="", "HL - DDM Parameter - Current"="", "HL - DDM Parameter - Power"="", "HL - DDM Parameter - Measured Power"="", "HL - DDM Parameter - Speed"="", "HL - DDM Parameter - Pressure"="", "HL - Tester Parameter - Voltage"="", "HL - Tester Parameter - Current"="", "HL - Tester Parameter - Power"="", "HL - DDM Real Power"="", "HL - Calibrate Task Detect HL"=""}, "LH_Status"={"Restriction Plate Diameter"="", "LH - DDM Parameter - Voltage"="", "LH - DDM Parameter - Current"="", "LH - DDM Parameter - Power"="", "LH - DDM Parameter - Measured Power"="", "LH - DDM Parameter - Speed"="", "LH - DDM Parameter - Pressure"="", "LH - Tester Parameter - Voltage"="", "LH - Tester Parameter - Current"="", "LH - Tester Parameter - Power"="", "LH - DDM Real Power"="", "LH - Calibrate Task Detect LH"=""}, "HH_Status"={"HH - DDM Parameter - Voltage"="", "HH - DDM Parameter - Current"="", "HH - DDM Parameter - Power"="", "HH - DDM Parameter - Measured Power"="", "HH - DDM Parameter - Speed"="", "HH - DDM Parameter - Pressure"="", "HH - Tester Parameter - Voltage"="", "HH - Tester Parameter - Current"="", "HH - Tester Parameter - Power"="", "HH - DDM Real Power"="", "HH - Calibrate Task Detect HH"=""}, "Inlet Blockage Calibration_Status"={"Inlet Blockage Calibration - DDM Parameter - Voltage"="", "Inlet Blockage Calibration - DDM Parameter - Current"="", "Inlet Blockage Calibration - DDM Parameter - Power"="", "Inlet Blockage Calibration - DDM Parameter - Measured Power"="", "Inlet Blockage Calibration - DDM Parameter - Speed"="", "Inlet Blockage Calibration - DDM Parameter - Pressure"="", "Inlet Blockage Calibration - Tester Parameter - Voltage"="", "Inlet Blockage Calibration - Tester Parameter - Current"="", "Inlet Blockage Calibration - Tester Parameter - Power"="", "Inlet Blockage Calibration - DDM Real Power"="", "Calibration Inlet Blockage_E"="", "Finalise Calibration"="", "Get Task Detect LL"="", "Get Task Detect HL"="", "Get Task Detect LH"="", "Get Task Detect HH"="", "Calibration Inlet Blockage"="", "Calibration eol cold bemf temp"=""}, "GOOD_Status"={"GOOD UNIT - Clear EEPROM Error Log"="", "GOOD UNIT - Write Product Timestamp - Mode"="", "GOOD UNIT - Write Product Timestamp - Timestamp"="", "GOOD UNIT - Write Product Timestamp - Rig ID"="", "GOOD UNIT - Write Product Timestamp - Passmark ID"="", "GOOD UNIT - Write Product Timestamp - Passmark Rev"="", "GOOD UNIT - Set Device Mode to PROD"="", "GOOD UNIT - Backup PCBA Calibration EEPROM Response"="", "GOOD UNIT - Check Security Bit"="", "GOOD UNIT - Set Calibration Lock"="", "GOOD UNIT - Get_Calibration_Lock"="", "GOOD UNIT - Disconnect UUT"=""}, "NG_Status"={"NG UNIT - Read NVM Error"="", "NG UNIT - Set Device Mode to FCT"="", "NG UNIT - Backup PCBA Calibration EEPROM Response - CAL"="", "NG UNIT - Backup PCBA Calibration EEPROM Response - ERROR"="", "NG UNIT - Backup PCBA Calibration EEPROM Response - USAGE"="", "NG UNIT - Disconnect UUT"=""}, "SKU"="", "Plate_Diameter"="", "Alarm"=""} ("Data in"), "SN"=w122, "Table"=w121, "Station ID"=w120, "Count"=w115, "daemon reference"=w114, "Config"=w110) -> (w123:T3)
            n42 = Select(t="Check_Carrier_Sensor_Signal", s=w118, f=w119) -> ()  [unwired: 1 out]
          }
          frame True {
          }
        }
        n43 = call "LogStatus.vi"("error in (no error)"=w105, "last message"=w96, "message"=w92) -> ("error  out"=w104:errorcluster)  [unwired: 8 in]
      }
      frame "MES_Verification" {
        (unwired) "Check_UUT_Sensor_Signal"
        n44 = Unbundle By Name(w219) -> ("Recipe"=w173:refnum<vi>, "MES"=w194:refnum<vi>, "ProductID"=w215:refnum<vi>)
        n45 = Unbundle By Name(w212) -> ("Enable_User"=w211:bool, "FFTesterPath"=w210:path)
        n46 = Unbundle By Name(w208) -> ("SN"=w220:string)
        n47 = call "User.vi"("Step"=enum16{"Initial", "Write", "Read"}."Read") -> ("User out"=w213:string)  [unwired: 9 in, 1 out]
        n48 = call "Get Unit Info.vi"("路径"=w210, "Enable_User"=w211, "UserID"=w213, "Serial Number"=w220) -> ("strUnitInfo"=w186:string, "Operation Success"=w216:bool, "结果字符串"=w200:string)  [unwired: 2 in, 3 out]
        n49 = Concatenate Strings(w200, "\r\n", w186) -> (w193:string)
        n50 = xnode "匹配正则表达式"("输入字符串"=w186, "正则表达式"="TestTimes_X692</Name><Value>") -> ("匹配之后"=w198:string)  [unwired: 4 in, 4 out]
        n51 = xnode "匹配正则表达式"("输入字符串"=w186, "正则表达式"="PlateSizeSKUforUIProvision</Name><Value>") -> ("匹配之后"=w189:string)  [unwired: 4 in, 4 out]
        n52 = xnode "匹配正则表达式"("输入字符串"=w186, "正则表达式"="PlateSizeforUIProvision</Name><Value>") -> ("匹配之后"=w190:string)  [unwired: 4 in, 4 out]
        n53 = xnode "匹配正则表达式"("输入字符串"=w186, "正则表达式"="<Name>DDMMotorSN_X692</Name><Value>") -> ("匹配之后"=w204:string)  [unwired: 4 in, 4 out]
        n54 = xnode "匹配正则表达式"("输入字符串"=w198, "正则表达式"="</Value>") -> ("匹配之前"=w195:string)  [unwired: 4 in, 4 out]
        n55 = xnode "匹配正则表达式"("输入字符串"=w190, "正则表达式"="</Value>") -> ("匹配之前"=w162:string)  [unwired: 4 in, 4 out]
        n56 = xnode "匹配正则表达式"("输入字符串"=w189, "正则表达式"="</Value>") -> ("匹配之前"=w171:string)  [unwired: 4 in, 4 out]
        n57 = xnode "匹配正则表达式"("输入字符串"=w204, "正则表达式"="</Value>") -> ("匹配之前"=w203:string)  [unwired: 4 in, 4 out]
        n58 = Empty String/Path?(string/path=w162) -> (empty?=w185:bool)
        n59 = Empty String/Path?(string/path=w171) -> (empty?=w184:bool)
        n60 = Concatenate Strings("'", w203) -> (w202:string)
        n61 = call "Read_Sku.vi"("SKU"=w171) -> ("Recipe"=w170:string)  [unwired: 10 in]
        n62 = Empty String/Path?(string/path=w170) -> (empty?=w169:bool)
        n63 = property class="CmbBox"(reference=w173, "Value"=w170) -> ()  [unwired: 1 in, 2 out]
        n64 = call "1-BasePath.vi"("Step"=enum16{"Initial", "Write", "Read"}."Read") -> ("Path Out"=w179:path)  [unwired: 9 in, 1 out]
        n65 = call "ReadConfigandSetting.vi"("Recipe"=w170, "Path Out"=w179) -> ("错误输出"=w168:errorcluster, "ConfigData"=w163:string[][], "TableData"=w182:string[][])  [unwired: 7 in]
        n66 = Build Path(base path=w179, name or relative path="data\\Recipe.ini") -> (appended path=w178:path)
        n67 = case shown="真" FALSE {
          tunnel: w178 -> [_ w226]
          tunnel: w170 -> [_ w224]
          frame False {
          }
          frame True {
            w225 = cluster{"Recipe":string} {"Recipe"=""}  # Recipe
            n68 = Bundle By Name(cluster=w225, "Recipe"=w224) -> (w227:cluster{"Recipe":string})
            n69 = call-poly "Read&WriteFile.vi"("Variant"=w227, "path"=w226) -> ()  [unwired: 9 in, 1 out]
          }
        }
        n70 = Delete From Array(array=w182, length=1 ("长度"), index (row)=0 ("索引 (行)")) -> (deleted portion=w180:string[][], array with subset deleted=w181:string[][])  [unwired: 1 in]
        n71 = call "Select_UUT_Table.vi"("all Title"=w180, "all Table"=w181) -> ("Table"=w172:string[][])  [unwired: 8 in, 1 out]
        n72 = Search and Replace String(input string=w162, search string="mm" ("替换字符串(\"\")")) -> (result string=w166:string)  [unwired: 6 in, 3 out]
        n73 = call "Index_Config.vi"("Action"="MAX_POWER_MODE_Orifice_size", "config"=w163) -> ("data"=w165:string)  [unwired: 9 in]
        n74 = Bundle By Name(cluster=w208, "MES DDM SN"=w202, "Retest"=w195, "Plate_Diameter"=w162, "SKU"=w171, "Table"=w172, "Config"=w163) -> (w207:T3)
        n75 = Not Equal?(x=w165, y=w166) -> (x != y?=w161:bool)
        n76 = Compound Arithmetic op=OR ("复合运算")(w161, w168, w169, w185, w184) -> (w183:bool)
        n77 = case shown="真" w216 {
          tunnel: w215 -> [w1145 w1146]
          tunnel: ["Wait_Scan_ProductID" ("Value") w1150] -> _
          tunnel: w194 -> [w1142 w1149]
          tunnel: w193 -> [w1141 w1148]
          tunnel: w183 -> [_ w1147]
          frame False {
            (unwired) TRUE ("闪烁")
            n78 = property class="Str"(reference=w1145, "Value"="" ("值")) -> ()  [unwired: 1 in, 2 out]
            n79 = property class="Str"(reference=w1142, "Value"=w1141, "Blinking"=FALSE ("闪烁")) -> ()  [unwired: 1 in, 2 out]
          }
          frame True {
            n80 = case shown="假" w1147 {
              tunnel: ["Check_UUT_Sensor_Signal" "Wait_Scan_ProductID" ("Value")] -> w1150
              tunnel: w1149 -> [w1153 w1155]
              tunnel: w1148 -> [w1152 _]
              tunnel: w1146 -> [_ w1158]
              frame False {
                n81 = property class="Str"(reference=w1153, "Value"=w1152) -> ()  [unwired: 1 in, 2 out]
              }
              frame True {
                n82 = property class="Str"(reference=w1158, "Value"="" ("值")) -> ()  [unwired: 1 in, 2 out]
                n83 = property class="Str"(reference=w1155, "Value"="0; SKU or PlateSize Data Error" ("字符串"), "Blinking"=FALSE ("闪烁")) -> ()  [unwired: 1 in, 2 out]
              }
            }
          }
        }
        n84 = call "LogStatus.vi"("error in (no error)"=w222, "last message"=w218, "message"=w217) -> ("error  out"=w221:errorcluster)  [unwired: 8 in]
      }
      frame "Check_UUT_Sensor_Signal" {
        n85 = call "IO.vi"("IO Name"=string[] ["Presence Detection Sensor"], "IO?"=enum16{"DI", "DO"}."DI") -> ("DI"=w1163:bool[])  [unwired: 8 in, 1 out]
        n86 = And Array Elements(Boolean array=w1163) -> (logical AND=w1162:bool)
        n87 = Select(t="Wait_Start_signal", s=w1162, f="Check_UUT_Sensor_Signal") -> (s? t:f=w1167:string)
        n88 = call "LogStatus.vi"("error in (no error)"=w1172, "last message"=w1164, "message"=w1165) -> ("error  out"=w1171:errorcluster)  [unwired: 8 in]
      }
      frame "Wait_Start_signal" {
        n89 = Unbundle By Name(w1176) -> ("Station ID"=w1177:string)
        n90 = Unbundle By Name(w1180) -> ("Device state"=w1179:refnum<vi>)
        n91 = call "IO.vi"("IO Name"=string[] ["Start_L", "Start_R"], "IO?"=enum16{"DI", "DO"}."DI") -> ("DI"=w1182:bool[])  [unwired: 8 in, 1 out]
        n92 = And Array Elements(Boolean array=w1182) -> (logical AND=w1181:bool)
        n93 = case shown="真" w1181 {
          tunnel: w1179 -> [_ w1197]
          tunnel: w1176 -> [w1191 w1196]
          tunnel: [w1191 w1195] -> w1174
          tunnel: ["Wait_Start_signal" w1193] -> w1178
          tunnel: w1177 -> [_ w1192]
          frame False {
          }
          frame True {
            n94 = call "Cheak File.vi"("Station ID"=w1192) -> ("true"=w1194:bool)  [unwired: 10 in]
            n95 = case shown="假" w1194 {
              tunnel: w1197 -> [w1204 _]
              tunnel: w1196 -> [w1203 w1207]
              tunnel: [w1201 w1207] -> w1195
              tunnel: ["5.3.1 Power-up Test" ("Name") "Wait_Start_signal"] -> w1193
              frame False {
                n96 = Get Date/Time In Seconds() -> (seconds since 1Jan1904=w1202:timestamp)
                n97 = Bundle By Name(cluster=w1203, "Start Time"=w1202) -> (w1201:T3)
                n98 = call "Start.vi"("Start In"=TRUE, "Step"=enum16{"Initial", "Write", "Read"}."Write") -> ()  [unwired: 8 in, 2 out]
                n99 = call "StatusLamp.vi"("State"="Testing", "Boolean输入"=w1204) -> ()  [unwired: 9 in, 1 out]
              }
              frame True {
              }
            }
          }
        }
        n100 = call "LogStatus.vi"("error in (no error)"=w1188, "last message"=w1183, "message"=w1184) -> ("error  out"=w1187:errorcluster)  [unwired: 8 in]
      }
      frame "5.3.1 Power-up Test" {
        n101 = call "LogStatus.vi"("error in (no error)"=w1222, "last message"=w1221, "message"=w1216) -> ("error  out"=w1214:errorcluster)  [unwired: 8 in]
        n102 = call "1.0.0_Power-up Test.vi"("Data in"=w1209, "error in (no error)"=w1214, "AllControls In"=w1211, 10:w1215, "Message Queue out"=w1220) -> ("error out"=w1218:errorcluster, "Flow"=w1208:string, "Data"=w1217:T4, "Message Queue Out"=w1219:T5, "Data out"=w1210:T3)  [unwired: 2 in]
        n103 = Equal?(x="Error", y=w1208) -> (x = y?=w1212:bool)
        n104 = case shown="真" w1212 {
          frame False {
          }
          frame True {
            n105 = call "6-AlarmStatus.vi"("AlarmValue"=TRUE, "AlarmIndex"=AlarmIndex."Test Error", "Step"=enum16{"Initial", "Write", "Read"}."Write") -> ()  [unwired: 7 in, 2 out]
          }
        }
      }
      frame "5.3.2 Firware Version Check" {
        n106 = call "LogStatus.vi"("error in (no error)"=w1241, "last message"=w1240, "message"=w1235) -> ("error  out"=w1233:errorcluster)  [unwired: 8 in]
        n107 = call "2.0.0_Firware Version Check.vi"(".batCM"=w1226, "Data in"=w1228, "error in (no error)"=w1233, "AllControls In"=w1230, 10:w1234, "Message Queue out"=w1239) -> ("error out"=w1237:errorcluster, "Flow"=w1227:string, "Data"=w1236:T4, "Message Queue Out"=w1238:T5, "Data out"=w1229:T3)  [unwired: 1 in]
        n108 = Equal?(x="Error", y=w1227) -> (x = y?=w1231:bool)
        n109 = case shown="真" w1231 {
          frame False {
          }
          frame True {
            n110 = call "6-AlarmStatus.vi"("AlarmValue"=TRUE, "AlarmIndex"=AlarmIndex."Test Error", "Step"=enum16{"Initial", "Write", "Read"}."Write") -> ()  [unwired: 7 in, 2 out]
          }
        }
      }
      frame "5.3.3 LED Test" {
        n111 = call "LogStatus.vi"("error in (no error)"=w1260, "last message"=w1259, "message"=w1254) -> ("error  out"=w1252:errorcluster)  [unwired: 8 in]
        n112 = call "3.0.0_LED Test.vi"(".batCMD"=w1245, "Data in"=w1247, "error in (no error)"=w1252, "AllControls In"=w1249, 10:w1253, "Message Queue out"=w1258) -> ("error out"=w1256:errorcluster, "Flow"=w1246:string, "Data"=w1255:T4, "Message Queue Out"=w1257:T5, "Data out"=w1248:T3)  [unwired: 1 in]
        n113 = Equal?(x="Error", y=w1246) -> (x = y?=w1250:bool)
        n114 = case shown="真" w1250 {
          frame False {
          }
          frame True {
            n115 = call "6-AlarmStatus.vi"("AlarmValue"=TRUE, "AlarmIndex"=AlarmIndex."Test Error", "Step"=enum16{"Initial", "Write", "Read"}."Write") -> ()  [unwired: 7 in, 2 out]
          }
        }
      }
      frame "5.3.5 Brush Motor Test" {
        n116 = call "LogStatus.vi"("error in (no error)"=w1279, "last message"=w1278, "message"=w1273) -> ("error  out"=w1271:errorcluster)  [unwired: 8 in]
        n117 = call "5.0.0_Brush Motor Test.vi"(".batCMD"=w1264, "Data in"=w1266, "error in (no error)"=w1271, "AllControls In"=w1268, 10:w1272, "Message Queue out"=w1277) -> ("error out"=w1275:errorcluster, "Flow"=w1265:string, "Data"=w1274:T4, "Message Queue Out"=w1276:T5, "Data out"=w1267:T3)  [unwired: 1 in]
        n118 = Equal?(x="Error", y=w1265) -> (x = y?=w1269:bool)
        n119 = case shown="真" w1269 {
          frame False {
          }
          frame True {
            n120 = call "6-AlarmStatus.vi"("AlarmValue"=TRUE, "AlarmIndex"=AlarmIndex."Test Error", "Step"=enum16{"Initial", "Write", "Read"}."Write") -> ()  [unwired: 7 in, 2 out]
          }
        }
      }
      frame "5.3.6 Pump Motor Test" {
        n121 = call "LogStatus.vi"("error in (no error)"=w1298, "last message"=w1297, "message"=w1292) -> ("error  out"=w1290:errorcluster)  [unwired: 8 in]
        n122 = call "6.0.0_Pump Motor Test.vi"(".batCMD"=w1283, "Data in"=w1285, "error in (no error)"=w1290, "AllControls In"=w1287, 10:w1291, "Message Queue out"=w1296) -> ("error out"=w1294:errorcluster, "Flow"=w1284:string, "Data"=w1293:T4, "Message Queue Out"=w1295:T5, "Data out"=w1286:T3)  [unwired: 1 in]
        n123 = Equal?(x="Error", y=w1284) -> (x = y?=w1288:bool)
        n124 = case shown="真" w1288 {
          frame False {
          }
          frame True {
            n125 = call "6-AlarmStatus.vi"("AlarmValue"=TRUE, "AlarmIndex"=AlarmIndex."Test Error", "Step"=enum16{"Initial", "Write", "Read"}."Write") -> ()  [unwired: 7 in, 2 out]
          }
        }
      }
      frame "Disconnect_UUT" {
        (unwired) "Off_Power_Supply_Output" ("Name")
        n126 = Unbundle By Name(w1317) -> ("OK/NG"=w1316:bool, "daemon reference"=w1320:refnum<k5>)
        n127 = call "HD_Config.vi"("Step"=enum16{"Initial", "Write", "Read"}."Read") -> ("HD Config out"=w1312:T12)  [unwired: 9 in, 1 out]
        n128 = Unbundle By Name(w1312) -> ("Tempt&Hum.COM"=w1310:refnum<visa-resource-name>)
        n129 = call "disconnect.vi"("daemon reference in"=w1320) -> ("error out"=w1315:errorcluster, "response"=w1314:string, "daemon reference out"=w1321:refnum<k5>)  [unwired: 7 in, 1 out]
        n130 = call <instrlib>:"example.vi"("Current Level (A)"=0.0, "Voltage Level (V)"=0.0, "VISA resource name"=w1310, "FLAG"=TRUE) -> ("error out"=w1303:errorcluster)  [unwired: 4 in, 3 out]
        n131 = call <vilib>:"Clear Errors.vi"("error in (no error)"=w1315) -> ()  [unwired: 5 in, 2 out]
        n132 = call "时间延迟"("error in (no error)"=w1303) -> ("error out"=w1302:errorcluster)  [unwired: 10 in]
        n133 = case shown="真" w1316 {
          tunnel: w1321 -> [w1328 w1334]
          tunnel: w1317 -> [w1329 w1333]
          tunnel: [w1330 w1332] -> w1319
          tunnel: w1314 -> [w1327 w1331]
          frame False {
            n134 = Bundle By Name(cluster=w1329, "daemon reference"=w1328, "NG.NG UNIT - Disconnect UUT"=w1327) -> (w1330:T3)
          }
          frame True {
            n135 = Bundle By Name(cluster=w1333, "daemon reference"=w1334, "GOOD.GOOD UNIT - Disconnect UUT"=w1331) -> (w1332:T3)
          }
        }
        n136 = call "LogStatus.vi"("error in (no error)"=w1325, "last message"=w1322, "message"=w1323) -> ("error  out"=w1324:errorcluster)  [unwired: 8 in]
        n137 = call "IO.vi"("错误常量"=w1302, "DO DATA"=bool[] [FALSE, FALSE, FALSE, FALSE, FALSE, FALSE, FALSE, FALSE], "IO Name"=string[] ["psu+   J3_1", "psu-   J3_5", "UART1_3V3  J63_1", "UART1_TX   J63_5", "UART1_RX   J63_6", "UART1_GND  J63_10", "PSU S+ J3_1", "PSU S- J3_5"], "IO?"=enum16{"DI", "DO"}."DO") -> ()  [unwired: 6 in, 2 out]
      }
      frame "UI_Display_and_Save_Test_Data" {
        n138 = Unbundle By Name(w1369) -> ("ProductID"=w1355:refnum<vi>, "MES bool"=w1357:refnum<vi>, "Device state"=w1361:refnum<vi>, "TestInfo"=w1366:refnum<vi>, "Current CT"=w1368:refnum<vi>)
        n139 = Unbundle By Name(w1341) -> ("Start Time"=w1371:timestamp, "Count"=w1370:T7, "OK/NG"=w1352:bool)
        n140 = Get Date/Time In Seconds() -> (seconds since 1Jan1904=w1376:timestamp)
        n141 = Subtract(x=w1376, y=w1371) -> (x-y=w1362:dbl)
        n142 = property class="Str"(reference=w1355, "Value"="" ("值")) -> ()  [unwired: 1 in, 2 out]
        n143 = property class="DigNum (严格)"(reference=w1368, "Value"=w1362) -> ()  [unwired: 1 in, 2 out]
        n144 = Unbundle By Name(w1370) -> ("Total"=w1375:i32, "OK"=w1349:i32, "NG"=w1350:i32)
        n145 = Increment(x=w1375) -> (x+1=w1373:i32)
        n146 = Increment(x=w1349) -> (x+1=w1353:i32)
        n147 = Increment(x=w1350) -> (x+1=w1351:i32)
        n148 = Select(t=w1353, s=w1352, f=w1349) -> (s? t:f=w1348:i32)
        n149 = Select(t=w1350, s=w1352, f=w1351) -> (s? t:f=w1347:i32)
        n150 = Divide(x=w1348, y=w1373) -> (x/y=w1374:dbl)
        n151 = Select(t="Pass" ("State"), s=w1352, f="Fail" ("State")) -> (s? t:f=w1360:string)
        n152 = Multiply(x=w1374, y=100.0) -> (x*y=w1346:dbl)
        n153 = Bundle By Name(cluster=w1370, "Total"=w1373, "OK"=w1348, "NG"=w1347, "Yield"=w1346) -> (w1365:T7)
        n154 = call "StatusLamp.vi"("State"=w1360, "Boolean输入"=w1361) -> ()  [unwired: 9 in, 1 out]
        n155 = property class="Clust (严格)"(reference=w1366, "Value"=w1365) -> ()  [unwired: 1 in, 2 out]
        n156 = Bundle By Name(cluster=w1341, "CT"=w1362, "Count"=w1365) -> (w1342:T3)
        n157 = Flatten To XML(anything=w1342) -> (xml string=w1367:string)
        n158 = call "HD_Config.vi"("Step"=enum16{"Initial", "Write", "Read"}."Read") -> ("HD Config out"=w1339:T12)  [unwired: 9 in, 1 out]
        n159 = call "AMC Send Local Message.vi"("Message Value"=w1367, "Message Name"="Save", "Message Queue in"=w1382) -> ()  [unwired: 7 in, 2 out]
        n160 = property class="Bool (严格)"(reference=w1357) -> ("Value"=w1356:bool)  [unwired: 1 in, 2 out]
        n161 = Unbundle By Name(w1339) -> ("GRR"=w1338:bool)
        n162 = call "Start.vi"("Start In"=FALSE, "Step"=enum16{"Initial", "Write", "Read"}."Write") -> ()  [unwired: 8 in, 2 out]
        n163 = Select(t="Upload_MES_System", s=w1356, f="Wait_Scan_ProductID" ("Name")) -> (s? t:f=w1336:string)
        n164 = call "LogStatus.vi"("error in (no error)"=w1380, "last message"=w1377, "message"=w1378) -> ("error  out"=w1379:errorcluster)  [unwired: 8 in]
        n165 = Select(t="Wait_Scan_ProductID" ("Name"), s=w1338, f=w1336) -> (s? t:f=w1335:string)
      }
      frame "Upload_MES_System" {
        n166 = Unbundle By Name(w1386) -> ("MES"=w1385:bool)
        n167 = call "Csv_fill_null.vi"("Data in"=w1388) -> ("Data out"=w1387:T3)  [unwired: 10 in]
        n168 = Unbundle By Name(w1388) -> ("SN"=w1392:string, "OK/NG"=w1400:bool)
        n169 = Format Date/Time String(time format string (%c)="%H%M%S" ("时间格式字符串(%c)")) -> (date/time string=w1393:string)  [unwired: 2 in]
        n170 = call "PathChoose.vi"(11:PathChoose."TestData") -> ("Path_Out"=w1396:path)  [unwired: 10 in]
        n171 = Concatenate Strings(w1392, "_" ("字符串"), w1393, ".csv" ("字符串")) -> (w1390:string)
        n172 = call "Data_Table.vi"("AllControls In"=w1384, "Data in"=w1387) -> ("Data out"=w1399:string[][])  [unwired: 9 in]
        n173 = Build Path(base path=w1396, name or relative path=w1390) -> (appended path=w1395:path)
        n174 = case shown="假" w1385 {
          tunnel: w1384 -> [w1415 _]
          tunnel: w1400 -> [w1411 _]
          tunnel: w1399 -> [w1410 _]
          tunnel: w1392 -> [w1409 _]
          frame False {
            n175 = call "Save Result.vi"("Data"=w1410, "布尔"=w1411, "ProductID"=w1409) -> ("结果字符串"=w1413:string)  [unwired: 5 in, 3 out]
            n176 = Unbundle By Name(w1415) -> ("MES"=w1414:refnum<vi>)
            n177 = Not Equal?(x=w1413, y="0") -> (x != y?=w1412:bool)
            n178 = property class="Str"(reference=w1414, "Value"=w1413, "Blinking"=w1412) -> ()  [unwired: 1 in, 2 out]
          }
          frame True {
          }
        }
        n179 = call-poly <vilib>:"Write Delimited Spreadsheet.vi"("file path (dialog if empty)"=w1395, "2D data"=w1399, "delimiter (\\t)"="," ("delimiter (\\t)")) -> ()  [unwired: 11 in, 2 out]
        n180 = call "LogStatus.vi"("error in (no error)"=w1406, "last message"=w1403, "message"=w1402) -> ("error  out"=w1405:errorcluster)  [unwired: 8 in]
      }
      frame "Error" {
        n181 = Unbundle By Name(w1416) -> ("daemon reference"=w1425:refnum<k5>)
        n182 = Unbundle By Name(w1432) -> ("Device state"=w1418:refnum<vi>, "ProductID"=w1431:refnum<vi>)
        n183 = property class="Str"(reference=w1431) -> ("Value"=w1430:string)  [unwired: 1 in, 2 out]
        n184 = Not A Number/Path/Refnum?(number/path/refnum=w1425) -> (NaN/Path/Refnum?=w1424:bool)
        n185 = Empty String/Path?(string/path=w1430) -> (empty?=w1429:bool)
        n186 = Select(t="Off_Power_Supply_Output", s=w1424, f="Disconnect_UUT") -> (s? t:f=w1422:string)
        n187 = call "6-AlarmStatus.vi"("Step"=enum16{"Initial", "Write", "Read"}."Read") -> ("AlarmValue Out"=w1427:bool[])  [unwired: 9 in, 1 out]
        n188 = call "IO.vi"("IO Name"=string[] ["Reset"], "IO?"=enum16{"DI", "DO"}."DI") -> ("DI"=w1438:bool[])  [unwired: 8 in, 1 out]
        n189 = Or Array Elements(Boolean array=w1427) -> (logical OR=w1420:bool)
        n190 = And Array Elements(Boolean array=w1438) -> (logical AND=w1419:bool)
        n191 = Not(x=w1420) -> (.not. x?=w1417:bool)
        n192 = Select(t="Initialize_UI" ("Name"), s=w1429, f=w1422) -> (s? t:f=w1435:string)
        n193 = And(x=w1417, y=w1419) -> ()  [unwired: 1 out]
        n194 = Select(t=w1435, s=w1417, f="Error" ("Name")) -> (s? t:f=w1433:string)
        n195 = case shown="真" w1417 {
          tunnel: w1418 -> [_ w1445]
          frame False {
          }
          frame True {
            n196 = call "StatusLamp.vi"("State"="Testing", "Boolean输入"=w1445) -> ()  [unwired: 9 in, 1 out]
          }
        }
        n197 = call "LogStatus.vi"("error in (no error)"=w1443, "last message"=w1440, "message"=w1441) -> ("error  out"=w1442:errorcluster)  [unwired: 8 in]
      }
      frame "Stop_E-Stop" {
        n198 = while {
          shift-right: [w1481] -> w1452
          shift-left: w1450 -> [w1480]
          tunnel: w1451 -> [w1481]
          tunnel: [w1480] -> w1453
          stop <- FALSE continue-if-true
          n199 = Wait (ms)(milliseconds to wait=u32 1 ("等待时间（毫秒）")) -> ()  [unwired: 1 out]
        }
        n200 = Unbundle By Name(w1463) -> ("Device state"=w1457:refnum<vi>, "ProductID"=w1467:refnum<vi>)
        n201 = property class="Str"(reference=w1467) -> ("Value"=w1466:string)  [unwired: 1 in, 2 out]
        n202 = Not Equal?(x=w1452, y=w1453) -> (x != y?=w1449:bool)
        n203 = Empty String/Path?(string/path=w1466) -> (empty?=w1465:bool)
        n204 = call "6-AlarmStatus.vi"("Step"=enum16{"Initial", "Write", "Read"}."Read") -> ("AlarmValue Out"=w1454:bool[])  [unwired: 9 in, 1 out]
        n205 = case shown="真" w1449 {
          tunnel: w1456 -> [w1482 w1503]
          tunnel: [w1482 w1502] -> w1455
          tunnel: w1454 -> [_ w1487]
          frame False {
          }
          frame True {
            w1483 = 1 ("长度")
            n206 = call "3-AlarmConfig.vi"("Step"=enum16{"Initial", "Write", "Read"}."Read") -> ("AlarmConfig Out"=w1500:string[][])  [unwired: 9 in, 1 out]
            n207 = Index Array ("索引数组")(array=w1500, index (col)=1 ("索引 (列)")) -> (element=w1485:string[])  [unwired: 1 in]
            n208 = Search 1D Array(1D array=w1485, element="Test Error" ("元素")) -> (index of element=w1484:i32)  [unwired: 1 in]
            n209 = Delete From Array(array=w1485, length=w1483, index=w1484) -> (array with subset deleted=w1489:string[])  [unwired: 1 out]
            n210 = Delete From Array(array=w1487, length=w1483, index=w1484) -> (array with subset deleted=w1488:bool[])  [unwired: 1 out]
            n211 = for {
              tunnel: w1489 -> [w1505] mode=indexing
              tunnel: w1488 -> [w1504] mode=indexing
              tunnel: [w1505] -> w1495
              stop <- w1504 stop-if-true
            }
            n212 = call <vilib>:"Space Constant.vi"() -> ("String"=w1496:string)
            n213 = Search and Replace String(replace all?=TRUE ("replace all? (F)"), input string=w1495, search string=";", replace string=w1496) -> (result string=w1491:string)  [unwired: 4 in, 3 out]
            n214 = call <vilib>:"Space Constant.vi"() -> ("String"=w1494:string)
            n215 = Search and Replace String(replace all?=TRUE ("replace all? (F)"), input string=w1491, search string="-", replace string=w1494) -> (result string=w1490:string)  [unwired: 4 in, 3 out]
            n216 = Bundle By Name(cluster=w1503, "Alarm"=w1490) -> (w1502:T3)
          }
        }
        n217 = call "IO.vi"("IO Name"=string[] ["Reset"], "IO?"=enum16{"DI", "DO"}."DI") -> ("DI"=w1471:bool[])  [unwired: 8 in, 1 out]
        n218 = Or Array Elements(Boolean array=w1454) -> (logical OR=w1459:bool)
        n219 = And Array Elements(Boolean array=w1471) -> (logical AND=w1458:bool)
        n220 = Not(x=w1459) -> (.not. x?=w1448:bool)
        n221 = Select(t="Initialize_UI" ("Name"), s=w1465, f="Disconnect_UUT") -> (s? t:f=w1468:string)
        n222 = And(x=w1448, y=w1458) -> ()  [unwired: 1 out]
        n223 = Select(t=w1468, s=w1448, f="Stop_E-Stop" ("Name")) -> (s? t:f=w1462:string)
        n224 = case shown="真" w1448 {
          tunnel: w1457 -> [_ w1477]
          frame False {
          }
          frame True {
            n225 = call "StatusLamp.vi"("State"="Testing", "Boolean输入"=w1477) -> ()  [unwired: 9 in, 1 out]
          }
        }
        n226 = call "LogStatus.vi"("error in (no error)"=w1474, "last message"=w1450, "message"=w1451) -> ("error  out"=w1473:errorcluster)  [unwired: 8 in]
      }
      frame "Exit_AutoRun" {
        n227 = call "HD_Config.vi"("Step"=enum16{"Initial", "Write", "Read"}."Read") -> ("HD Config out"=w1516:T12)  [unwired: 9 in, 1 out]
        n228 = Unbundle By Name(w1516) -> ("Tempt&Hum.COM"=w1514:refnum<visa-resource-name>)
        n229 = call <instrlib>:"example.vi"("Current Level (A)"=0.0, "Voltage Level (V)"=0.0, "VISA resource name"=w1514, "FLAG"=TRUE) -> ("error out"=w1507:errorcluster)  [unwired: 4 in, 3 out]
        n230 = call "LogStatus.vi"("error in (no error)"=w1518, "message"=w1521) -> ("error  out"=w1520:errorcluster)  [unwired: 9 in]
        n231 = call "时间延迟2"("error in (no error)"=w1507) -> ("error out"=w1506:errorcluster)  [unwired: 10 in]
        n232 = call "IO.vi"("错误常量"=w1506, "DO DATA"=bool[] [FALSE, FALSE, FALSE, FALSE, FALSE, FALSE, FALSE, FALSE], "IO Name"=string[] ["psu+   J3_1", "psu-   J3_5", "UART1_3V3  J63_1", "UART1_TX   J63_5", "UART1_RX   J63_6", "UART1_GND  J63_10", "PSU S+ J3_1", "PSU S- J3_5"], "IO?"=enum16{"DI", "DO"}."DO") -> ()  [unwired: 6 in, 2 out]
      }
    }
    n233 = call "AMC Run Step.vi"("Message Queue In"=w35, "Message Name"=w30, "Message Value"=w29, "error in (no error)"=w31, "Mli/Sig"=FALSE) -> ("Message Queue Out"=w40:T5, "error out"=w41:errorcluster)  [unwired: 13 in]
  }
  n234 = while {
    tunnel: w14 -> [w1530]
    tunnel: "AllControls In" -> [w1525]
    tunnel: [w1524] -> w4
    stop <- w1531 stop-if-true
    n235 = call "AMC Read Next Message.vi"("timeout (1ms)"=100, "Message Queue in"=w1530) -> ("Message Value"=w1526:string, "Message Name"=w1529:string, "Message Queue out"=w1524:T5)  [unwired: 2 in, 5 out]
    n236 = Wait (ms)(milliseconds to wait=u32 1) -> ()  [unwired: 1 out]
    n237 = case shown="\"Save\"" w1529 {
      tunnel: w1526 -> [_ _ w1540]
      tunnel: w1525 -> [_ _ w1539]
      frame "Null", Default {
      }
      frame "Wait" {
      }
      frame "Save" {
        n238 = Unflatten From XML(xml string=w1540, type=T3 {"Initialisation"={"LMT - Connect UUT (con COM)"="", "LMT - Software Version (rrel)"="", "LMT - Write SKU file (wskuc)"="", "LMT - SKU file name"="", "Connect UUT DDM"="", "Read DDM EOL Timestamp - Mode"="", "Read DDM EOL Timestamp - Timestamp"="", "Read DDM EOL Timestamp - Rig ID"="", "Read DDM EOL Timestamp - Passmark ID"="", "Read DDM EOL Timestamp - Passmark Rev"="", "Software Version before flashing"="", "Read Hardware Serial"="", "UUT DDM SN"="", "Compare DDM SN with MES SN"="", "Backup PCBA Calibration EEPROM Response - CAL"="", "Flash Firmware Version"="", "Check SW Version"="", "Read DDM SW Version after flashing"="", "Set SKU Config"="", "Ready Status"="", "Set Device Mode to EOL"="", "DDM Parameter - Voltage"="", "DDM Parameter - Current"="", "DDM Parameter - Power"="", "DDM Parameter - Speed"="", "DDM Parameter - Pressure"="", "Tester Parameter - Voltage"="", "Tester Parameter - Current"="", "Tester Parameter - Power"="", "Tester Parameter - Ambient Pressure"="", "Tester Parameter - Ambient Temperature"="", "Calculated Parameter - DDM Pressure Corrected"="", "Calculated Parameter - DDM Real Power"="", "Calculated Parameter - Delta V"=""}, "BEMF_Calibration"={"Calibration Result - eol_cold_bemf_temp"="", "DDM Ambient Temp"="", "Restriction Plate Diameter"="", "Calibration Result - eol_bemf_mp_cold_coef_a"="", "Calibration Result - eol_bemf_mp_cold_coef_b"="", "Calibration Result - eol_bemf_mp_cold_coef_c"="", "Calibration Result - eol_bemf_lsi_cold_ref_coeffs"="", "Get - Calibration Result - eol_bemf_lsi_speed"="", "Get - Calibration Result - eol_bemf_lsi_integral_0"="", "Calibration Result - eol_bemf_lsi_integral_1"="", "Get - Calibration Result - eol_bemf_lsi_integral_2"="", "Get - Calibration Result - eol_cold_bemf"="", "Get - Calibration Result - eol_cold_bemf_fisf"="", "Finalise Calibration"="", "Compare -Calibration Result - eol_cold_bemf"="", "Compare -Calibration Result - eol_cold_bemf_fisf"=""}, "ECO"={"Reset Power Tune"="", "Reset BEMF FISF Calibration"="", "Restriction Plate Diameter"="", "ECO - Stabilisation Time"="", "ECO - DDM Parameter - Voltage"="", "ECO - DDM Parameter - Current"="", "ECO - DDM Parameter - Power"="", "ECO - DDM Parameter - Measured Power"="", "ECO - DDM Parameter - Speed"="", "ECO - DDM Parameter - Pressure"="", "ECO - Tester Parameter - Voltage"="", "ECO - Tester Parameter - Current"="", "ECO - Tester Parameter - Power"="", "ECO - Tester Parameter - Ambient Pressure"="", "ECO - Tester Parameter - Ambient Temperature"="", "ECO - Tester Parameter - Ambient Humidity"="", "ECO - Calculated Parameter - DDM Pressure Corrected"="", "ECO - Calculated Parameter - DDM Real Power"="", "ECO - Calculated Parameter - Delta V"="", "ECO - Calculated Parameter - Flowrate"="", "ECO - Calculated Parameter - Airwatt"="", "ECO - Formula"="", "PT ECO - Power Tune Mode Status"=""}, "BOOST"={"Restriction Plate Diameter"="", "BOOST - Stabilisation Time"="", "BOOST - DDM Parameter - Voltage"="", "BOOST - DDM Parameter - Current"="", "BOOST - DDM Parameter - Power"="", "BOOST - DDM Parameter - Measured Power"="", "BOOST - DDM Parameter - Speed"="", "BOOST - DDM Parameter - Pressure"="", "BOOST - Tester Parameter - Voltage"="", "BOOST - Tester Parameter - Current"="", "BOOST - Tester Parameter - Power"="", "BOOST - Tester Parameter - Ambient Pressure"="", "BOOST - Tester Parameter - Ambient Temperature"="", "BOOST - Tester Parameter - Ambient Humidity"="", "BOOST - Calculated Parameter - DDM Pressure Corrected"="", "BOOST - Calculated Parameter - DDM Real Power"="", "BOOST - Calculated Parameter - Delta V"="", "BOOST - Calculated Parameter - Flowrate"="", "BOOST - Calculated Parameter - Airwatt"="", "BOOST - Get AM Presence"="", "Air Muscle Turn Off Status"="", "BOOST - Air Muscle Calculated Parameter - Airwatt B"="", "BOOST - Air Muscle Calculate Airwatt Delta"="", "PT BOOST - Power Tune Mode Status"="", "Finalise Calibration"="", "ECO - Get AW Calibration value"="", "BOOST - Get AW Calibration value"=""}, "MAX"={"Restriction Plate Diameter"="", "MAX - Stabilisation Time"="", "Get Average Delta Tmag (LSIdelta_FISFdelta_LSItmag_FISFtmag_IIRtmag)"="", "Get Average Delta Tmag FISF"="", "MAX - DDM Parameter - Voltage"="", "MAX - DDM Parameter - Current"="", "MAX - DDM Parameter - Power"="", "MAX - DDM Parameter - Measured Power"="", "MAX - DDM Parameter - Speed"="", "MAX - DDM Parameter - Pressure"="", "MAX - Tester Parameter - Voltage"="", "MAX - Tester Parameter - Current"="", "MAX - Tester Parameter - Power"="", "MAX - Tester Parameter - Ambient Pressure"="", "MAX - Tester Parameter - Ambient Temperature"="", "MAX - Tester Parameter - Ambient Humidity"="", "MAX - Calculated Parameter - DDM Pressure Corrected"="", "MAX - Calculated Parameter - DDM Real Power"="", "MAX - Calculated Parameter - Delta V"="", "MAX - Calculated Parameter - Flowrate"="", "MAX - Calculated Parameter - Airwatt"="", "MAX_FISF_Check_Average_Delta_Tmag"="", "MAX - FISF - BEMF Finetune Result"="", "MAX tune - Delta P1"="", "MAX tune - Calculated Parameter - Airwatt"="", "Calculate Delta Airwatts - MAX finetune - Delta P2"="", "MAX finetune - DDM Parameter - Voltage"="", "MAX finetune - DDM Parameter - Current"="", "MAX finetune - DDM Parameter - Power"="", "MAX finetune - DDM Parameter - Measured Power"="", "MAX finetune - DDM Parameter - Speed"="", "MAX finetune - DDM Parameter - Pressure"="", "MAX finetune - Tester Parameter - Voltage"="", "MAX finetune - Tester Parameter - Current"="", "MAX finetune - Tester Parameter - Power"="", "MAX finetune - Tester Parameter - Ambient Pressure"="", "MAX finetune - Tester Parameter - Ambient Temperature"="", "MAX finetune - Tester Parameter - Ambient Humidity"="", "MAX finetune - Calculated Parameter - DDM Pressure Corrected"="", "MAX finetune - Calculated Parameter - DDM Real Power"="", "MAX finetune - Calculated Parameter - Delta V"="", "MAX finetune - Calculated Parameter - Flowrate"="", "MAX finetune - Calculated Parameter - Airwatt"="", "Check Derate Result"="", "Delta Tmag FISF"="", "Get Hot BEMF Result"="", "Calculate delta Pressure"="", "Finalise Calibration"="", "Calculate & Check Delta BEMF"="", "Delta P Airwatts Value"=""}, "LL"={"DDM Ambient Temp"="", "Restriction Plate Diameter"="", "LL - DDM Parameter - Voltage"="", "LL - DDM Parameter - Current"="", "LL - DDM Parameter - Power"="", "LL - DDM Parameter - Measured Power"="", "LL - DDM Parameter - Speed"="", "LL - DDM Parameter - Pressure"="", "LL - Tester Parameter - Voltage"="", "LL - Tester Parameter - Current"="", "LL - Tester Parameter - Power"="", "LL - DDM Real Power"="", "LL - Calibrate Task Detect LL"=""}, "HL"={"HL - DDM Parameter - Voltage"="", "HL - DDM Parameter - Current"="", "HL - DDM Parameter - Power"="", "HL - DDM Parameter - Measured Power"="", "HL - DDM Parameter - Speed"="", "HL - DDM Parameter - Pressure"="", "HL - Tester Parameter - Voltage"="", "HL - Tester Parameter - Current"="", "HL - Tester Parameter - Power"="", "HL - DDM Real Power"="", "HL - Calibrate Task Detect HL"=""}, "LH"={"Restriction Plate Diameter"="", "LH - DDM Parameter - Voltage"="", "LH - DDM Parameter - Current"="", "LH - DDM Parameter - Power"="", "LH - DDM Parameter - Measured Power"="", "LH - DDM Parameter - Speed"="", "LH - DDM Parameter - Pressure"="", "LH - Tester Parameter - Voltage"="", "LH - Tester Parameter - Current"="", "LH - Tester Parameter - Power"="", "LH - DDM Real Power"="", "LH - Calibrate Task Detect LH"=""}, "HH"={"HH - DDM Parameter - Voltage"="", "HH - DDM Parameter - Current"="", "HH - DDM Parameter - Power"="", "HH - DDM Parameter - Measured Power"="", "HH - DDM Parameter - Speed"="", "HH - DDM Parameter - Pressure"="", "HH - Tester Parameter - Voltage"="", "HH - Tester Parameter - Current"="", "HH - Tester Parameter - Power"="", "HH - DDM Real Power"="", "HH - Calibrate Task Detect HH"=""}, "Inlet Blockage Calibration"={"Inlet Blockage Calibration - DDM Parameter - Voltage"="", "Inlet Blockage Calibration - DDM Parameter - Current"="", "Inlet Blockage Calibration - DDM Parameter - Power"="", "Inlet Blockage Calibration - DDM Parameter - Measured Power"="", "Inlet Blockage Calibration - DDM Parameter - Speed"="", "Inlet Blockage Calibration - DDM Parameter - Pressure"="", "Inlet Blockage Calibration - Tester Parameter - Voltage"="", "Inlet Blockage Calibration - Tester Parameter - Current"="", "Inlet Blockage Calibration - Tester Parameter - Power"="", "Inlet Blockage Calibration - DDM Real Power"="", "Calibration Inlet Blockage_E"="", "Finalise Calibration"="", "Get Task Detect LL"="", "Get Task Detect HL"="", "Get Task Detect LH"="", "Get Task Detect HH"="", "Calibration Inlet Blockage"="", "Calibration eol cold bemf temp"=""}, "GOOD"={"GOOD UNIT - Clear EEPROM Error Log"="", "GOOD UNIT - Write Product Timestamp - Mode"="", "GOOD UNIT - Write Product Timestamp - Timestamp"="", "GOOD UNIT - Write Product Timestamp - Rig ID"="", "GOOD UNIT - Write Product Timestamp - Passmark ID"="", "GOOD UNIT - Write Product Timestamp - Passmark Rev"="", "GOOD UNIT - Set Device Mode to PROD"="", "GOOD UNIT - Backup PCBA Calibration EEPROM Response"="", "GOOD UNIT - Check Security Bit"="", "GOOD UNIT - Set Calibration Lock"="", "GOOD UNIT - Get_Calibration_Lock"="", "GOOD UNIT - Disconnect UUT"=""}, "NG"={"NG UNIT - Read NVM Error"="", "NG UNIT - Set Device Mode to FCT"="", "NG UNIT - Backup PCBA Calibration EEPROM Response - CAL"="", "NG UNIT - Backup PCBA Calibration EEPROM Response - ERROR"="", "NG UNIT - Backup PCBA Calibration EEPROM Response - USAGE"="", "NG UNIT - Disconnect UUT"=""}, "SN"="", "Table"=[], "Count"={"Total"=0, "OK"=0, "NG"=0, "Yield"=0.0}, "Start Time"=timestamp(0 s since 1904-01-01), "daemon reference"=refnum, "CT"=0.0, "Config"=[], "OK/NG"=FALSE, "Station ID"="", "MES DDM SN"="", "MES PCBA SN"="", "Retest"="", "Lux"="", "Initialisation_Status"={"LMT - Connect UUT (con COM)"="", "LMT - Software Version (rrel)"="", "LMT - Write SKU file (wskuc)"="", "LMT - SKU file name"="", "Connect UUT DDM"="", "Read DDM EOL Timestamp - Mode"="", "Read DDM EOL Timestamp - Timestamp"="", "Read DDM EOL Timestamp - Rig ID"="", "Read DDM EOL Timestamp - Passmark ID"="", "Read DDM EOL Timestamp - Passmark Rev"="", "Software Version before flashing"="", "Read Hardware Serial"="", "UUT DDM SN"="", "Compare DDM SN with MES SN"="", "Backup PCBA Calibration EEPROM Response - CAL"="", "Flash Firmware Version"="", "Check SW Version"="", "Read DDM SW Version after flashing"="", "Set SKU Config"="", "Ready Status"="", "Set Device Mode to EOL"="", "DDM Parameter - Voltage"="", "DDM Parameter - Current"="", "DDM Parameter - Power"="", "DDM Parameter - Speed"="", "DDM Parameter - Pressure"="", "Tester Parameter - Voltage"="", "Tester Parameter - Current"="", "Tester Parameter - Power"="", "Tester Parameter - Ambient Pressure"="", "Tester Parameter - Ambient Temperature"="", "Calculated Parameter - DDM Pressure Corrected"="", "Calculated Parameter - DDM Real Power"="", "Calculated Parameter - Delta V"=""}, "BEMF_Calibration_Status"={"Calibration Result - eol_cold_bemf_temp"="", "DDM Ambient Temp"="", "Restriction Plate Diameter"="", "Calibration Result - eol_bemf_mp_cold_coef_a"="", "Calibration Result - eol_bemf_mp_cold_coef_b"="", "Calibration Result - eol_bemf_mp_cold_coef_c"="", "Calibration Result - eol_bemf_lsi_cold_ref_coeffs"="", "Get - Calibration Result - eol_bemf_lsi_speed"="", "Get - Calibration Result - eol_bemf_lsi_integral_0"="", "Calibration Result - eol_bemf_lsi_integral_1"="", "Get - Calibration Result - eol_bemf_lsi_integral_2"="", "Get - Calibration Result - eol_cold_bemf"="", "Get - Calibration Result - eol_cold_bemf_fisf"="", "Finalise Calibration"="", "Compare -Calibration Result - eol_cold_bemf"="", "Compare -Calibration Result - eol_cold_bemf_fisf"=""}, "ECO_Status"={"Reset Power Tune"="", "Reset BEMF FISF Calibration"="", "Restriction Plate Diameter"="", "ECO - Stabilisation Time"="", "ECO - DDM Parameter - Voltage"="", "ECO - DDM Parameter - Current"="", "ECO - DDM Parameter - Power"="", "ECO - DDM Parameter - Measured Power"="", "ECO - DDM Parameter - Speed"="", "ECO - DDM Parameter - Pressure"="", "ECO - Tester Parameter - Voltage"="", "ECO - Tester Parameter - Current"="", "ECO - Tester Parameter - Power"="", "ECO - Tester Parameter - Ambient Pressure"="", "ECO - Tester Parameter - Ambient Temperature"="", "ECO - Tester Parameter - Ambient Humidity"="", "ECO - Calculated Parameter - DDM Pressure Corrected"="", "ECO - Calculated Parameter - DDM Real Power"="", "ECO - Calculated Parameter - Delta V"="", "ECO - Calculated Parameter - Flowrate"="", "ECO - Calculated Parameter - Airwatt"="", "ECO - Formula"="", "PT ECO - Power Tune Mode Status"=""}, "BOOST_Status"={"Restriction Plate Diameter"="", "BOOST - Stabilisation Time"="", "BOOST - DDM Parameter - Voltage"="", "BOOST - DDM Parameter - Current"="", "BOOST - DDM Parameter - Power"="", "BOOST - DDM Parameter - Measured Power"="", "BOOST - DDM Parameter - Speed"="", "BOOST - DDM Parameter - Pressure"="", "BOOST - Tester Parameter - Voltage"="", "BOOST - Tester Parameter - Current"="", "BOOST - Tester Parameter - Power"="", "BOOST - Tester Parameter - Ambient Pressure"="", "BOOST - Tester Parameter - Ambient Temperature"="", "BOOST - Tester Parameter - Ambient Humidity"="", "BOOST - Calculated Parameter - DDM Pressure Corrected"="", "BOOST - Calculated Parameter - DDM Real Power"="", "BOOST - Calculated Parameter - Delta V"="", "BOOST - Calculated Parameter - Flowrate"="", "BOOST - Calculated Parameter - Airwatt"="", "BOOST - Get AM Presence"="", "Air Muscle Turn Off Status"="", "BOOST - Air Muscle Calculated Parameter - Airwatt B"="", "BOOST - Air Muscle Calculate Airwatt Delta"="", "PT BOOST - Power Tune Mode Status"="", "Finalise Calibration"="", "ECO - Get AW Calibration value"="", "BOOST - Get AW Calibration value"=""}, "MAX_Status"={"Restriction Plate Diameter"="", "MAX - Stabilisation Time"="", "Get Average Delta Tmag (LSIdelta_FISFdelta_LSItmag_FISFtmag_IIRtmag)"="", "Get Average Delta Tmag FISF"="", "MAX - DDM Parameter - Voltage"="", "MAX - DDM Parameter - Current"="", "MAX - DDM Parameter - Power"="", "MAX - DDM Parameter - Measured Power"="", "MAX - DDM Parameter - Speed"="", "MAX - DDM Parameter - Pressure"="", "MAX - Tester Parameter - Voltage"="", "MAX - Tester Parameter - Current"="", "MAX - Tester Parameter - Power"="", "MAX - Tester Parameter - Ambient Pressure"="", "MAX - Tester Parameter - Ambient Temperature"="", "MAX - Tester Parameter - Ambient Humidity"="", "MAX - Calculated Parameter - DDM Pressure Corrected"="", "MAX - Calculated Parameter - DDM Real Power"="", "MAX - Calculated Parameter - Delta V"="", "MAX - Calculated Parameter - Flowrate"="", "MAX - Calculated Parameter - Airwatt"="", "MAX_FISF_Check_Average_Delta_Tmag"="", "MAX - FISF - BEMF Finetune Result"="", "MAX tune - Delta P1"="", "MAX tune - Calculated Parameter - Airwatt"="", "Calculate Delta Airwatts - MAX finetune - Delta P2"="", "MAX finetune - DDM Parameter - Voltage"="", "MAX finetune - DDM Parameter - Current"="", "MAX finetune - DDM Parameter - Power"="", "MAX finetune - DDM Parameter - Measured Power"="", "MAX finetune - DDM Parameter - Speed"="", "MAX finetune - DDM Parameter - Pressure"="", "MAX finetune - Tester Parameter - Voltage"="", "MAX finetune - Tester Parameter - Current"="", "MAX finetune - Tester Parameter - Power"="", "MAX finetune - Tester Parameter - Ambient Pressure"="", "MAX finetune - Tester Parameter - Ambient Temperature"="", "MAX finetune - Tester Parameter - Ambient Humidity"="", "MAX finetune - Calculated Parameter - DDM Pressure Corrected"="", "MAX finetune - Calculated Parameter - DDM Real Power"="", "MAX finetune - Calculated Parameter - Delta V"="", "MAX finetune - Calculated Parameter - Flowrate"="", "MAX finetune - Calculated Parameter - Airwatt"="", "Check Derate Result"="", "Delta Tmag FISF"="", "Get Hot BEMF Result"="", "Calculate delta Pressure"="", "Finalise Calibration"="", "Calculate & Check Delta BEMF"="", "Delta P Airwatts Value"=""}, "LL_Status"={"DDM Ambient Temp"="", "Restriction Plate Diameter"="", "LL - DDM Parameter - Voltage"="", "LL - DDM Parameter - Current"="", "LL - DDM Parameter - Power"="", "LL - DDM Parameter - Measured Power"="", "LL - DDM Parameter - Speed"="", "LL - DDM Parameter - Pressure"="", "LL - Tester Parameter - Voltage"="", "LL - Tester Parameter - Current"="", "LL - Tester Parameter - Power"="", "LL - DDM Real Power"="", "LL - Calibrate Task Detect LL"=""}, "HL_Status"={"HL - DDM Parameter - Voltage"="", "HL - DDM Parameter - Current"="", "HL - DDM Parameter - Power"="", "HL - DDM Parameter - Measured Power"="", "HL - DDM Parameter - Speed"="", "HL - DDM Parameter - Pressure"="", "HL - Tester Parameter - Voltage"="", "HL - Tester Parameter - Current"="", "HL - Tester Parameter - Power"="", "HL - DDM Real Power"="", "HL - Calibrate Task Detect HL"=""}, "LH_Status"={"Restriction Plate Diameter"="", "LH - DDM Parameter - Voltage"="", "LH - DDM Parameter - Current"="", "LH - DDM Parameter - Power"="", "LH - DDM Parameter - Measured Power"="", "LH - DDM Parameter - Speed"="", "LH - DDM Parameter - Pressure"="", "LH - Tester Parameter - Voltage"="", "LH - Tester Parameter - Current"="", "LH - Tester Parameter - Power"="", "LH - DDM Real Power"="", "LH - Calibrate Task Detect LH"=""}, "HH_Status"={"HH - DDM Parameter - Voltage"="", "HH - DDM Parameter - Current"="", "HH - DDM Parameter - Power"="", "HH - DDM Parameter - Measured Power"="", "HH - DDM Parameter - Speed"="", "HH - DDM Parameter - Pressure"="", "HH - Tester Parameter - Voltage"="", "HH - Tester Parameter - Current"="", "HH - Tester Parameter - Power"="", "HH - DDM Real Power"="", "HH - Calibrate Task Detect HH"=""}, "Inlet Blockage Calibration_Status"={"Inlet Blockage Calibration - DDM Parameter - Voltage"="", "Inlet Blockage Calibration - DDM Parameter - Current"="", "Inlet Blockage Calibration - DDM Parameter - Power"="", "Inlet Blockage Calibration - DDM Parameter - Measured Power"="", "Inlet Blockage Calibration - DDM Parameter - Speed"="", "Inlet Blockage Calibration - DDM Parameter - Pressure"="", "Inlet Blockage Calibration - Tester Parameter - Voltage"="", "Inlet Blockage Calibration - Tester Parameter - Current"="", "Inlet Blockage Calibration - Tester Parameter - Power"="", "Inlet Blockage Calibration - DDM Real Power"="", "Calibration Inlet Blockage_E"="", "Finalise Calibration"="", "Get Task Detect LL"="", "Get Task Detect HL"="", "Get Task Detect LH"="", "Get Task Detect HH"="", "Calibration Inlet Blockage"="", "Calibration eol cold bemf temp"=""}, "GOOD_Status"={"GOOD UNIT - Clear EEPROM Error Log"="", "GOOD UNIT - Write Product Timestamp - Mode"="", "GOOD UNIT - Write Product Timestamp - Timestamp"="", "GOOD UNIT - Write Product Timestamp - Rig ID"="", "GOOD UNIT - Write Product Timestamp - Passmark ID"="", "GOOD UNIT - Write Product Timestamp - Passmark Rev"="", "GOOD UNIT - Set Device Mode to PROD"="", "GOOD UNIT - Backup PCBA Calibration EEPROM Response"="", "GOOD UNIT - Check Security Bit"="", "GOOD UNIT - Set Calibration Lock"="", "GOOD UNIT - Get_Calibration_Lock"="", "GOOD UNIT - Disconnect UUT"=""}, "NG_Status"={"NG UNIT - Read NVM Error"="", "NG UNIT - Set Device Mode to FCT"="", "NG UNIT - Backup PCBA Calibration EEPROM Response - CAL"="", "NG UNIT - Backup PCBA Calibration EEPROM Response - ERROR"="", "NG UNIT - Backup PCBA Calibration EEPROM Response - USAGE"="", "NG UNIT - Disconnect UUT"=""}, "SKU"="", "Plate_Diameter"="", "Alarm"=""} ("Data in")) -> (value=w1537:T3)  [unwired: 1 in, 1 out]
        n239 = call "Csv_fill_null.vi"("Data in"=w1537) -> ("Data out"=w1536:T3)  [unwired: 10 in]
        n240 = call "Data_Save.vi"("AllControls In"=w1539, "Data in"=w1536) -> ()  [unwired: 10 in]
      }
    }
    n241 = call "Exit.vi"("Step"=enum16{"Initial", "Write", "Read"}."Read" ("step")) -> ("Exit Out"=w1533:bool)  [unwired: 9 in, 1 out]
    n242 = call "Stop.vi"("Step"=enum16{"Initial", "Write", "Read"}."Read") -> ("Stop Out"=w1532:bool)  [unwired: 9 in, 1 out]
    n243 = Compound Arithmetic op=OR(w1533, w1532) -> (w1531:bool)
  }
  n244 = Release Queue(queue=w4) -> ()  [unwired: 2 in, 3 out]
  n245 = Unbundle By Name(w9) -> ("daemon reference"=w13:refnum<k5>)
  n246 = Release Queue(queue=w6, error in (no error)=w5) -> ()  [unwired: 1 in, 3 out]
  n247 = call "daemon disconnect.vi"("daemon reference in"=w13) -> ("error out"=w12:errorcluster)  [unwired: 10 in]
  n248 = call <vilib>:"Clear Errors.vi"("error in (no error)"=w12) -> ()  [unwired: 5 in, 2 out]
